vi "TLB Native Dynamic Events ver 0.17e.vi"() -> ()   [LabVIEW 2018]
uses:
  Labview Training Phase 2/Enum Controls/States for Action Engine.ctl
  TLB Type Definitions/State Type Definitions, for 0.26g versions and later 2.ctl
  TLB Type Definitions/Intruction Type Definitions.ctl
  TLB Type Definitions/Encoder cluster.ctl
  TLB Type Definitions/PING CLUSTER.ctl
  <vilib>/Studica/Studica Toolkit/NavX/NavX.lvlib
  <vilib>/Studica/Studica Toolkit/Background/DIO Channel.ctl
  Underlying VI's/NavX VI/navX type def.ctl
  <vilib>/Studica/Studica Toolkit/Background/I2C Channel.ctl
  TLB Type Definitions/Vision cluster.ctl
  <vilib>/NI_Real-Time Target Support.lvlib
  TLB Type Definitions/Stepper cluster.ctl
  Experimental VI's/Archived VI's/MOTOR CONTROL NO PID Type Def.ctl
  Underlying VI's/I2C Master VI/I2C MASTER Type Def.ctl
  Underlying VI's/I2C Master VI/I2C_MASTER_WRITE_NEW Type Def.ctl
  <vilib>/userdefined/High Color/IMAQdx.ctl
  Underlying VI's/I2C Master VI/Arduino_Interfacing.ctl
  TLB Type Definitions/Yaw Cluster.ctl
  TLB Type Definitions/Time cluster.ctl
  TLB Type Definitions/Y Stepper cluster.ctl
  Underlying VI's/Modified webcam FGV/Webcam AE.ctl
  Underlying VI's/Elasped Timer/Elapsed timer control.ctl
  Underlying VI's/Motor Control VI with PID/MOTOR CONTROL WITH PID AE DATA MODE TYPE DEF.ctl
  Underlying VI's/Motor Control VI with PID/MOTOR CONTROL WITH PID AE DIRECTION TYPE DEF.ctl
  TLB Type Definitions/IR Sensor Type Def.ctl
  <vilib>/myRIO/Common/Instrument Driver Framework/myRIO v1.0/AI/typedefs/AI Channels Enum.ctl
  <vilib>/myRIO/Common/Instrument Driver Framework/myRIO v1.0/AI/typedefs/AI Channels List.ctl
  <vilib>/Utility/RT CPU Load.ctl
panel:
  out "Left IR Sensor":dbl
  out "Obstacle detected":bool
  out "Speed & distance":T1
  out "Object Center Coordinates":cluster{"x":sgl, "y":sgl}
  out "Object detection cluster":T2
  out "Time up flag":bool
  out "Task selection":u8
  in  "Object recognition mode":enum16{"Ball", "Soap", "Gel", "Pipe", "None"}(ring)
  out "NavX Readings":T3
  out "Arduino Data":T4
  out "CPU loads":T5[](array[typedef]) {"ISR (%)" format="%#.2f"; "Idle (%)" format="%#.2f"; "Background (%)" format="%#.2f"; "Normal (%)" format="%#.2f"; "Above Normal (%)" format="%#.2f"; "High (%)" format="%#.2g"; "Timed Structures (%)" format="%#.2g"; "Time Critical (%)" format="%#.2g"; "Total (%)" format="%#.2g"}
  out "TASK ENABLE":bool
  out "Rising Edge":bool
  in  "Green LED":bool
  out "I2C Error":errorcluster
  out "State Logic":T6=enum."Startup"
  out "elements":T7[](array[typedef])
  in  "STOP TASK":bool
  in  "OK Button":bool
  in  "STOP":bool
  out "error out":errorcluster
  out "Action Queue Items":i32
  out "State Logic Queue Items":i32
  out "Action Queues items":string[](array[string])=["Hardware reset", "Software reset", ""]
  out "Action State":string
  # "System Health Status Update"
  # "VISION"
  # "TLB FRAMEWORK STATUS"
  # "Test Programme written by Calvin Loke    Dated: 28 Aug 2019\nTest Programme revised by Dr Alex See   Dated 30 Aug 2019\n\nRevision date: 20/03/2020\nProgramme version:   TLB Native Dynamic Events ver 0.14a"
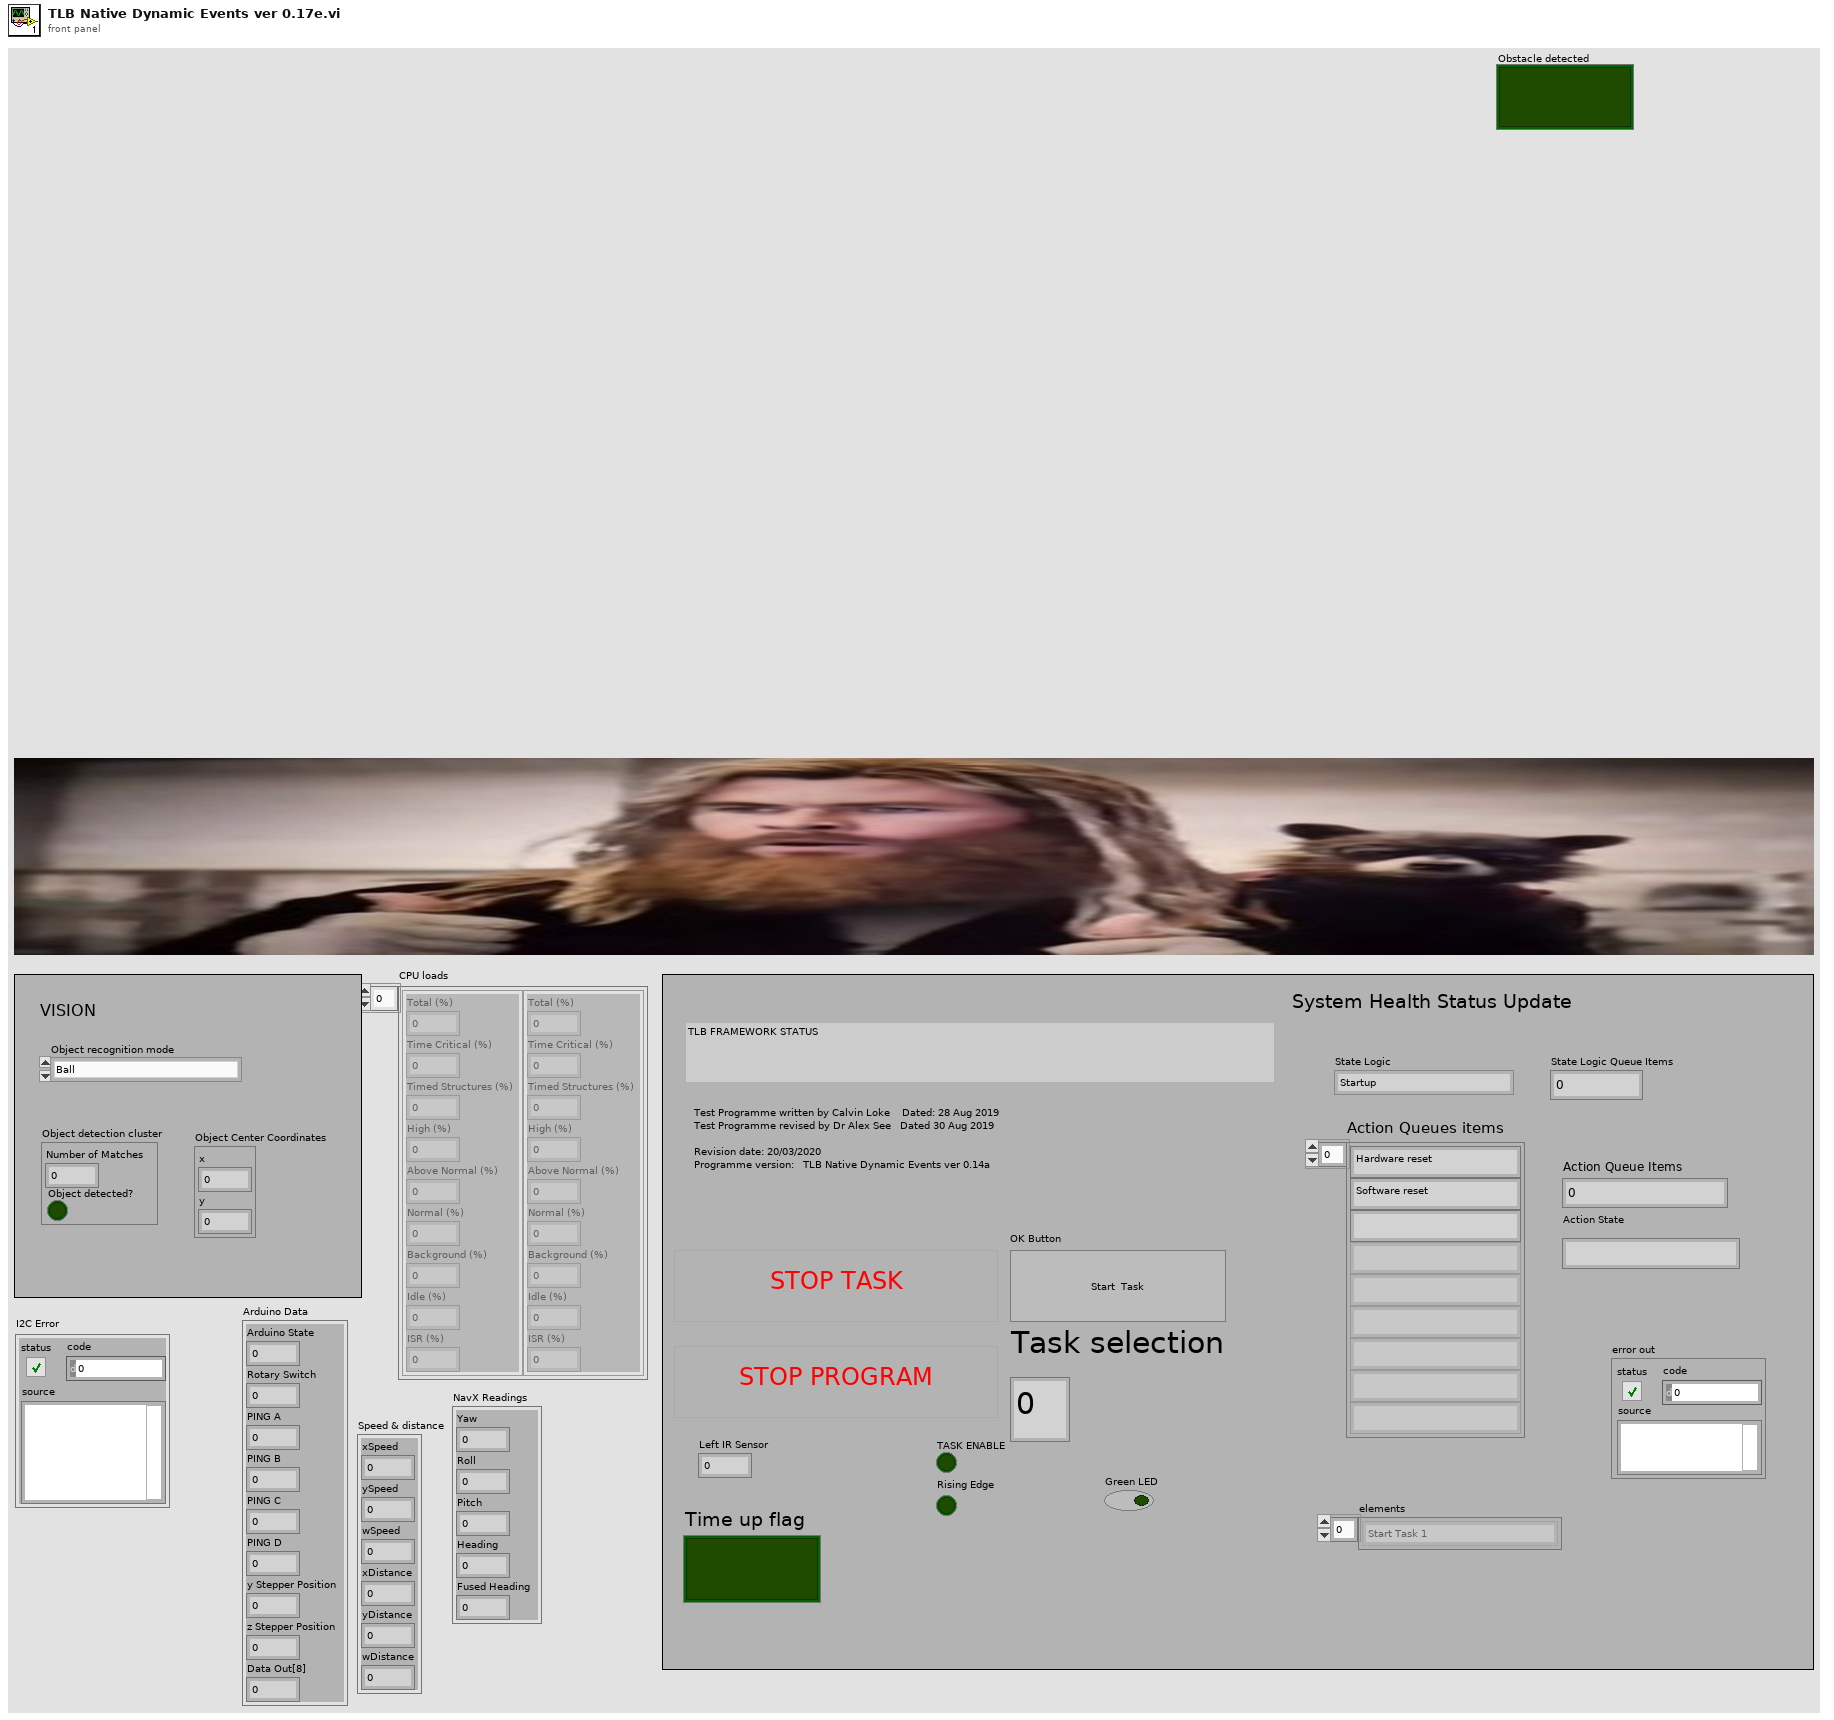
[diagram p1: front panel]
types:
  T1 = cluster{"xSpeed":dbl, "ySpeed":dbl, "wSpeed":dbl, "xDistance":dbl, "yDistance":dbl, "wDistance":dbl}
  T2 = cluster{"Number of Matches":i32, "Object detected?":bool}
  T3 = cluster{"Yaw":dbl, "Roll":dbl, "Pitch":dbl, "Heading":dbl, "Fused Heading":dbl}
  T4 = cluster{"Arduino State":u8, "Rotary Switch":u8, "PING A":u8, "PING B":u8, "PING C":u8, "PING D":u8, "y Stepper Position":u8, "z Stepper Position":u8, "Data Out[8]":u8}
  T5 = typedef "NI_Real-Time Target Support.lvlib/RT CPU Load.ctl" = cluster{"Total (%)":dbl, "Time Critical (%)":dbl, "Timed Structures (%)":dbl, "High (%)":dbl, "Above Normal (%)":dbl, "Normal (%)":dbl, "Background (%)":dbl, "Idle (%)":dbl, "ISR (%)":dbl}
  T6 = typedef "State Type Definitions, for 0.26g versions and later 2.ctl" = enum16{"None", "Startup", "Move to Angle", "True Stop", "Idle", "Shutdown", "Task 1A", "Task 1B", "Task 2:Raise Arm", "Task 2:Sensor Mode", "Task 2:Reverse Mode", "Task 3", "Task 4_A", "Task 4_B", "Task 4_C", "Task 4_D", "Task 5A", "Task 5B", "Task 5C", "Task 5D", "Task 5E: POSITION ARM", "Task 5F: ARM GRAB HEIGHT", "Task 5G: CLOSE CLAW", "Task 5H: RAISE ARM", "Task 6_A", "Task 6_B", "Task 7", "Task 8A: RAISE ARM", "Task 8B: MOVE TO BOX", "Task 8C: CAM BURST", "Task 8D: PROCESS IMAGE", "Task 8E: ROBOT ADJUST", "Task 8F: CAM BURST 2", "Task 8G: PROCESS IMAGE 2", "Task 8H: ARM ADJUST", "Task 8I: ARM GRAB HEIGHT", "Task 8J: CLOSE CLAW", "Task 8K: RAISE MY SWORD", "Task 9A: Raise Arm", "Task 9B: Rotate to Angle", "Task 9C: Detect Box", "Task 9D: MOVE FORWARD", "Task 9E: MOVE LEFT", "Task 9F: SCAN BOX", "Task 9G: MOVE RIGHT", "Task 9H: SCAN BOX 2", "Task 9I: ROTATE 90 CW", "Task 9J: FORWARD", "Task 9K: RAM WALL", "Task 9L: MOVE RIGHT", "Task 9M: SCAN BOX 3", "Task 9M: MOVE RIGHT", "Task 9N: SCAN BOX 4", "PENIS", "PENIS 2", "PENIS 3", "Task 9R: PROCESS COLOUR", "Task A1: Task 9 Open cam", "Task A2: Task 9 Move Arm", "Task A3: Task 9 Set Timer", "Task A4: Tasl 9 Capture images", "Task A5: Task 9 Close camera", "Task A6: Process Colour", "Task A7: Dispose Camera Buffer"}
  T7 = typedef "Intruction Type Definitions.ctl" = enum16{"None", "Start Task 1", "Start Task 2", "Start Task 3", "Start Task 4", "Start Task 5", "Start Task 6", "Start Task 7", "Start Task 8 - BALL", "Start Task 8 - Gel", "Start Task 8 - Pipe", "Start Task 8 - Soap", "Start Task 9", "Start Task A", "Start Task B", "Exit"}
  T8 = typedef "IR Sensor Type Def.ctl" = cluster{"Left IR Sensor":dbl, "Arm IR Sensor":dbl, "Bottom IR Sensor":dbl}
  T9 = typedef "Y Stepper cluster.ctl" = cluster{"yStepper desired":u8}
  T10 = typedef "Time cluster.ctl" = cluster{"Time up flag":bool, "SET TIME TO CHECK":dbl}
  T11 = typedef "Yaw Cluster.ctl" = cluster{"Yaw":dbl, "Compass":dbl}
  T12 = typedef "Stepper cluster.ctl" = cluster{"y Stepper Position":u8, "z Stepper Position":u8}
  T13 = typedef "DIO Channel.ctl" = enum16{"Not Connected", "A/DIO1", "A/DIO2", "A/DIO3", "A/DIO4", "A/DIO5", "A/DIO6", "A/DIO7", "A/DIO13", "B/DIO1", "B/DIO2", "B/DIO3", "B/DIO4", "B/DIO5", "B/DIO6", "B/DIO7", "B/DIO13", "C/DIO0", "C/DIO1", "C/DIO2", "C/DIO3", "C/DIO4", "C/DIO5", "C/DIO6", "C/DIO7"}
  T14 = typedef "Vision cluster.ctl" = cluster{"Recognized Object":bool, "Object X coordinate":dbl, "Object Y coordinate":dbl}
  T15 = typedef "PING CLUSTER.ctl" = cluster{"PING_A":u8, "PING_B":u8, "PING_C":u8, "PING_D":u8}
  T16 = typedef "Encoder cluster.ctl" = cluster{"xDistance":dbl, "yDistance":dbl, "wDistance":dbl}
  T17 = cluster{"DIO Channel":T13, "FPGA VI Reference Out":refnum<k20>}
  T18 = typedef "navX type def.ctl" = enum16{"Get i2C reference", "Read Values", "Zero Yaw"}
  T19 = typedef "Arduino_Interfacing.ctl" = enum16{"Initialize", "Write to Arduino", "Read From Arduino"}
  T20 = typedef "I2C Channel.ctl" = enum16{"Not Connected", "A", "B"}
  T21 = typedef "States for Action Engine.ctl" = enum16{"Initialize", "Write", "Read"}
  T22 = cluster{"I2C Ref Out":cluster{"I2C Channel":T20, "FPGA VI Reference Out":refnum<k20>}, "Connected":bool, "Slave Address (7-bit)":u8, "Registry":u8[]}
  T23 = typedef "Intruction Type Definitions.ctl" = enum16{"None", "Start Task 1", "Start Task 2", "Start Task 3", "Start Task 4", "Start Task 5", "Start Task 6", "Start Task 7", "Start Task 8", "Start Task 9", "Start Task A", "Start Task B", "Exit"}
  T24 = typedef "IMAQ Image.ctl" = refnum<image>
  T25 = typedef "State Type Definitions.ctl" = enum16{"None", "Startup", "Move to Angle", "True Stop", "Idle", "Shutdown", "Task 1", "Task 2:Raise Arm", "Task 2:Sensor Mode", "Task 2:Reverse Mode", "Task 3", "Task 4_A", "Task 4_B", "Task 4_C", "Task 4_D", "Task 5A: ARM CAM HEIGHT", "Task 5B: MOVE TO BOX", "Task 5C: CAM BURST", "Task 5D: PROCESS IMAGE", "Task 5E: POSITION ARM", "Task 5F: ARM GRAB HEIGHT", "Task 5G: CLOSE CLAW", "Task 5H: RAISE ARM", "Task 6_A", "Task 6_B", "Task 7", "Task 8A: RAISE ARM", "Task 8B: MOVE TO BOX", "Task 8C: CAM BURST", "Task 8D: PROCESS IMAGE", "Task 8E: ROBOT ADJUST", "Task 9A: Raise Arm", "Task 9B: Rotate to Angle", "Task 9C: Rotation alignmnet", "Task B"}
  T26 = typedef "MOTOR CONTROL WITH PID AE DIRECTION TYPE DEF.ctl" = enum16{"y-axis movement", "x-axis movement", "rotation", "stop", "reset encoders"}
  T27 = typedef "MOTOR CONTROL WITH PID AE DATA MODE TYPE DEF.ctl" = enum16{"Init AE", "Write to AE", "Read from AE"}
  T28 = typedef "Elapsed timer control.ctl" = enum16{"Start", "Pause", "Initialize"}
  T29 = typedef "I2C_MASTER_WRITE_NEW Type Def.ctl" = enum16{"Ultrasonic sensors", "Stepper origin", "zStepper 13.3k", "zStepper 13k", "zStepper 12k", "zStepper 11k", "zStepper 10k", "zStepper 9k", "zStepper 8k", "zStepper 7k", "zStepper 6k", "zStepper 5k", "zStepper 4k", "zStepper 3k", "zStepper 2k", "zStepper 1k", "zStepper 900", "zStepper 800", "zStepper 700", "zStepper 600", "zStepper 500", "zStepper 400", "zStepper 300", "zStepper 200", "zStepper 100", "zStepper 0", "yStepper control", "Open Claw", "Close Claw", "Soft Reset"}
  T30 = typedef "Webcam AE.ctl" = enum16{"Initialize Camera", "Open Camera", "Continuous Acquisition", "Close Camera", "Retrieve Image", "Dispose Camera Image Buffer"}
  T31 = typedef "IMAQdx.ctl" = refnum<k21>
  T32 = typedef "Webcam AE.ctl" = enum16{"Initialize Camera", "Open Camera", "Continuous Acquisition", "Close Camera", "Retrieve Image", "Dispose Image Buffers"}
  T33 = typedef "MOTOR CONTROL NO PID Type Def.ctl" = enum16{"Init", "Front Back", "Left Right", "Rotate", "Stop", "Latch"}
  T34 = typedef "AI Channels List.ctl" = T35[]
  T35 = typedef "AI Channels Enum.ctl" = enum16{"Not Connected", "AudioIn/Left", "AudioIn/Right", "C/AI0", "C/AI1", "A/AI0", "A/AI1", "A/AI2", "A/AI3", "A/AI4", "A/AI5", "A/AI6", "A/AI7", "B/AI0", "B/AI1", "B/AI2", "B/AI3", "B/AI4", "B/AI5", "B/AI6", "B/AI7", "AI/AI0", "AI/AI1", "AI/AI2", "AI/AI3", "A/AI0 (DIFF)", "A/AI1 (DIFF)", "A/AI2 (DIFF)", "A/AI3 (DIFF)", "B/AI0 (DIFF)", "B/AI1 (DIFF)", "B/AI2 (DIFF)", "B/AI3 (DIFF)"}
  T36 = typedef "I2C MASTER Type Def.ctl" = enum16{"Last State", "Mode 0", "Mode 1", "Mode 2", "Mode 3", "Mode 4", "Mode 5", "Mode 6", "Mode 7", "Mode 8", "Mode 9", "Mode 10"}
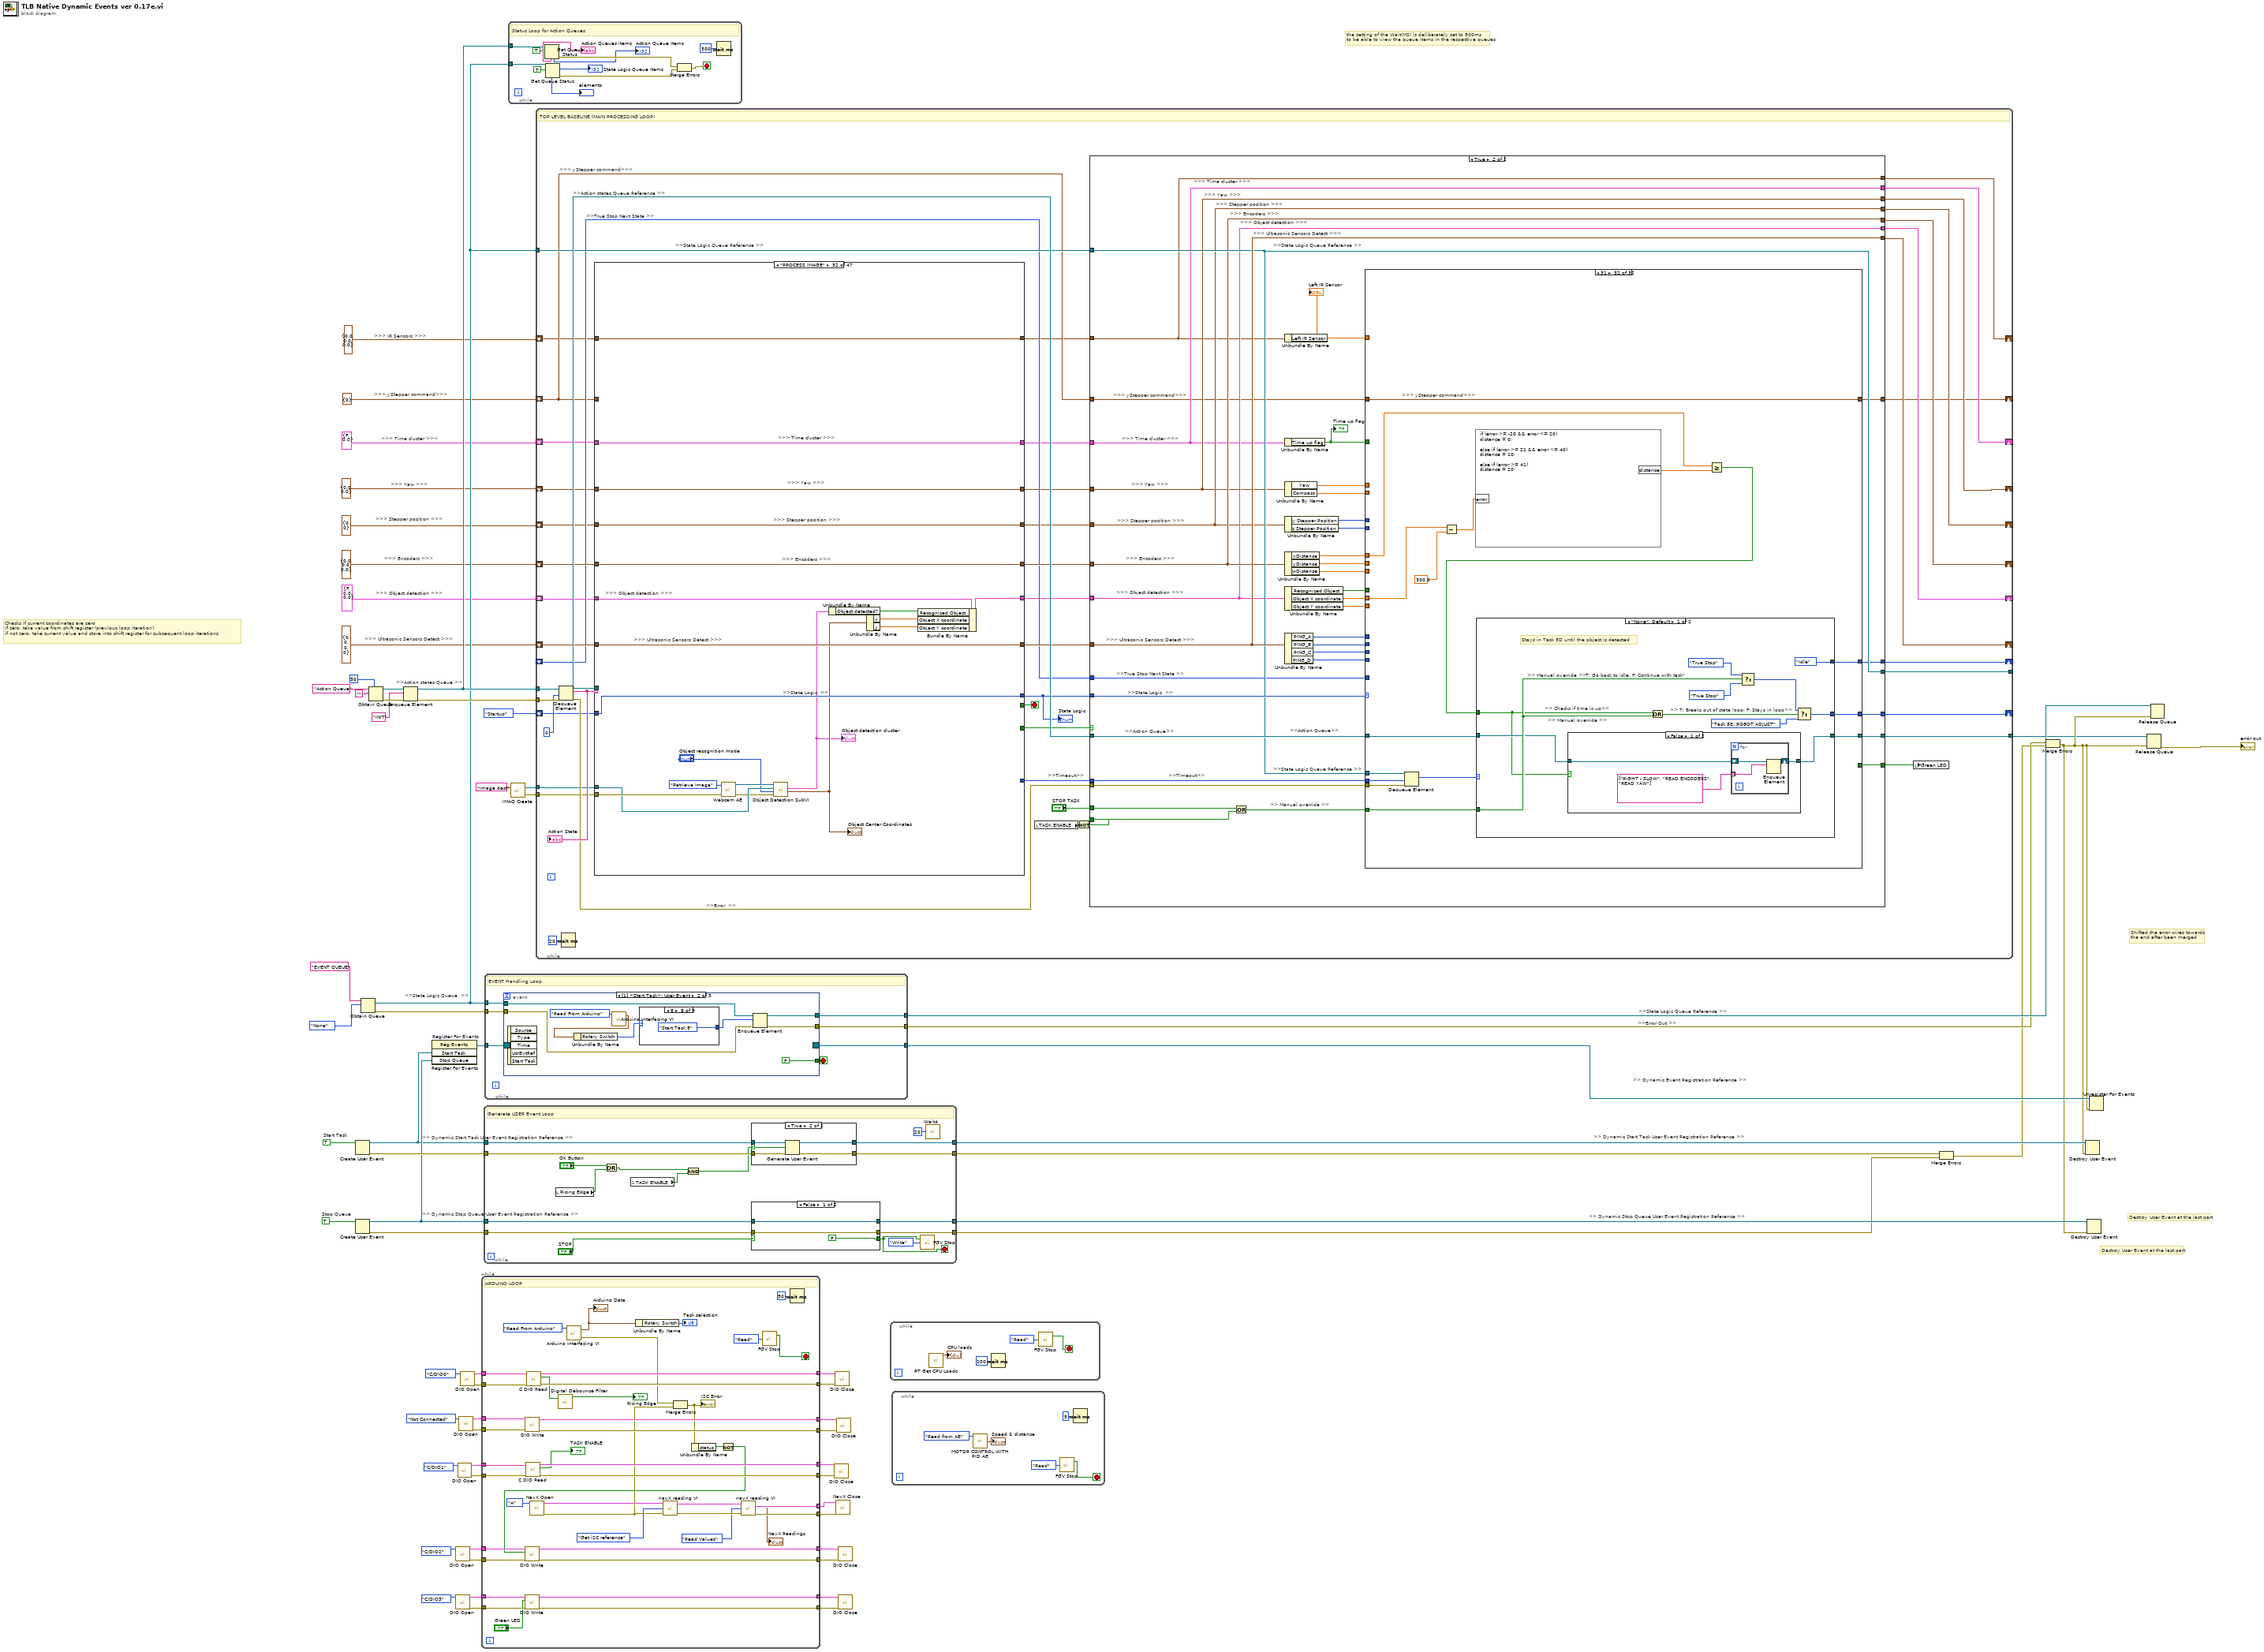
[diagram p0: block diagram]
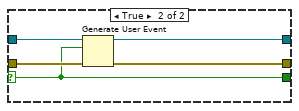
[diagram p2: hidden frame]
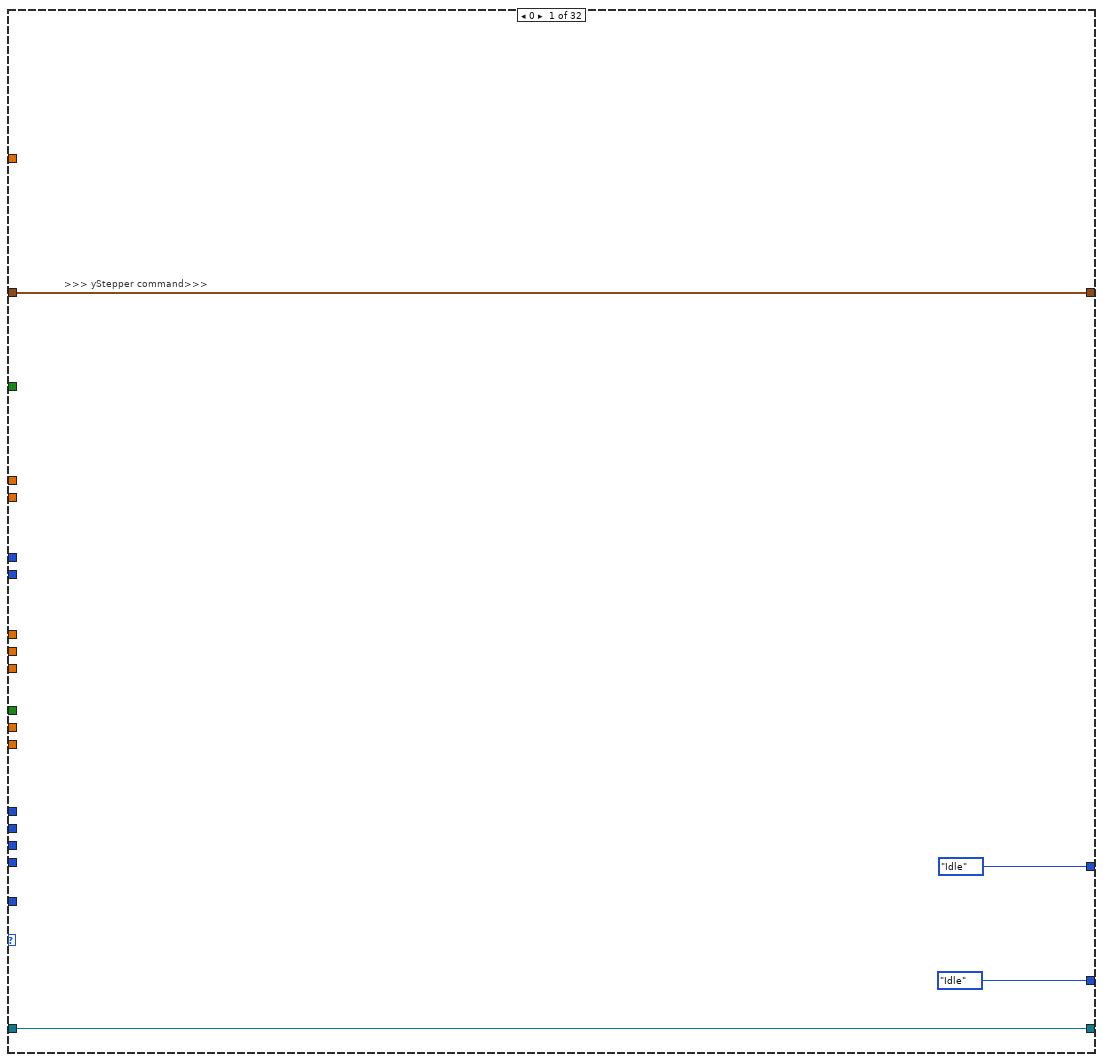
[diagram p5: hidden frame]
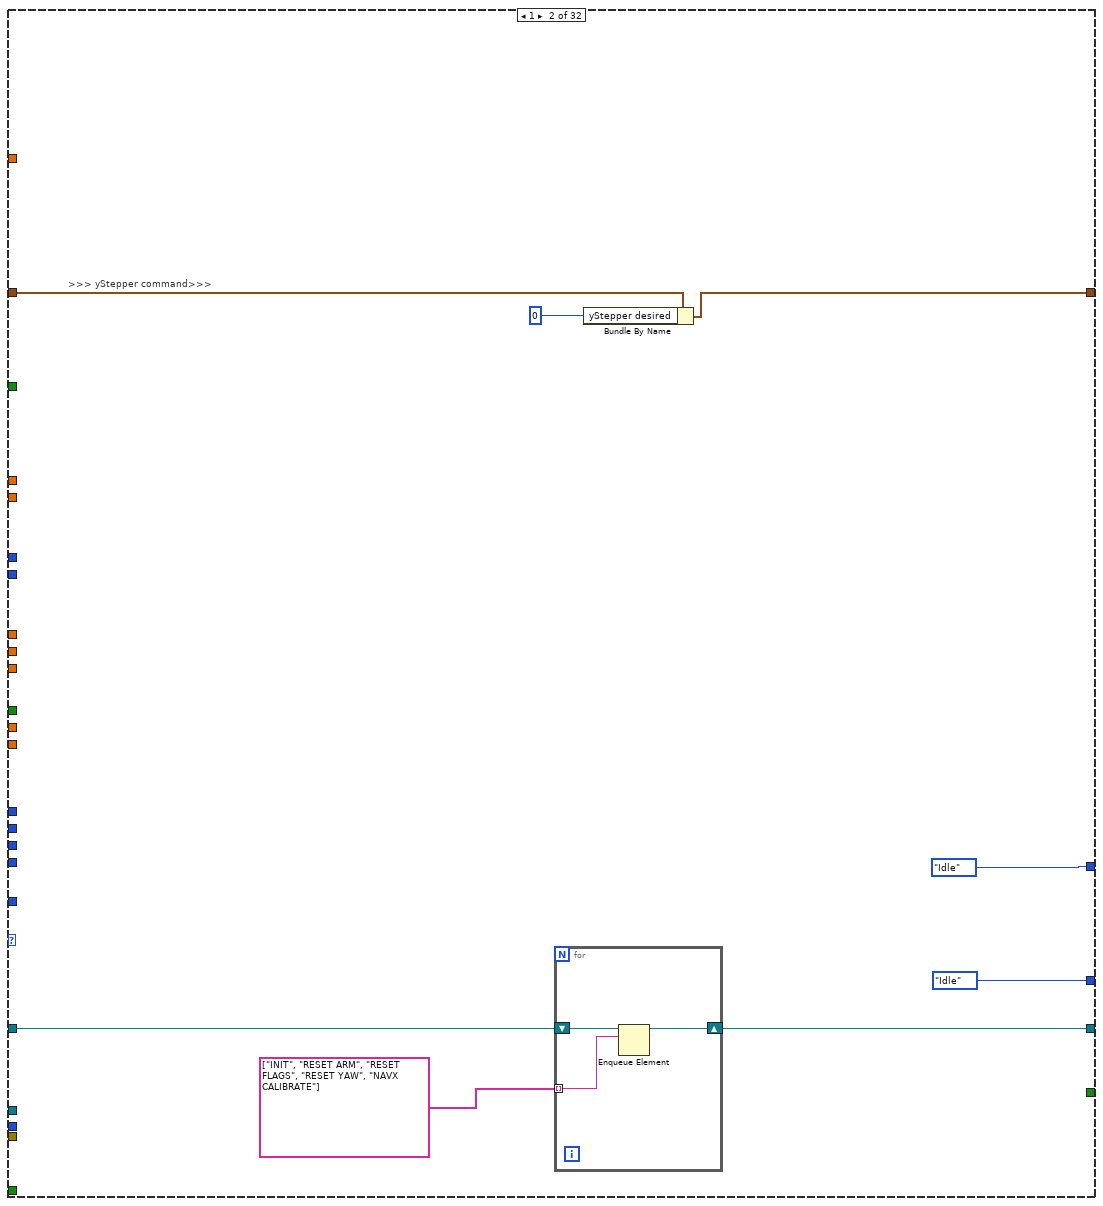
[diagram p6: hidden frame]
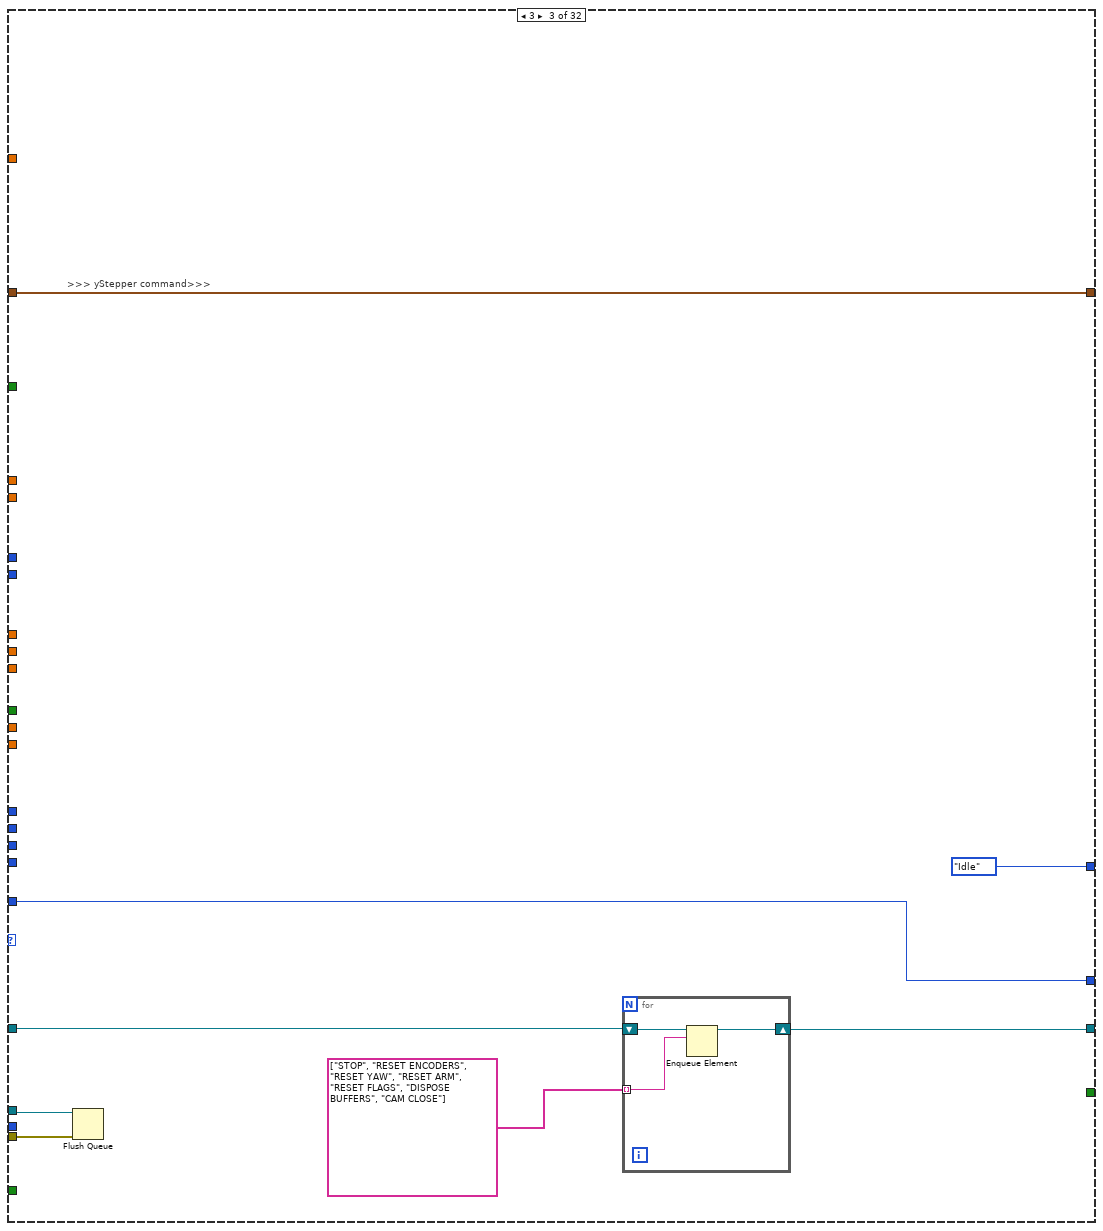
[diagram p7: hidden frame]
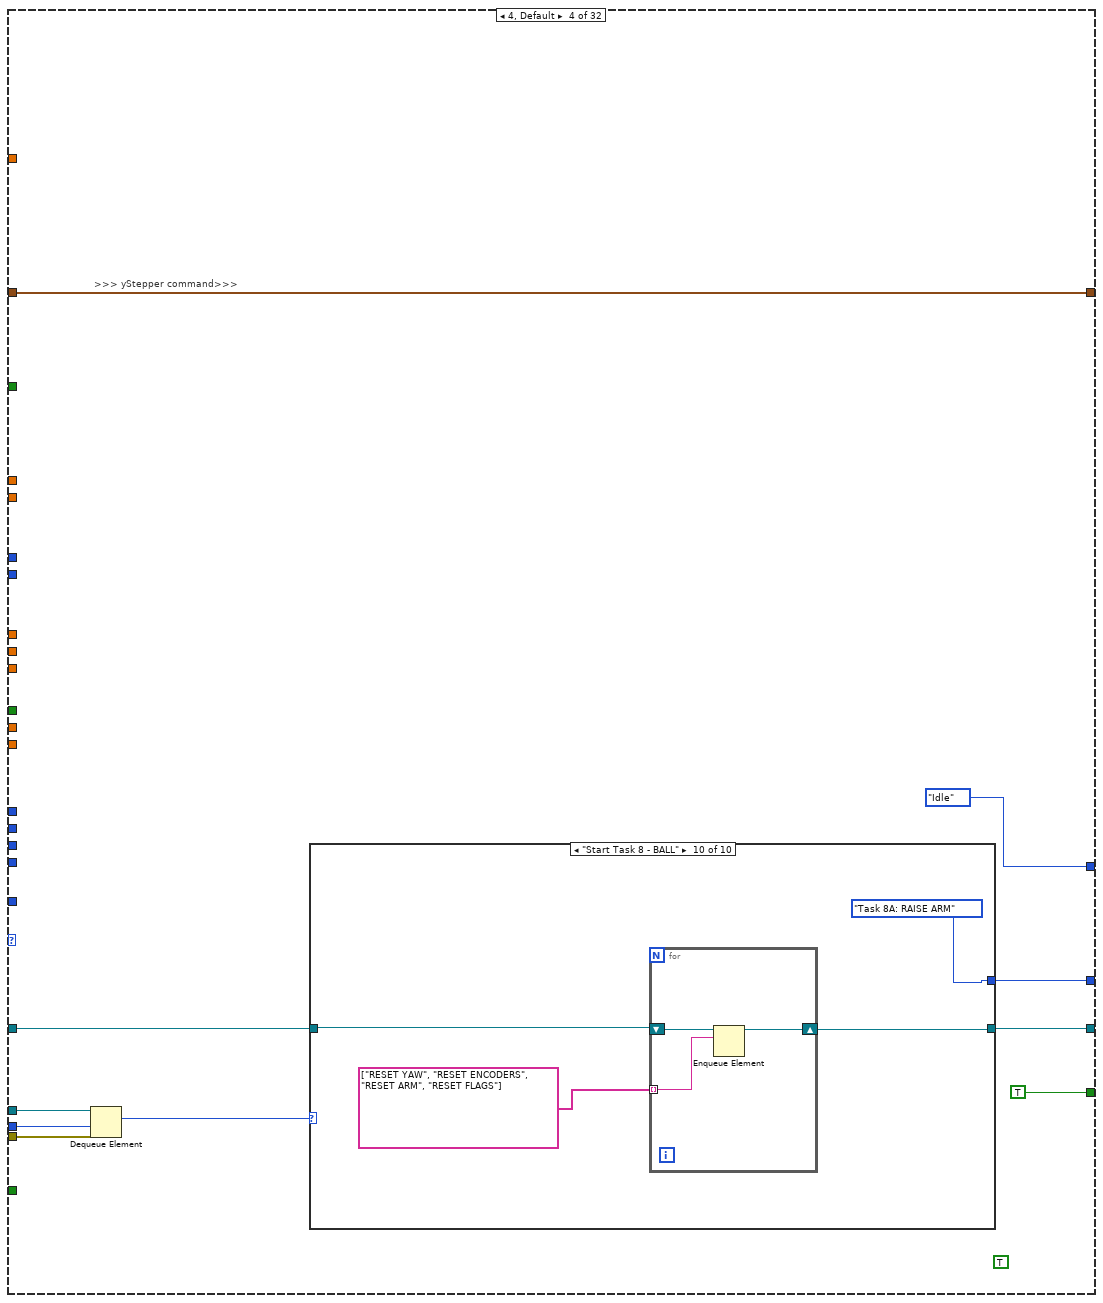
[diagram p8: hidden frame]
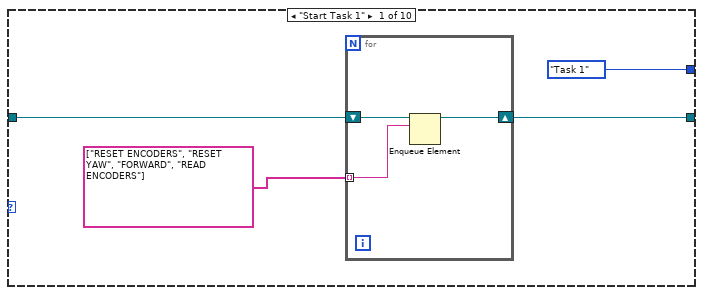
[diagram p9: hidden frame]
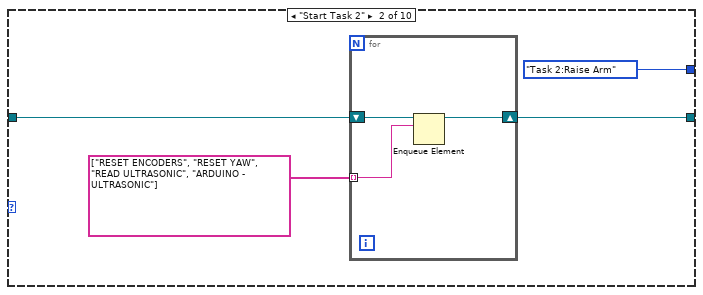
[diagram p10: hidden frame]
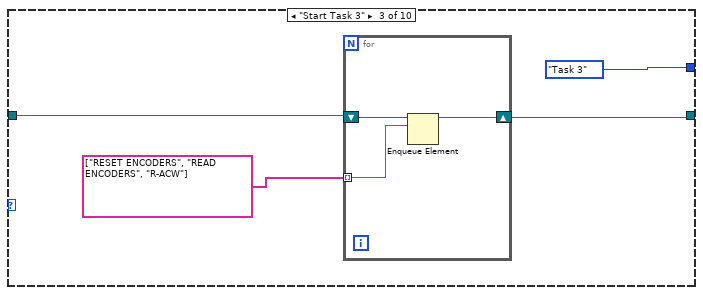
[diagram p11: hidden frame]
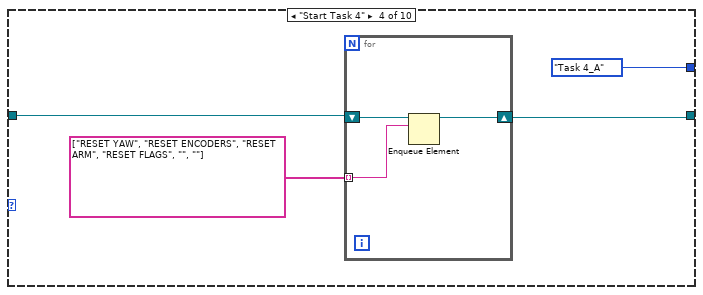
[diagram p12: hidden frame]
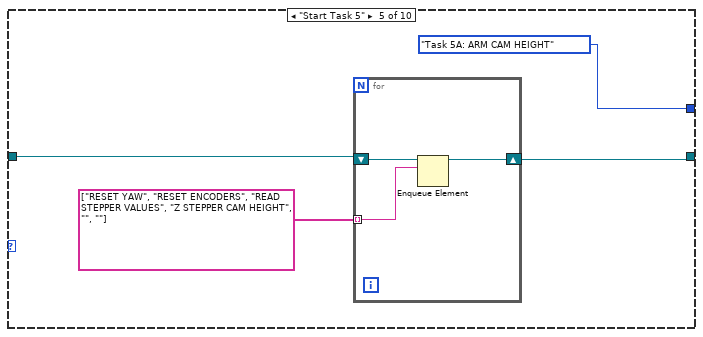
[diagram p13: hidden frame]
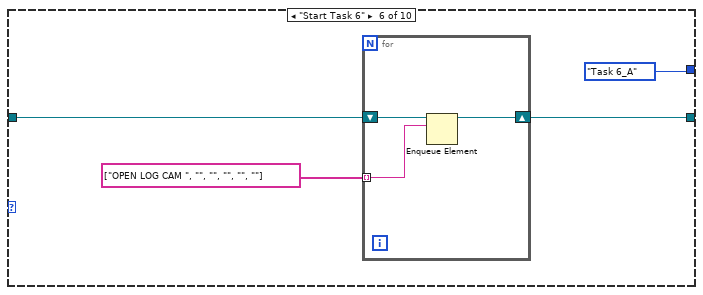
[diagram p14: hidden frame]
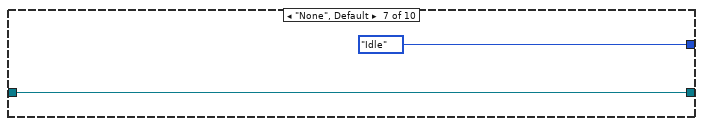
[diagram p15: hidden frame]
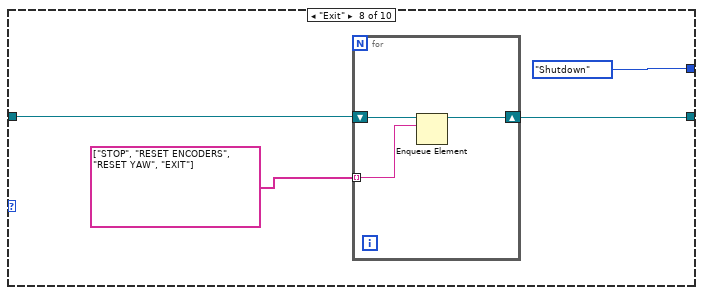
[diagram p16: hidden frame]
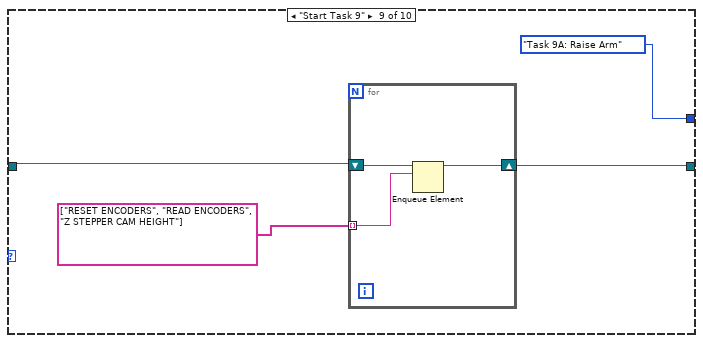
[diagram p17: hidden frame]
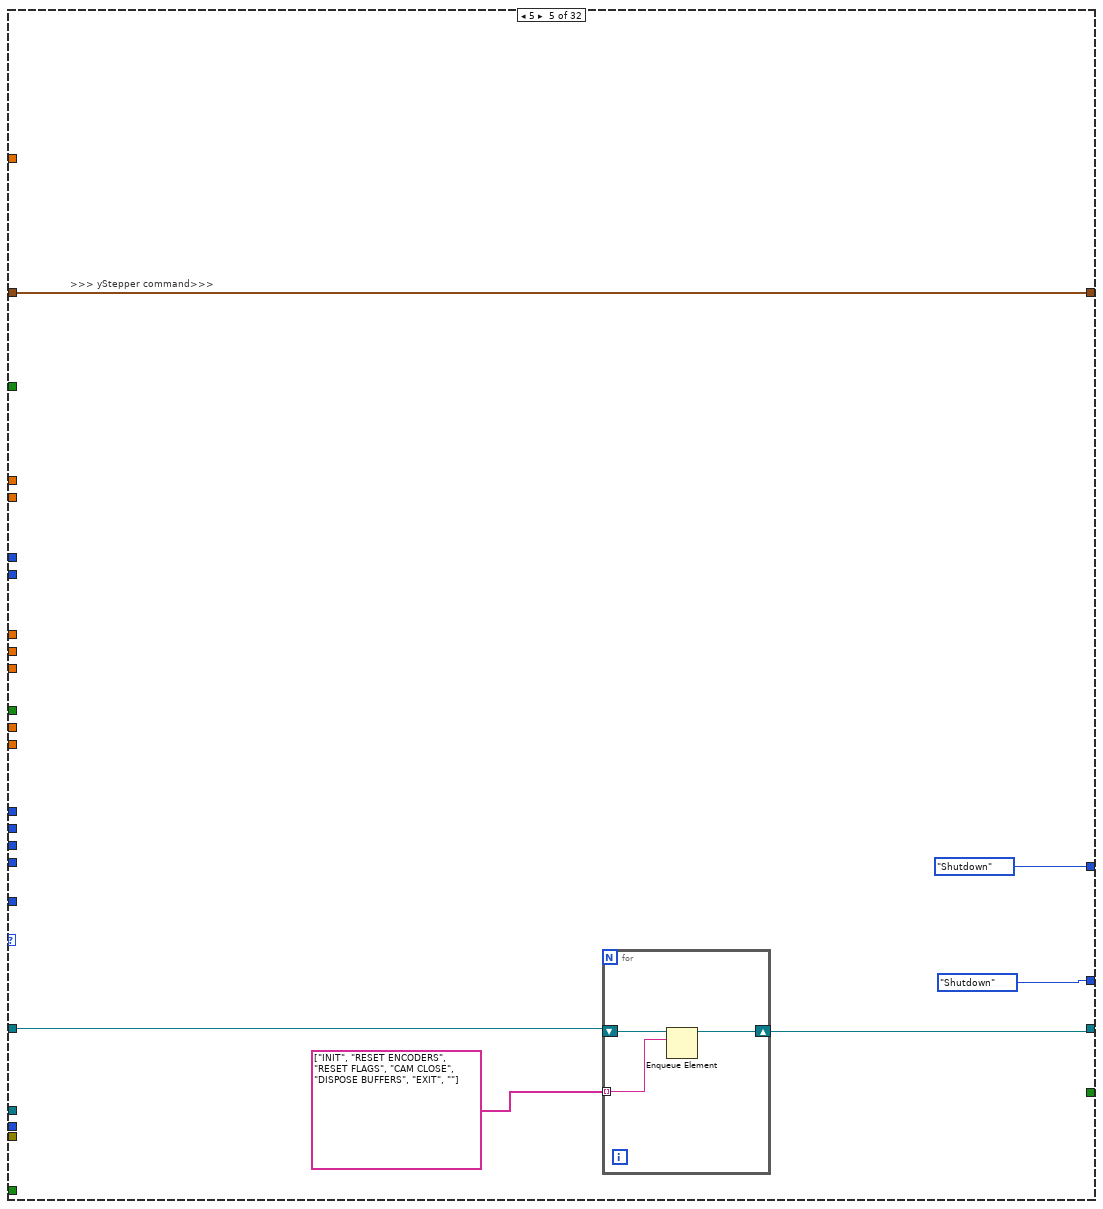
[diagram p18: hidden frame]
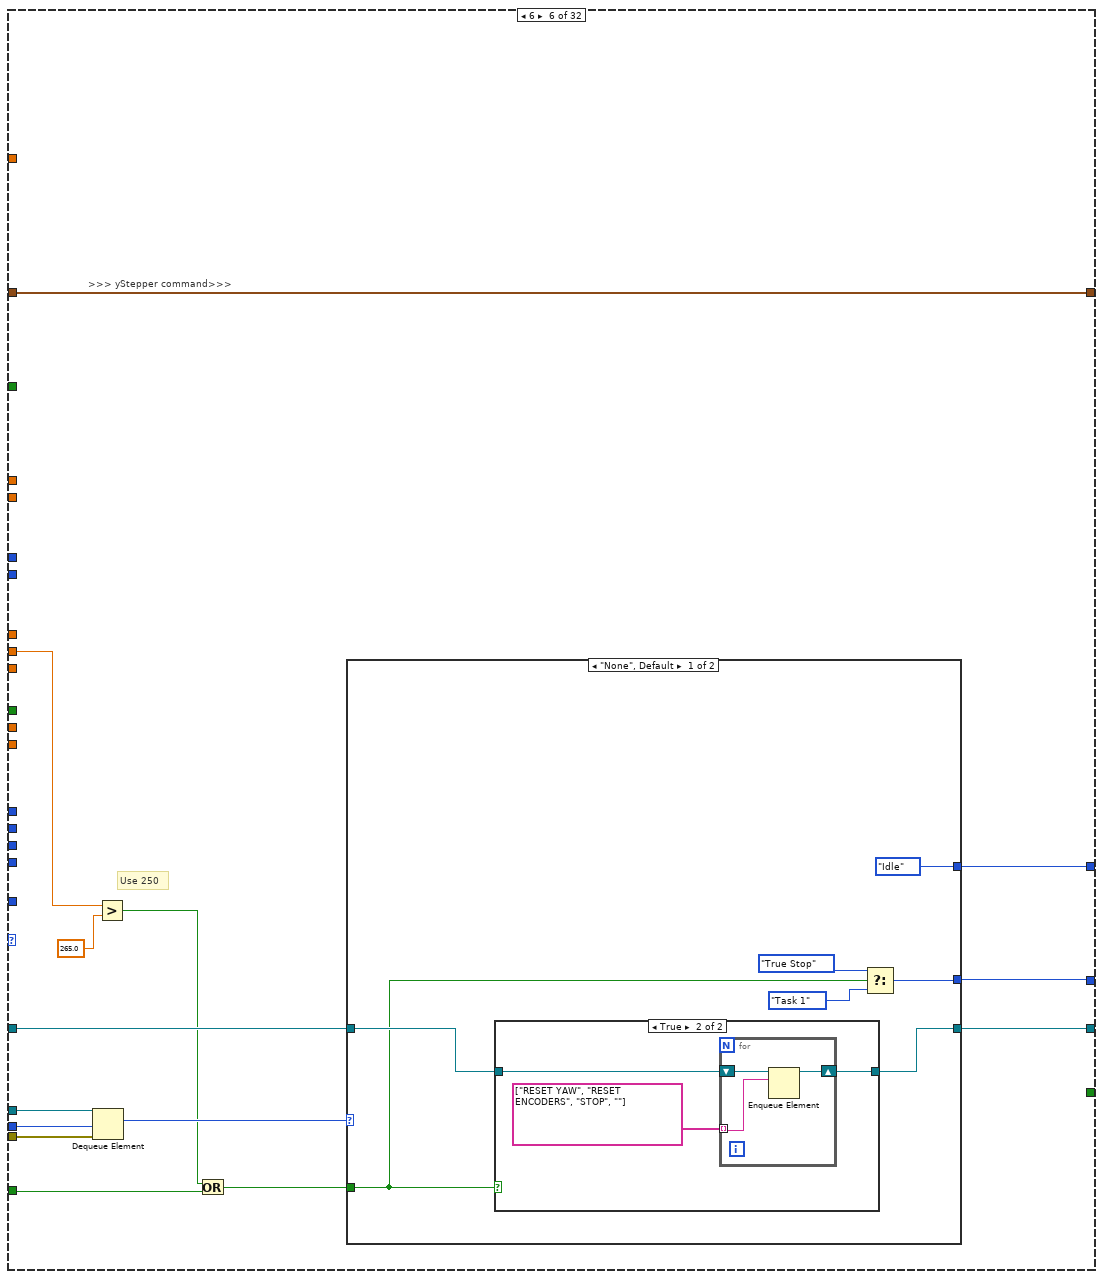
[diagram p19: hidden frame]
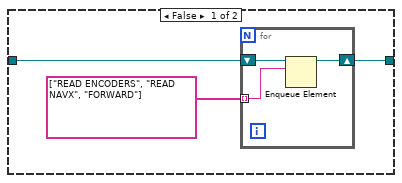
[diagram p20: hidden frame]
diagram:
  w69 = TRUE  # Stop Queue
  w68 = TRUE  # Start Task
  # ">>> IR Sensors >>>"
  # "Checks if current coordinates are zero\nif zero, take value from shift register (previous loop iteration)\nif not zero, take current value and store into shift register for subsequent loop iterations"
  # ">>> yStepper command>>>"
  # ">>> Time cluster >>>"
  # ">>> Yaw >>>"
  # ">>> Stepper position >>>"
  # ">>> Encoders >>>"
  # ">>> Object detection >>>"
  # ">>> Ultrasonic Sensors Detect >>>"
  # "the setting of the Wait(MS) is deliberately set to 500ms\nto be able to view the queue items in the respective queues"
  # ">>Error Out >>"
  # ">> Dynamic Stop Queue User Event Registration Reference >>"
  # ">> Dynamic Start Task User Event Registration Reference >>"
  # ">> Dynamic Stop Queue User Event Registration Reference >>"
  # ">> Dynamic Start Task User Event Registration Reference >>"
  # ">> Dynamic Event Registration Reference >>"
  # ">>Action states Queue >>"
  # ">>State Logic Queue  >>"
  # ">>State Logic Queue Reference >>"
  # "Destroy User Event at the last part"
  # "Destroy User Event at the last part"
  # "Shifted the error wires towards\nthe end after been merged"
  n1 = Create User Event(user event datatype=w68) -> (user event=w60:refnum<user-event>, error out=w65:errorcluster)  [unwired: 1 in]
  n2 = Create User Event(user event datatype=w69) -> (user event=w61:refnum<user-event>, error out=w64:errorcluster)  [unwired: 1 in]
  n3 = Obtain Queue(name (unnamed)="EVENT QUEUE", element data type=Intruction_Type_Definitions."None" ("Enum")) -> (queue out=w46:refnum<queue>, error out=w52:errorcluster)  [unwired: 3 in, 1 out]
  n4 = Obtain Queue(max queue size (-1, unlimited)=50, name (unnamed)="Action Queue", element data type="") -> (queue out=w55:refnum<queue>, error out=w51:errorcluster)  [unwired: 2 in, 1 out]
  n5 = Enqueue Element(queue=w55, element="INIT", error in (no error)=w51) -> (queue out=w47:refnum<queue>, error out=w50:errorcluster)  [unwired: 1 in, 1 out]
  n6 = register-events "Register For Events"(w60, w61) -> (reference out=w59:refnum<event-registration>)  [unwired: 2 in, 1 out]
  n7 = call <vilib>:"DIO Open.vi"("DIO Channel"=DIO_Channel."C/DIO2") -> ("error out"=w16:errorcluster, "DIO Info Out"=w17:T17)  [unwired: 9 in]
  n8 = call <vilib>:"DIO Open.vi"("DIO Channel"=DIO_Channel."C/DIO3") -> ("error out"=w11:errorcluster, "DIO Info Out"=w12:T17)  [unwired: 9 in]
  n9 = call <vilib>:"DIO Open.vi"("DIO Channel"=DIO_Channel."C/DIO1") -> ("error out"=w24:errorcluster, "DIO Info Out"=w25:T17)  [unwired: 9 in]
  n10 = call <vilib>:"DIO Open.vi"("DIO Channel"=DIO_Channel."Not Connected") -> ("error out"=w29:errorcluster, "DIO Info Out"=w31:T17)  [unwired: 9 in]
  n11 = call <vilib>:"DIO Open.vi"("DIO Channel"=DIO_Channel."C/DIO0") -> ("error out"=w34:errorcluster, "DIO Info Out"=w37:T17)  [unwired: 9 in]
  n12 = while {
    tunnel: w37 -> [w110]
    tunnel: [w109] -> w35
    tunnel: w34 -> [w108]
    tunnel: [w107] -> w33
    tunnel: w31 -> [w104]
    tunnel: [w103] -> w30
    tunnel: w29 -> [w102]
    tunnel: [w101] -> w28
    tunnel: [w100] -> w26
    tunnel: w25 -> [w99]
    tunnel: w24 -> [w98]
    tunnel: [w97] -> w23
    tunnel: w17 -> [w91]
    tunnel: w16 -> [w90]
    tunnel: [w89] -> w15
    tunnel: [w88] -> w14
    tunnel: w12 -> [w87]
    tunnel: w11 -> [w86]
    tunnel: [w85] -> w10
    tunnel: [w84] -> w9
    tunnel: [w78] -> w6
    tunnel: [w77] -> w7
    stop <- w112 stop-if-true
    # "ARDUINO LOOP"
    n13 = call <vilib>:"DIO Write.vi"("error in (no error)"=w86, "Input"="Green LED", "DIO Info In"=w87) -> ("error out"=w84:errorcluster, "DIO Info Out"=w85:T17)  [unwired: 7 in]
    n14 = call <vilib>:"DIO Write.vi"("error in (no error)"=w102, "DIO Info In"=w104) -> ("error out"=w101:errorcluster, "DIO Info Out"=w103:T17)  [unwired: 8 in]
    n15 = call <vilib>:"C DIO Read.vi"("error in (no error)"=w98, "DIO Info In in"=w99) -> ("error out"=w97:errorcluster, "IN"=→"TASK ENABLE":bool, "DIO Info In out"=w100:T17)  [unwired: 7 in]
    n16 = call <vilib>:"C DIO Read.vi"("error in (no error)"=w108, "DIO Info In in"=w110) -> ("error out"=w107:errorcluster, "IN"=w106:bool, "DIO Info In out"=w109:T17)  [unwired: 7 in]
    n17 = call <vilib>:"NavX Open.vi"("I2C Channel"=I2C_Channel."A") -> ("error out"=w93:errorcluster, "NavX Info"=w95:T22)  [unwired: 9 in]
    n18 = call "Digital Debounce Filter.vi"("Boolean input"=w106) -> ("Rising Edge"=→"Rising Edge":bool)  [unwired: 1 in, 2 out]
    n19 = call "Arduino Interfacing VI.vi"("AE Mode"=Arduino_Interfacing."Read From Arduino") -> ("error out"=w81:errorcluster, "Arduino Data"=w74:T4)  [unwired: 3 in]
    "Arduino Data" <- w74
    n20 = Unbundle By Name(w74) -> ("Rotary Switch"=→"Task selection":u8)
    n21 = call "navX reading VI.vi"("NavX Info In"=w95, "Mode"=navX_type_def."Get i2C reference", "error in (no error)"=w93) -> ("NavX Info Out"=w80:T22, "Error Out"=w79:errorcluster)  [unwired: 2 out]
    n22 = Merge Errors(w81, w93) -> (w72:errorcluster)
    "I2C Error" <- w72
    n23 = Unbundle By Name(w72) -> ("status"=w71:bool)
    n24 = Not(x=w71) -> (.not. x?=w70:bool)
    n25 = call <vilib>:"DIO Write.vi"("error in (no error)"=w90, "Input"=w70, "DIO Info In"=w91) -> ("error out"=w88:errorcluster, "DIO Info Out"=w89:T17)  [unwired: 7 in]
    n26 = call "navX reading VI.vi"("NavX Info In"=w80, "Mode"=navX_type_def."Read Values", "error in (no error)"=w79) -> ("NavX Info Out"=w78:T22, "NavX Readings"=→"NavX Readings":T3, "Error Out"=w77:errorcluster)  [unwired: 1 out]
    n27 = call "FGV Stop.vi"("Init/Read/Write State"=States_for_Action_Engine."Read") -> ("Output node"=w112:bool)  [unwired: 2 in, 1 out]
    n28 = Wait (ms)(milliseconds to wait=u32 50) -> ()  [unwired: 1 out]
  }
  n29 = while {
    tunnel: w60 -> [w130]
    tunnel: w61 -> [w129]
    tunnel: [w128] -> w67
    tunnel: [w127] -> w66
    tunnel: w65 -> [w126]
    tunnel: [w125] -> w63
    tunnel: w64 -> [w124]
    tunnel: [w123] -> w62
    stop <- w121 stop-if-true
    # "Generate USER Event Loop"
    n30 = local read "Rising Edge"() -> (w117:bool)
    n31 = Or(x="OK Button", y=w117) -> (x .or. y?=w116:bool)
    n32 = local read "TASK ENABLE"() -> (w115:bool)
    n33 = And(x=w116, y=w115) -> (x .and. y?=w114:bool)
    n34 = case shown="True" w114 {
      selector: w114 -> [_ w141]
      tunnel: w130 -> [w140 w145]
      tunnel: [w140 w144] -> w127
      tunnel: w126 -> [w139 w143]
      tunnel: [w139 w142] -> w125
      frame False {
      }
      frame True {
        n35 = Generate User Event(user event=w145, event data cluster=w141, error in=w143) -> (user event out=w144:refnum<user-event>, error out=w142:errorcluster)  [unwired: 1 in]
      }
    }
    n36 = case shown="False" "STOP" {
      selector: "STOP" -> [_ w134]
      tunnel: w129 -> [w133 w138]
      tunnel: [w133 w137] -> w128
      tunnel: w124 -> [w132 w136]
      tunnel: [w132 w135] -> w123
      tunnel: [FALSE w134] -> w121
      frame False {
      }
      frame True {
        n37 = Generate User Event(user event=w138, event data cluster=w134, error in=w136) -> (user event out=w137:refnum<user-event>, error out=w135:errorcluster)  [unwired: 1 in]
      }
    }
    n38 = call "FGV Stop.vi"("Init/Read/Write State"=States_for_Action_Engine."Write", "Input Node"=w121) -> ()  [unwired: 1 in, 2 out]
    n39 = call "Wait4"("Count(uSec)"=u32 20) -> ()  [unwired: 1 out]
  }
  n40 = while {
    tunnel: w59 -> [w152]
    tunnel: [w151] -> w58
    tunnel: w46 -> [w149]
    tunnel: [w148] -> w57
    tunnel: w52 -> [w147]
    tunnel: [w146] -> w49
    stop <- w150 stop-if-true
    # "EVENT Handling Loop"
    n41 = event shown="[1] <Start Task>: User Event" {
      selector: w152 -> [_ _ _]
      dyn-events: [_ _ _] -> w151
      timeout: _ -> [_ _ _]
      tunnel: [FALSE FALSE w182] -> w150
      tunnel: w149 -> [w157 w166 w180]
      tunnel: [w156 w165 w181] -> w148
      tunnel: w147 -> [w155 w164 w179]
      tunnel: [w154 w163 w178] -> w146
      event Timeout {
        n42 = event-data() -> ()  [unwired: 1 in, 3 out]
        n43 = Enqueue Element(queue=w157, element=Intruction_Type_Definitions."None" ("Enum"), error in (no error)=w155) -> (queue out=w156:refnum<queue>, error out=w154:errorcluster)  [unwired: 1 in, 1 out]
      }
      event User Event {
        n44 = event-data() -> ()  [unwired: 1 in, 5 out]
        n45 = call "Arduino Interfacing VI.vi"("AE Mode"=Arduino_Interfacing."Read From Arduino") -> ("Arduino Data"=w160:T4)  [unwired: 3 in, 1 out]
        n46 = Unbundle By Name(w160) -> ("Rotary Switch"=w159:u8)
        n47 = case shown="8" w159 {
          tunnel: [Intruction_Type_Definitions."None" ("Enum") Intruction_Type_Definitions."Start Task 1" ("Enum") Intruction_Type_Definitions."Start Task 2" ("Enum") Intruction_Type_Definitions."Start Task 3" ("Enum") Intruction_Type_Definitions."Start Task 4" ("Enum") Intruction_Type_Definitions."Start Task 5" ("Enum") Intruction_Type_Definitions."Start Task 6" ("Enum") Intruction_Type_Definitions."Start Task 8" ("Enum") Intruction_Type_Definitions."Start Task 9" ("Enum")] -> w162
          frame 0, Default {
          }
          frame 1 {
          }
          frame 2 {
          }
          frame 3 {
          }
          frame 4 {
          }
          frame 5 {
          }
          frame 6 {
          }
          frame 8 {
          }
          frame 9 {
          }
        }
        n48 = Enqueue Element(queue=w166, element=w162, error in (no error)=w164) -> (queue out=w165:refnum<queue>, error out=w163:errorcluster)  [unwired: 1 in, 1 out]
      }
      event User Event {
        n49 = event-data() -> ("Stop Queue"=w182:bool)  [unwired: 1 in, 4 out]
        n50 = Enqueue Element At Opposite End(queue=w180, element=Intruction_Type_Definitions."Exit" ("Enum"), error in (no error)=w179) -> (queue out=w181:refnum<queue>, error out=w178:errorcluster)  [unwired: 1 in, 1 out]
      }
    }
  }
  n51 = while {
    tunnel: w47 -> [w192]
    tunnel: w46 -> [w189]
    stop <- w186 stop-if-true
    # "Status Loop for Action Queues"
    n52 = Get Queue Status(queue=w192, return elements? (F)=TRUE) -> (error out=w188:errorcluster, # elements in queue=→"Action Queue Items":i32, elements=→"Action Queues items":string[])  [unwired: 1 in, 5 out]
    n53 = Get Queue Status(queue=w189, return elements? (F)=TRUE) -> (# pending remove=→"State Logic Queue Items":i32, error out=w187:errorcluster, elements=→"elements":T7[])  [unwired: 1 in, 5 out]
    n54 = Merge Errors(w188, w187) -> (w186:errorcluster)
    n55 = Wait (ms)(milliseconds to wait=u32 500) -> ()  [unwired: 1 out]
  }
  n56 = call "IMAQ Create"("Image Name"="Image dest") -> ("New Image"=w21:T24, "error out"=w20:errorcluster)  [unwired: 4 in]
  n57 = while {
    tunnel: w46 -> [w229]
    tunnel: w47 -> [w241]
    tunnel: w50 -> [w239]
    tunnel: [w238] -> _
    tunnel: [w237] -> w40
    shift-right: [w230] -> _
    shift-left: T15 {"PING_A"=0, "PING_B"=0, "PING_C"=0, "PING_D"=0} -> [w232]
    shift-right: [w223] -> _
    shift-left: State_Type_Definitions,_for_0.26g_versions_and_later_2."Startup" ("Enum") -> [w226]
    shift-right: [w219] -> _
    shift-left: T16 {"xDistance"=0.0, "yDistance"=0.0, "wDistance"=0.0} -> [w221]
    shift-right: [w216] -> _
    shift-left: _ -> [w215]
    tunnel: w21 -> [w214]
    tunnel: w20 -> [w213]
    shift-right: [w210] -> _
    shift-left: T14 {"Recognized Object"=FALSE, "Object X coordinate"=0.0, "Object Y coordinate"=0.0} -> [w212]
    shift-right: [w207] -> _
    shift-left: T12 {"y Stepper Position"=0, "z Stepper Position"=0} -> [w209]
    shift-right: [w204] -> _
    shift-left: T11 {"Yaw"=0.0, "Compass"=0.0} -> [w206]
    shift-right: [w201] -> _
    shift-left: T10 {"Time up flag"=FALSE, "SET TIME TO CHECK"=0.0} -> [w203]
    shift-right: [w199] -> _
    shift-left: T9 {"yStepper desired"=0} -> [w200]
    shift-right: [w195] -> _
    shift-left: T8 {"Left IR Sensor"=0.0, "Arm IR Sensor"=0.0, "Bottom IR Sensor"=0.0} -> [w197]
    stop <- w228 stop-if-true
    # ">>> yStepper command>>>"
    # ">>True Stop Next State >>"
    # ">>Error  >>"
    # ">>Timeout>>"
    # ">>Action states Queue Reference >>"
    # ">>State Logic Queue Reference >>"
    # "TOP LEVEL BASELINE (MAIN PROCESSING LOOP)"
    n58 = Dequeue Element(queue=w241, timeout in ms (-1)=0, error in (no error)=w239) -> (queue out=w233:refnum<queue>, element=w240:string, error out=w234:errorcluster)  [unwired: 1 out]
    "Action State" <- w240
    n59 = Wait (ms)(milliseconds to wait=u32 20) -> ()  [unwired: 1 out]
    n60 = case shown="\"PROCESS IMAGE\"" w240 {
      tunnel: [_ _ _ _ _ _ _ _ _ _ _ _ _ _ _ _ _ _ _ 0 w1842 _ _ _ _ _ _ _ _ _ _ _ _ _ _ _ _ _ _ _ _ _ _ _ _ _ _] -> w236
      tunnel: w233 -> [_ _ _ _ _ _ _ _ _ _ _ _ _ _ _ _ _ _ _ _ _ _ _ _ _ _ _ _ _ _ _ _ _ _ _ _ _ _ _ _ _ _ _ _ _ _ _]
      tunnel: w232 -> [w1601 w1610 w1622 w1633 w1650 w1661 w1672 w1684 w1696 w1708 w1719 w1726 w1741 w1755 w1767 w1775 w1787 w1812 w1822 w1833 w1843 w1852 w1862 w1892 w1903 w1911 w1920 w1933 w1946 w1956 w1965 w1982 w1991 w2002 w2012 w2022 w2032 w2039 w2051 w2067 w2073 w2085 w2097 w2109 w2121 w2133 w2144]
      tunnel: [w1601 w1610 w1622 w1633 w1650 w1661 w1672 w1684 w1696 w1708 w1719 w1726 w1741 w1756 w1767 w1775 w1787 w1813 w1822 w1833 w1843 w1852 w1862 w1891 w1903 w1911 w1920 w1933 w1946 w1956 w1965 w1982 w1991 w2002 w2012 w2022 w2032 w2039 w2051 w2067 w2073 w2085 w2097 w2109 w2121 w2133 w2144] -> w231
      tunnel: [TRUE TRUE _ _ _ _ _ _ _ _ _ _ _ _ _ _ _ _ _ _ _ _ _ _ _ _ _ _ _ _ _ _ _ _ _ _ _ _ _ _ _ _ _ _ _ _ _] -> w228
      tunnel: w226 -> [w1599 w1608 w1621 w1632 w1649 w1660 w1671 w1683 w1695 w1707 w1718 w1725 w1740 w1754 w1766 w1773 w1786 w1811 w1821 w1830 w1840 w1851 w1861 w1890 w1902 w1910 w1919 w1932 w1945 w1955 w1964 w1981 w1990 w2001 w2011 w2021 w2031 w2038 w2050 w2066 w2072 w2084 w2096 w2108 w2120 w2132 w2143]
      tunnel: [_ _ _ _ _ _ _ _ _ _ _ _ _ _ _ _ _ _ _ _ TRUE _ _ _ _ _ _ _ _ _ _ _ _ _ _ _ _ _ _ _ _ _ _ _ _ _ _] -> w225
      tunnel: [w1599 w1608 w1621 w1632 w1649 w1660 w1671 w1683 w1695 w1707 w1718 w1725 w1740 w1754 w1766 w1773 w1786 w1811 w1821 w1830 w1840 w1851 w1861 w1890 w1902 w1910 w1919 w1932 w1945 w1955 w1964 w1981 w1990 w2001 w2011 w2021 w2031 w2038 w2050 w2066 w2072 w2084 w2096 w2108 w2120 w2132 w2143] -> w224
      tunnel: w221 -> [w1598 w1607 w1620 w1635 w1648 w1659 w1670 w1682 w1694 w1706 w1717 w1727 w1739 w1753 w1768 w1777 w1788 w1810 w1823 w1829 w1839 w1853 w1863 w1880 w1901 w1913 w1921 w1934 w1947 w1957 w1966 w1983 w1993 w2004 w2014 w2024 w2034 w2041 w2053 w2069 w2075 w2087 w2099 w2111 w2123 w2135 w2146]
      tunnel: [w1598 w1607 w1620 w1635 w1648 w1659 w1670 w1682 w1694 w1706 w1717 w1727 w1738 w1753 w1768 w1777 w1788 w1809 w1823 w1829 w1839 w1853 w1863 w1879 w1901 w1913 w1921 w1934 w1947 w1957 w1966 w1983 w1993 w2004 w2014 w2024 w2034 w2041 w2053 w2069 w2075 w2087 w2099 w2111 w2123 w2135 w2146] -> w220
      tunnel: w214 -> [w1593 _ _ _ _ _ _ _ _ _ _ _ _ _ _ _ _ _ _ _ _ _ _ _ _ _ _ _ _ _ _ w1977 _ _ _ _ _ _ _ _ _ _ _ _ _ _ _]
      tunnel: w213 -> [_ _ _ _ _ _ _ _ _ _ _ _ _ _ _ _ _ _ _ _ _ _ _ _ _ _ _ _ _ w1949 _ w1979 w1989 _ _ _ _ _ _ _ _ _ _ _ _ _ _]
      tunnel: w212 -> [w1597 w1606 w1619 w1634 w1647 w1658 w1669 w1681 w1693 w1705 w1715 w1724 w1737 w1752 w1761 w1776 w1785 w1801 w1820 w1828 w1838 w1850 w1860 w1885 w1899 w1912 w1918 w1931 w1944 w1951 w1963 w1974 w1992 w2003 w2013 w2023 w2033 w2040 w2052 w2068 w2074 w2086 w2098 w2110 w2122 w2134 w2145]
      tunnel: [w1597 w1606 w1619 w1634 w1647 w1658 w1669 w1681 w1693 w1705 w1715 w1724 w1737 w1752 w1761 w1776 w1785 w1800 w1820 w1828 w1838 w1850 w1860 w1884 w1899 w1912 w1918 w1931 w1944 w1951 w1963 w1973 w1992 w2003 w2013 w2023 w2033 w2040 w2052 w2068 w2074 w2086 w2098 w2110 w2122 w2134 w2145] -> w211
      tunnel: w209 -> [w1596 w1605 w1618 w1636 w1646 w1657 w1668 w1680 w1692 w1704 w1714 w1723 w1736 w1751 w1769 w1778 w1784 w1806 w1819 w1827 w1837 w1849 w1859 w1875 w1898 w1909 w1917 w1930 w1943 w1954 w1962 w1984 w1994 w2000 w2010 w2020 w2030 w2042 w2054 w2065 w2076 w2088 w2100 w2112 w2124 w2136 w2147]
      tunnel: [w1596 w1605 w1618 w1636 w1646 w1657 w1668 w1680 w1692 w1704 w1714 w1723 w1736 w1751 w1769 w1778 w1784 w1805 w1819 w1827 w1837 w1849 w1859 w1874 w1898 w1909 w1917 w1930 w1943 w1954 w1962 w1984 w1994 w2000 w2010 w2020 w2030 w2042 w2054 w2064 w2076 w2088 w2100 w2112 w2124 w2136 w2147] -> w208
      tunnel: w206 -> [w1595 w1604 w1616 w1637 w1644 w1655 w1667 w1678 w1690 w1702 w1713 w1722 w1735 w1744 w1764 w1779 w1783 w1796 w1818 w1826 w1836 w1848 w1858 w1871 w1897 w1906 w1916 w1929 w1942 w1953 w1961 w1985 w1995 w1999 w2007 w2017 w2027 w2043 w2055 w2059 w2077 w2089 w2101 w2113 w2125 w2137 w2148]
      tunnel: [w1595 w1604 w1616 w1637 w1644 w1655 w1667 w1678 w1690 w1702 w1713 w1722 w1735 w1744 w1763 w1779 w1783 w1795 w1818 w1826 w1836 w1848 w1858 w1870 w1897 w1906 w1916 w1929 w1942 w1953 w1961 w1985 w1995 w1999 w2007 w2017 w2027 w2043 w2055 w2059 w2077 w2089 w2101 w2113 w2125 w2137 w2148] -> w205
      tunnel: w203 -> [w1592 w1603 w1617 w1638 w1645 w1656 w1666 w1679 w1691 w1703 w1712 w1721 w1734 w1743 w1760 w1780 w1782 w1792 w1815 w1825 w1835 w1847 w1857 w1868 w1895 w1905 w1915 w1928 w1941 w1952 w1960 w1986 w1996 w1998 w2006 w2016 w2026 w2044 w2056 w2058 w2071 w2083 w2095 w2107 w2119 w2131 w2142]
      tunnel: [w1592 w1603 w1617 w1638 w1645 w1656 w1666 w1679 w1691 w1703 w1712 w1721 w1734 w1743 w1760 w1780 w1782 w1792 w1815 w1825 w1835 w1847 w1857 w1867 w1895 w1905 w1915 w1928 w1941 w1952 w1960 w1986 w1996 w1998 w2006 w2016 w2026 w2044 w2056 w2058 w2071 w2081 w2093 w2105 w2117 w2129 w2141] -> w202
      tunnel: w200 -> [_ _ _ _ _ _ _ _ _ _ _ _ _ _ _ _ _ _ _ _ _ _ _ _ _ _ _ _ _ _ _ _ _ _ _ _ _ _ w2047 _ _ _ _ _ _ _ _]
      tunnel: [w1591 w1602 w1611 w1628 w1639 w1651 w1662 w1673 w1685 w1697 w1709 w1720 w1728 w1742 w1757 w1771 w1781 w1789 w1814 w1824 w1834 w1846 w1854 w1864 w1894 w1904 w1914 w1922 w1935 w1948 w1958 w1967 w1987 w1997 w2005 w2015 w2025 w2035 w2045 w2057 w2070 w2078 w2090 w2102 w2114 w2126 w2138] -> w196
      tunnel: w197 -> [w1591 w1602 w1611 w1628 w1639 w1651 w1662 w1673 w1685 w1697 w1709 w1720 w1728 w1742 w1757 w1772 w1781 w1789 w1814 w1824 w1834 w1846 w1854 w1864 w1894 w1904 w1914 w1922 w1935 w1948 w1958 w1967 w1987 w1997 w2005 w2015 w2025 w2035 w2045 w2057 w2070 w2078 w2090 w2102 w2114 w2126 w2138]
      frame "Exit" {
        # ">>State Logic  >>"
        # ">>> Time cluster >>>"
        # ">>> Yaw >>>"
        # ">>> Stepper position >>>"
        # ">>> Encoders >>>"
        # ">>> Object detection >>>"
        # ">>> Ultrasonic Sensors Detect >>>"
        n61 = call "Imaq Dispose"("All Images? (No)"=TRUE, "Image"=w1593) -> ()  [unwired: 4 in, 1 out]
      }
      frame "----Movement States----" {
        # ">>State Logic  >>"
        # ">>> Time cluster >>>"
        # ">>> Yaw >>>"
        # ">>> Stepper position >>>"
        # ">>> Encoders >>>"
        # ">>> Object detection >>>"
        # ">>> Ultrasonic Sensors Detect >>>"
      }
      frame "FORWARD" {
        # ">>State Logic  >>"
        # ">>> Time cluster >>>"
        # ">>> Yaw >>>"
        # ">>> Stepper position >>>"
        # ">>> Encoders >>>"
        # ">>> Object detection >>>"
        # ">>> Ultrasonic Sensors Detect >>>"
        n62 = Unbundle By Name(w1616) -> ("Yaw"=w1612:dbl)
        n63 = call "MOTOR CONTROL WITH PID AE.vi"("Yaw"=w1612, "Speed"=50.0, "Direction"=MOTOR_CONTROL_WITH_PID_AE_DIRECTION_TYPE_DEF."y-axis movement", "AE Mode"=MOTOR_CONTROL_WITH_PID_AE_DATA_MODE_TYPE_DEF."Write to AE") -> ()  [unwired: 1 out]
      }
      frame "FORWARD - IR ASSIST" {
        # ">>State Logic  >>"
        # ">>> Time cluster >>>"
        # ">>> Yaw >>>"
        # ">>> Stepper position >>>"
        # ">>> Encoders >>>"
        # ">>> Object detection >>>"
        # ">>> Ultrasonic Sensors Detect >>>"
        n64 = Unbundle By Name(w1628) -> ("Left IR Sensor"=w1627:dbl)
        n65 = Subtract(x=w1627, y=15.0) -> (x-y=w1625:dbl)
        n66 = Multiply(x=w1625, y=0.5) -> (x*y=w1623:dbl)
        n67 = call "MOTOR CONTROL WITH PID AE.vi"("Yaw"=w1623, "Speed"=30.0, "Direction"=MOTOR_CONTROL_WITH_PID_AE_DIRECTION_TYPE_DEF."y-axis movement", "AE Mode"=MOTOR_CONTROL_WITH_PID_AE_DATA_MODE_TYPE_DEF."Write to AE") -> ()  [unwired: 1 out]
      }
      frame "LEFT" {
        # ">>State Logic  >>"
        # ">>> Time cluster >>>"
        # ">>> Yaw >>>"
        # ">>> Stepper position >>>"
        # ">>> Encoders >>>"
        # ">>> Object detection >>>"
        # ">>> Ultrasonic Sensors Detect >>>"
        n68 = Unbundle By Name(w1644) -> ("Yaw"=w1641:dbl)
        n69 = call "MOTOR CONTROL WITH PID AE.vi"("Yaw"=w1641, "Speed"=-25.0, "Direction"=MOTOR_CONTROL_WITH_PID_AE_DIRECTION_TYPE_DEF."x-axis movement", "AE Mode"=MOTOR_CONTROL_WITH_PID_AE_DATA_MODE_TYPE_DEF."Write to AE") -> ()  [unwired: 1 out]
      }
      frame "R-ACW" {
        # ">>> IR Sensors >>>"
        # ">>> Time cluster >>>"
        # ">>> Yaw >>>"
        # ">>> Stepper position >>>"
        # ">>> Encoders >>>"
        # ">>> Object detection >>>"
        # ">>> Ultrasonic Sensors Detect >>>"
        n70 = call "MOTOR CONTROL WITH PID AE.vi"("Speed"=-10.0, "Direction"=MOTOR_CONTROL_WITH_PID_AE_DIRECTION_TYPE_DEF."rotation", "AE Mode"=MOTOR_CONTROL_WITH_PID_AE_DATA_MODE_TYPE_DEF."Write to AE") -> ()  [unwired: 1 in, 1 out]
      }
      frame "R-CW" {
        (unwired) -0.2 ("Speed")
        # ">>> Time cluster >>>"
        # ">>> Yaw >>>"
        # ">>> Stepper position >>>"
        # ">>> Encoders >>>"
        # ">>> Object detection >>>"
        # ">>> Ultrasonic Sensors Detect >>>"
        n71 = call "MOTOR CONTROL WITH PID AE.vi"("Speed"=10.0, "Direction"=MOTOR_CONTROL_WITH_PID_AE_DIRECTION_TYPE_DEF."rotation", "AE Mode"=MOTOR_CONTROL_WITH_PID_AE_DATA_MODE_TYPE_DEF."Write to AE") -> ()  [unwired: 1 in, 1 out]
      }
      frame "RIGHT" {
        # ">>> Time cluster >>>"
        # ">>> Yaw >>>"
        # ">>> Stepper position >>>"
        # ">>> Encoders >>>"
        # ">>> Object detection >>>"
        # ">>> Ultrasonic Sensors Detect >>>"
        n72 = Unbundle By Name(w1678) -> ("Yaw"=w1674:dbl)
        n73 = call "MOTOR CONTROL WITH PID AE.vi"("Yaw"=w1674, "Speed"=50.0, "Direction"=MOTOR_CONTROL_WITH_PID_AE_DIRECTION_TYPE_DEF."x-axis movement", "AE Mode"=MOTOR_CONTROL_WITH_PID_AE_DATA_MODE_TYPE_DEF."Write to AE") -> ()  [unwired: 1 out]
      }
      frame "RIGHT - SLOW" {
        # ">>> Time cluster >>>"
        # ">>> Yaw >>>"
        # ">>> Stepper position >>>"
        # ">>> Encoders >>>"
        # ">>> Object detection >>>"
        # ">>> Ultrasonic Sensors Detect >>>"
        n74 = Unbundle By Name(w1690) -> ("Yaw"=w1686:dbl)
        n75 = call "MOTOR CONTROL WITH PID AE.vi"("Yaw"=w1686, "Speed"=30.0, "Direction"=MOTOR_CONTROL_WITH_PID_AE_DIRECTION_TYPE_DEF."x-axis movement", "AE Mode"=MOTOR_CONTROL_WITH_PID_AE_DATA_MODE_TYPE_DEF."Write to AE") -> ()  [unwired: 1 out]
      }
      frame "REVERSE" {
        # ">>> Time cluster >>>"
        # ">>> Yaw >>>"
        # ">>> Stepper position >>>"
        # ">>> Encoders >>>"
        # ">>> Object detection >>>"
        # ">>> Ultrasonic Sensors Detect >>>"
        n76 = Unbundle By Name(w1702) -> ("Yaw"=w1698:dbl)
        n77 = call "MOTOR CONTROL WITH PID AE.vi"("Yaw"=w1698, "Speed"=-50.0, "Direction"=MOTOR_CONTROL_WITH_PID_AE_DIRECTION_TYPE_DEF."y-axis movement", "AE Mode"=MOTOR_CONTROL_WITH_PID_AE_DATA_MODE_TYPE_DEF."Write to AE") -> ()  [unwired: 1 out]
      }
      frame "STOP" {
        n78 = Wait (ms)(milliseconds to wait=u32 100) -> ()  [unwired: 1 out]
        n79 = call "MOTOR CONTROL WITH PID AE.vi"("Direction"=MOTOR_CONTROL_WITH_PID_AE_DIRECTION_TYPE_DEF."stop", "AE Mode"=MOTOR_CONTROL_WITH_PID_AE_DATA_MODE_TYPE_DEF."Write to AE") -> ()  [unwired: 2 in, 1 out]
      }
      frame "----SENSOR READING---- " {
      }
      frame "READ ENCODERS" {
        # ">>> Time cluster >>>"
        # ">>> Yaw >>>"
        # ">>> Stepper position >>>"
        # ">>> Object detection >>>"
        # ">>> Current encoder distance >>>"
        # ">>> Ultrasonic Sensors Detect >>>"
        n80 = call "MOTOR CONTROL WITH PID AE.vi"("AE Mode"=MOTOR_CONTROL_WITH_PID_AE_DATA_MODE_TYPE_DEF."Read from AE") -> ("Speed & distance"=w1732:T1)  [unwired: 3 in]
        n81 = Unbundle By Name(w1732) -> ("xDistance"=w1731:dbl, "yDistance"=w1730:dbl, "wDistance"=w1729:dbl)
        n82 = Bundle By Name(cluster=w1739, "xDistance"=w1731, "yDistance"=w1730, "wDistance"=w1729) -> (w1738:T16)
      }
      frame "READ ULTRASONIC" {
        (unwired) navX_type_def."Read Values" ("Mode")
        (unwired) MOTOR_CONTROL_NO_PID_Type_Def."Latch" ("Direction")
        # ">>State Logic  >>"
        # ">>> Time cluster >>>"
        # ">>> Ultrasonic Sensors Detect >>>"
        # ">>> Object detection >>>"
        # ">>> Encoders >>>"
        # ">>> Stepper position >>>"
        # ">>> Yaw >>>"
        n83 = call "Arduino Interfacing VI.vi"("AE Mode"=Arduino_Interfacing."Read From Arduino") -> ("Arduino Data"=w1749:T4)  [unwired: 3 in, 1 out]
        n84 = Unbundle By Name(w1749) -> ("PING A"=w1748:u8, "PING B"=w1747:u8, "PING C"=w1746:u8, "PING D"=w1745:u8)
        n85 = Bundle By Name(cluster=w1755, "PING_A"=w1748, "PING_B"=w1747, "PING_C"=w1746, "PING_D"=w1745) -> (w1756:T15)
      }
      frame "READ NAVX" {
        # ">>> Time cluster >>>"
        # ">>> Yaw >>>"
        # ">>> Ultrasonic Sensors Detect >>>"
        # ">>> Object detection >>>"
        # ">>> Encoders >>>"
        # ">>> Stepper position >>>"
        n86 = call "navX reading VI.vi"("Mode"=navX_type_def."Read Values") -> ("NavX Readings"=w1759:T3)  [unwired: 2 in, 3 out]
        n87 = Unbundle By Name(w1759) -> ("Heading"=w1758:dbl)
        n88 = Unbundle By Name(w1759) -> ("Yaw"=w1762:dbl)
        n89 = Bundle By Name(cluster=w1764, "Yaw"=w1762, "Compass"=w1758) -> (w1763:T11)
      }
      frame "READ IR" {
        w1774 = T34 [enum."A/AI0"] items=["Not Connected", "AudioIn/Left", "AudioIn/Right", "C/AI0", "C/AI1", "A/AI0", "A/AI1", "A/AI2", "A/AI3", "A/AI4", "A/AI5", "A/AI6", "A/AI7", "B/AI0", "B/AI1", "B/AI2", "B/AI3", "B/AI4", "B/AI5", "B/AI6", "B/AI7", "AI/AI0", "AI/AI1", "AI/AI2", "AI/AI3", "A/AI0 (DIFF)", "A/AI1 (DIFF)", "A/AI2 (DIFF)", "A/AI3 (DIFF)", "B/AI0 (DIFF)", "B/AI1 (DIFF)", "B/AI2 (DIFF)", "B/AI3 (DIFF)"] ("AI Channel")
        # ">>State Logic  >>"
        # ">>> Time cluster >>>"
        # ">>> Ultrasonic Sensors Detect >>>"
        # ">>> Object detection >>>"
        # ">>> Encoders >>>"
        # ">>> Stepper position >>>"
        # ">>> Yaw >>>"
        n90 = call <vilib>:"Sharp IR.vi"("AI Channel"=w1774) -> ("Sharp IR Distance"=w1770:dbl)  [unwired: 8 in, 2 out]
        n91 = Bundle By Name(cluster=w1772, "Left IR Sensor"=w1770) -> (w1771:T8)
      }
      frame "----SYSTEM MODES----" {
        (unwired) I2C_MASTER_Type_Def."Last State" ("Arduino Mode")
        # ">>> Object detection >>>"
        # ">>> Yaw >>>"
        # ">>> Ultrasonic Sensors Detect >>>"
        # ">>> Encoders >>>"
        # ">>> Stepper position >>>"
      }
      frame "INIT" {
        w1807 = u8 0
        w1808 = 0.0
        # ">>> Time cluster >>>"
        # ">>> Object detection >>>"
        # ">>> Yaw >>>"
        # ">>> Ultrasonic Sensors Detect >>>"
        # ">>> Encoders >>>"
        # ">>> Stepper position >>>"
        # ">>State Logic  >>"
        n92 = call "Arduino Interfacing VI.vi"("AE Mode"=Arduino_Interfacing."Initialize") -> ()  [unwired: 3 in, 2 out]
        n93 = call "FGV Stop.vi"("Init/Read/Write State"=States_for_Action_Engine."Initialize") -> ()  [unwired: 2 in, 2 out]
        n94 = call "Elasped Timer.vi"("Action"=Elapsed_timer_control."Initialize") -> ()  [unwired: 7 in, 4 out]
        n95 = call "MOTOR CONTROL WITH PID AE.vi"("AE Mode"=MOTOR_CONTROL_WITH_PID_AE_DATA_MODE_TYPE_DEF."Init AE") -> ()  [unwired: 3 in, 1 out]
        n96 = Bundle By Name(cluster=w1801, "Recognized Object"=FALSE, "Object X coordinate"=0.0, "Object Y coordinate"=0.0) -> (w1800:T14)
        n97 = Bundle By Name(cluster=w1806, "y Stepper Position"=u8 0, "z Stepper Position"=u8 0) -> (w1805:T12)
        n98 = Bundle By Name(cluster=w1810, "xDistance"=w1808, "yDistance"=w1808, "wDistance"=w1808) -> (w1809:T16)
        n99 = Bundle By Name(cluster=w1812, "PING_A"=w1807, "PING_B"=w1807, "PING_C"=w1807, "PING_D"=w1807) -> (w1813:T15)
        n100 = Bundle By Name(cluster=w1796, "Yaw"=0.0) -> (w1795:T11)
      }
      frame "ARDUINO - ULTRASONIC" {
        # ">>> Object detection >>>"
        # ">>> Yaw >>>"
        # ">>> Ultrasonic Sensors Detect >>>"
        # ">>> Encoders >>>"
        # ">>> Stepper position >>>"
        # ">>State Logic  >>"
        n101 = call "Arduino Interfacing VI.vi"("Data to Write"=I2C_MASTER_WRITE_NEW_Type_Def."Ultrasonic sensors", "AE Mode"=Arduino_Interfacing."Write to Arduino") -> ()  [unwired: 2 in, 2 out]
      }
      frame "NAVX CALIBRATE" {
        # ">>> Object detection >>>"
        # ">>> Yaw >>>"
        # ">>> Ultrasonic Sensors Detect >>>"
        # ">>> Encoders >>>"
        # ">>> Stepper position >>>"
        # ">>State Logic  >>"
        # "Adds a 15 second delay to the startup process \nfor the NavX to calibrate"
        n102 = Wait (ms)(milliseconds to wait=u32 1000) -> ()  [unwired: 1 out]
      }
      frame "NO ACTION", Default {
        (unwired) u8 0 ("y Stepper value")
        (unwired) TRUE ("Latch")
        (unwired) navX_type_def."Read Values" ("Mode")
        (unwired) MOTOR_CONTROL_NO_PID_Type_Def."Latch" ("Direction")
        # ">>> Object detection >>>"
        # ">>> Yaw >>>"
        # ">>> Ultrasonic Sensors Detect >>>"
        # ">>> Encoders >>>"
        # ">>> Stepper position >>>"
        # ">>State Logic  >>"
        n103 = case shown="4" w1840 {
          tunnel: [0 100] -> w1842
          frame 1, Default {
          }
          frame 4 {
          }
        }
      }
      frame "----RESET CASES----" {
        (unwired) I2C_MASTER_Type_Def."Last State" ("Arduino Mode")
        # ">>> Object detection >>>"
        # ">>> Yaw >>>"
        # ">>> Ultrasonic Sensors Detect >>>"
        # ">>> Encoders >>>"
        # ">>> Stepper position >>>"
        # ">>State Logic  >>"
      }
      frame "RESET ENCODERS" {
        # ">>> Object detection >>>"
        # ">>> Yaw >>>"
        # ">>> Ultrasonic Sensors Detect >>>"
        # ">>> Encoders >>>"
        # ">>> Stepper position >>>"
        # ">>State Logic  >>"
        n104 = call "MOTOR CONTROL WITH PID AE.vi"("Direction"=MOTOR_CONTROL_WITH_PID_AE_DIRECTION_TYPE_DEF."reset encoders", "AE Mode"=MOTOR_CONTROL_WITH_PID_AE_DATA_MODE_TYPE_DEF."Write to AE") -> ()  [unwired: 2 in, 1 out]
      }
      frame "RESET FLAGS" {
        (unwired) I2C_MASTER_Type_Def."Last State" ("Arduino Mode")
        # "Resets any software variables\nand/or non-critical states"
        n105 = Wait (ms)(milliseconds to wait=u32 20) -> ()  [unwired: 1 out]
        n106 = Bundle By Name(cluster=w1868, "Time up flag"=FALSE, "SET TIME TO CHECK"=0.0) -> (w1867:T10)
        n107 = Bundle By Name(cluster=w1885, "Recognized Object"=FALSE, "Object X coordinate"=0.0, "Object Y coordinate"=0.0) -> (w1884:T14)
        n108 = Bundle By Name(cluster=w1875, "y Stepper Position"=u8 0, "z Stepper Position"=u8 0) -> (w1874:T12)
        n109 = Bundle By Name(cluster=w1880, "xDistance"=0.0, "yDistance"=0.0, "wDistance"=0.0) -> (w1879:T16)
        n110 = Bundle By Name(cluster=w1892, "PING_A"=u8 0, "PING_B"=u8 0, "PING_C"=u8 0, "PING_D"=u8 0) -> (w1891:T15)
        n111 = Bundle By Name(cluster=w1871, "Yaw"=0.0) -> (w1870:T11)
      }
      frame "RESET YAW" {
        n112 = Wait (ms)(milliseconds to wait=u32 100) -> ()  [unwired: 1 out]
        n113 = call "navX reading VI.vi"("Mode"=navX_type_def."Zero Yaw") -> ()  [unwired: 2 in, 4 out]
      }
      frame "RESET ARM" {
        n114 = call "Arduino Interfacing VI.vi"("Data to Write"=I2C_MASTER_WRITE_NEW_Type_Def."Soft Reset", "AE Mode"=Arduino_Interfacing."Write to Arduino") -> ()  [unwired: 2 in, 2 out]
      }
      frame "--------CAM STATES-------" {
      }
      frame "OPEN LOG CAM" {
        n115 = call "Webcam AE.vi"("Session In"=T31 "cam0", "Camera states"=Webcam_AE."Initialize Camera") -> ("error out"=w1925:errorcluster, "Session Out"=w1924:T31)  [unwired: 1 in, 1 out]
        n116 = call "Webcam AE.vi"("error in (no error)"=w1925, "Session In"=w1924, "Camera states"=Webcam_AE."Open Camera") -> ()  [unwired: 3 out]
      }
      frame "OPEN LIFE CAM" {
        n117 = call "Webcam AE.vi"("Session In"=T31 "cam1", "Camera states"=Webcam_AE."Initialize Camera") -> ("error out"=w1938:errorcluster, "Session Out"=w1937:T31)  [unwired: 1 in, 1 out]
        n118 = call "Webcam AE.vi"("error in (no error)"=w1938, "Session In"=w1937, "Camera states"=Webcam_AE."Open Camera") -> ()  [unwired: 3 out]
      }
      frame "CAM ACQ" {
        # ">>State Logic  >>"
        # ">>> Time cluster >>>"
        # ">>> Yaw >>>"
        # ">>> Stepper position >>>"
        # ">>> Encoders >>>"
        # ">>> Object detection >>>"
        # ">>> Ultrasonic Sensors Detect >>>"
        n119 = call "Webcam AE.vi"("error in (no error)"=w1949, "Camera states"=Webcam_AE."Continuous Acquisition") -> ()  [unwired: 1 in, 3 out]
      }
      frame "CAM CLOSE" {
        # ">>State Logic  >>"
        # ">>> Time cluster >>>"
        # ">>> Yaw >>>"
        # ">>> Stepper position >>>"
        # ">>> Encoders >>>"
        # ">>> Object detection >>>"
        # ">>> Ultrasonic Sensors Detect >>>"
        n120 = call "Webcam AE.vi"("Camera states"=Webcam_AE."Close Camera") -> ()  [unwired: 2 in, 3 out]
      }
      frame "PROCESS IMAGE" {
        # ">>State Logic  >>"
        # ">>> Time cluster >>>"
        # ">>> Yaw >>>"
        # ">>> Stepper position >>>"
        # ">>> Encoders >>>"
        # ">>> Object detection >>>"
        # ">>> Ultrasonic Sensors Detect >>>"
        n121 = call "Webcam AE.vi"("error in (no error)"=w1979, "Camera states"=Webcam_AE."Retrieve Image") -> ("error out"=w1975:errorcluster, "Image Out"=w1978:T24)  [unwired: 1 in, 1 out]
        n122 = call "Object Detection SubVI.vi"("Error In"=w1975, "Mode"="Object recognition mode", "Image Dest"=w1977, "Image in"=w1978) -> ("Object Center Coordinates"=w1972:cluster{"x":sgl, "y":sgl}, "Object detection cluster"=w1968:T2)  [unwired: 2 out]
        "Object detection cluster" <- w1968
        "Object Center Coordinates" <- w1972
        n123 = Unbundle By Name(w1968) -> ("Object detected?"=w1969:bool)
        n124 = Unbundle By Name(w1972) -> ("x"=w1971:sgl, "y"=w1970:sgl)
        n125 = Bundle By Name(cluster=w1974, "Recognized Object"=w1969, "Object X coordinate"=w1971, "Object Y coordinate"=w1970) -> (w1973:T14)
      }
      frame "DISPOSE BUFFERS" {
        # ">>State Logic  >>"
        # ">>> Time cluster >>>"
        # ">>> Yaw >>>"
        # ">>> Stepper position >>>"
        # ">>> Encoders >>>"
        # ">>> Object detection >>>"
        # ">>> Ultrasonic Sensors Detect >>>"
        n126 = call "Webcam AE.vi"("error in (no error)"=w1989, "Camera states"=Webcam_AE."Dispose Image Buffers") -> ()  [unwired: 1 in, 3 out]
      }
      frame "-----ARM ACTIONS-----" {
      }
      frame "CLOSE CLAW" {
        n127 = call "Arduino Interfacing VI.vi"("Data to Write"=I2C_MASTER_WRITE_NEW_Type_Def."Close Claw", "AE Mode"=Arduino_Interfacing."Write to Arduino") -> ()  [unwired: 2 in, 2 out]
      }
      frame "OPEN CLAW" {
        n128 = call "Arduino Interfacing VI.vi"("Data to Write"=I2C_MASTER_WRITE_NEW_Type_Def."Open Claw", "AE Mode"=Arduino_Interfacing."Write to Arduino") -> ()  [unwired: 2 in, 2 out]
      }
      frame "Z STEPPER CAM HEIGHT" {
        n129 = call "Arduino Interfacing VI.vi"("Data to Write"=I2C_MASTER_WRITE_NEW_Type_Def."zStepper 6k", "AE Mode"=Arduino_Interfacing."Write to Arduino") -> ()  [unwired: 2 in, 2 out]
      }
      frame "Z STEPPER GRAB HEIGHT" {
        # ">>State Logic  >>"
        # ">>> Time cluster >>>"
        # ">>> Yaw >>>"
        # ">>> Stepper position >>>"
        # ">>> Encoders >>>"
        # ">>> Object detection >>>"
        # ">>> Ultrasonic Sensors Detect >>>"
        n130 = call "Arduino Interfacing VI.vi"("Data to Write"=I2C_MASTER_WRITE_NEW_Type_Def."zStepper 100", "AE Mode"=Arduino_Interfacing."Write to Arduino") -> ()  [unwired: 2 in, 2 out]
      }
      frame "Y STEPPER CONTROL" {
        # ">>State Logic  >>"
        # ">>> yStepper command>>>"
        # ">>> Time cluster >>>"
        # ">>> Yaw >>>"
        # ">>> Stepper position >>>"
        # ">>> Encoders >>>"
        # ">>> Object detection >>>"
        # ">>> Ultrasonic Sensors Detect >>>"
        n131 = Unbundle By Name(w2047) -> ("yStepper desired"=w2046:u8)
        n132 = call "Arduino Interfacing VI.vi"("y Stepper value"=w2046, "Data to Write"=I2C_MASTER_WRITE_NEW_Type_Def."yStepper control", "AE Mode"=Arduino_Interfacing."Write to Arduino") -> ()  [unwired: 1 in, 2 out]
      }
      frame "READ STEPPER VALUES" {
        # ">>State Logic  >>"
        # ">>> Time cluster >>>"
        # ">>> Yaw >>>"
        # ">>> Stepper position >>>"
        # ">>> Encoders >>>"
        # ">>> Object detection >>>"
        # ">>> Ultrasonic Sensors Detect >>>"
        n133 = call "Arduino Interfacing VI.vi"("AE Mode"=Arduino_Interfacing."Read From Arduino") -> ("Arduino Data"=w2062:T4)  [unwired: 3 in, 1 out]
        n134 = Unbundle By Name(w2062) -> ("y Stepper Position"=w2061:u8, "z Stepper Position"=w2060:u8)
        n135 = Bundle By Name(cluster=w2065, "y Stepper Position"=w2061, "z Stepper Position"=w2060) -> (w2064:T12)
      }
      frame " -----TIMING-----" {
        # ">>State Logic  >>"
        # ">>> Time cluster >>>"
        # ">>> Yaw >>>"
        # ">>> Stepper position >>>"
        # ">>> Encoders >>>"
        # ">>> Object detection >>>"
        # ">>> Ultrasonic Sensors Detect >>>"
      }
      frame "SET TIMER 1" {
        # ">>State Logic  >>"
        # ">>> Time cluster >>>"
        # ">>> Yaw >>>"
        # ">>> Stepper position >>>"
        # ">>> Encoders >>>"
        # ">>> Object detection >>>"
        # ">>> Ultrasonic Sensors Detect >>>"
        n136 = call "Elasped Timer.vi"("Time Setting"=1.0, "Action"=Elapsed_timer_control."Initialize") -> ()  [unwired: 6 in, 4 out]
        n137 = Bundle By Name(cluster=w2083, "Time up flag"=FALSE) -> (w2081:T10)
      }
      frame "SET TIMER 2" {
        # ">>State Logic  >>"
        # ">>> Time cluster >>>"
        # ">>> Yaw >>>"
        # ">>> Stepper position >>>"
        # ">>> Encoders >>>"
        # ">>> Object detection >>>"
        # ">>> Ultrasonic Sensors Detect >>>"
        n138 = call "Elasped Timer.vi"("Time Setting"=2.0, "Action"=Elapsed_timer_control."Initialize") -> ()  [unwired: 6 in, 4 out]
        n139 = Bundle By Name(cluster=w2095, "Time up flag"=FALSE) -> (w2093:T10)
      }
      frame "SET TIMER 3" {
        # ">>State Logic  >>"
        # ">>> Time cluster >>>"
        # ">>> Yaw >>>"
        # ">>> Stepper position >>>"
        # ">>> Encoders >>>"
        # ">>> Object detection >>>"
        # ">>> Ultrasonic Sensors Detect >>>"
        n140 = call "Elasped Timer.vi"("Time Setting"=3.0, "Action"=Elapsed_timer_control."Initialize") -> ()  [unwired: 6 in, 4 out]
        n141 = Bundle By Name(cluster=w2107, "Time up flag"=FALSE) -> (w2105:T10)
      }
      frame "SET TIMER 4" {
        # ">>State Logic  >>"
        # ">>> Time cluster >>>"
        # ">>> Yaw >>>"
        # ">>> Stepper position >>>"
        # ">>> Encoders >>>"
        # ">>> Object detection >>>"
        # ">>> Ultrasonic Sensors Detect >>>"
        n142 = call "Elasped Timer.vi"("Time Setting"=4.0, "Action"=Elapsed_timer_control."Initialize") -> ()  [unwired: 6 in, 4 out]
        n143 = Bundle By Name(cluster=w2119, "Time up flag"=FALSE) -> (w2117:T10)
      }
      frame "SET TIMER 5" {
        # ">>State Logic  >>"
        # ">>> Time cluster >>>"
        # ">>> Yaw >>>"
        # ">>> Stepper position >>>"
        # ">>> Encoders >>>"
        # ">>> Object detection >>>"
        # ">>> Ultrasonic Sensors Detect >>>"
        n144 = call "Elasped Timer.vi"("Time Setting"=5.0, "Action"=Elapsed_timer_control."Initialize") -> ()  [unwired: 6 in, 4 out]
        n145 = Bundle By Name(cluster=w2131, "Time up flag"=FALSE) -> (w2129:T10)
      }
      frame "START TIMER" {
        # ">>State Logic  >>"
        # ">>> Time cluster >>>"
        # ">>> Yaw >>>"
        # ">>> Stepper position >>>"
        # ">>> Encoders >>>"
        # ">>> Object detection >>>"
        # ">>> Ultrasonic Sensors Detect >>>"
        n146 = call "Elasped Timer.vi"("Action"=Elapsed_timer_control."Start") -> ("Time Out?!"=w2139:bool)  [unwired: 7 in, 3 out]
        n147 = Bundle By Name(cluster=w2142, "Time up flag"=w2139) -> (w2141:T10)
      }
    }
    "State Logic" <- w224
    n148 = local read "TASK ENABLE"() -> (w218:bool)
    n149 = Not(x=w218) -> (.not. x?=w217:bool)
    n150 = case shown="True" w225 {
      tunnel: w229 -> [w253 w286]
      tunnel: w233 -> [w249 w288]
      tunnel: [w253 w286] -> w238
      tunnel: [w249 w289] -> w237
      tunnel: w234 -> [_ w284]
      tunnel: w236 -> [_ w285]
      tunnel: w231 -> [w252 w291]
      tunnel: [w252 w291] -> w230
      tunnel: "STOP TASK" -> [_ w274]
      tunnel: w224 -> [w251 w290]
      tunnel: [w251 w287] -> w223
      tunnel: w220 -> [w250 w280]
      tunnel: [w250 w280] -> w219
      tunnel: w217 -> [_ w275]
      tunnel: [w248 w272] -> w216
      tunnel: w215 -> [w248 w271]
      tunnel: w211 -> [w247 w268]
      tunnel: [w247 w268] -> w210
      tunnel: w208 -> [w246 w264]
      tunnel: [w246 w264] -> w207
      tunnel: w205 -> [w245 w262]
      tunnel: [w245 w262] -> w204
      tunnel: w202 -> [w244 w260]
      tunnel: [w244 w260] -> w201
      tunnel: w200 -> [w243 w259]
      tunnel: [w243 w258] -> w199
      tunnel: [_ w256] -> w198
      tunnel: w196 -> [w242 w254]
      tunnel: [w242 w254] -> w195
      frame False {
        # ">>> IR Sensors >>>"
        # ">>> IR Sensors >>>"
        # ">>> yStepper command>>>"
        # ">>> Time cluster >>>"
        # ">>> Yaw >>>"
        # ">>> Stepper position >>>"
        # ">>> Encoders >>>"
        # ">>> Object detection >>>"
        # ">>> Ultrasonic Sensors Detect >>>"
        # ">>> Time cluster >>>"
        # ">>> Yaw >>>"
        # ">>> Stepper position >>>"
        # ">>> Encoders >>>"
        # ">>> Object detection >>>"
        # ">>> Ultrasonic Sensors Detect >>>"
      }
      frame True {
        # ">>State Logic Queue Reference >>"
        # ">>Timeout>>"
        # ">>> yStepper command>>>"
        # ">>> Time cluster >>>"
        # ">>> Object detection >>>"
        # ">>> Yaw >>>"
        # ">>> Ultrasonic Sensors Detect >>>"
        # ">>> Encoders >>>"
        # ">>> Stepper position >>>"
        # ">>State Logic  >>"
        # ">>True Stop Next State >>"
        # ">>Action Queue>>"
        # ">> Manual override >>"
        # ">>> Time cluster >>>"
        # ">>> Yaw >>>"
        # ">>> Stepper position >>>"
        # ">>> Encoders >>>"
        # ">>> Object detection >>>"
        # ">>> Ultrasonic Sensors Detect >>>"
        # ">>Action Queue>>"
        # ">>State Logic Queue Reference >>"
        n151 = Or(x=w274, y=w275) -> (x .or. y?=w273:bool)
        n152 = Unbundle By Name(w254) -> ("Left IR Sensor"=w255:dbl)
        "Left IR Sensor" <- w255
        n153 = Unbundle By Name(w260) -> ("Time up flag"=w261:bool)
        "Time up flag" <- w261
        n154 = Unbundle By Name(w262) -> ("Yaw"=w263:dbl, "Compass"=w257:dbl)
        n155 = Unbundle By Name(w264) -> ("y Stepper Position"=w266:u8, "z Stepper Position"=w265:u8)
        n156 = Unbundle By Name(w280) -> ("xDistance"=w277:dbl, "yDistance"=w278:dbl, "wDistance"=w279:dbl)
        n157 = Unbundle By Name(w268) -> ("Recognized Object"=w267:bool, "Object X coordinate"=w270:dbl, "Object Y coordinate"=w269:dbl)
        n158 = Unbundle By Name(w291) -> ("PING_A"=w283:u8, "PING_B"=w282:u8, "PING_C"=w281:u8, "PING_D"=w276:u8)
        n159 = case shown="31" w290 {
          tunnel: [w294 w300 w312 w321 w395 w408 w443 w495 w536 w582 w624 w677 w723 w762 w821 w865 w904 w951 w992 w1043 w1079 w1129 w1171 w1213 w1243 w1290 w1330 w1380 w1424 w1463 w1510 w1557] -> w289
          tunnel: w288 -> [w294 w303 w313 w324 w397 w409 w452 w493 w540 w583 w630 w670 w726 w769 w811 w868 w910 w950 w995 w1033 w1085 w1119 w1166 w1204 w1247 w1297 w1335 w1370 w1427 w1469 w1509 w1556]
          tunnel: [State_Type_Definitions,_for_0.26g_versions_and_later_2."Idle" ("Enum") State_Type_Definitions,_for_0.26g_versions_and_later_2."Idle" ("Enum") w308 w323 State_Type_Definitions,_for_0.26g_versions_and_later_2."Shutdown" ("Enum") w410 w450 w496 w537 w581 w625 w676 w724 w764 w820 w866 w911 w952 w994 w1042 w1086 w1128 w1172 w1205 w1244 w1291 w1331 w1379 w1425 w1470 w1511 w1558] -> w287
          tunnel: w286 -> [_ _ w311 w327 _ w415 w446 w492 w541 w590 w629 w674 w727 w768 w818 w863 w909 w948 w996 w1040 w1084 w1126 w1169 w1212 w1251 w1296 w1338 w1377 w1422 w1468 w1507 w1554]
          tunnel: w285 -> [_ _ _ w326 _ w414 w445 w491 w542 w589 w628 w673 w720 w767 w817 w862 w908 w947 w997 w1039 w1083 w1125 w1168 w1210 w1246 w1295 w1337 w1376 w1421 w1467 w1506 w1553]
          tunnel: w284 -> [_ _ w310 w322 _ w413 w444 w490 w543 w588 w627 w672 w719 w766 w819 w864 w907 w946 w998 w1041 w1082 w1127 w1167 w1211 w1250 w1294 w1336 w1378 w1423 w1466 w1505 w1552]
          tunnel: w273 -> [_ _ _ _ _ w407 w451 w489 w544 w585 w623 w675 w725 w770 w812 w869 w905 w949 w999 w1034 w1080 w1120 w1170 w1208 w1249 w1289 w1334 w1371 w1428 w1464 w1508 w1555]
          tunnel: w283 -> [_ _ _ _ _ _ _ _ _ _ _ _ _ _ _ _ _ _ _ _ _ _ _ _ _ _ _ _ _ _ _ _]
          tunnel: w282 -> [_ _ _ _ _ _ _ w488 _ _ _ w666 w708 w760 _ w855 _ _ _ _ _ _ _ _ _ _ _ _ w1414 _ _ _]
          tunnel: w281 -> [_ _ _ _ _ _ _ w487 _ _ _ w667 w709 w761 _ w856 _ _ _ _ _ _ _ _ _ _ _ _ w1415 _ _ _]
          tunnel: w279 -> [_ _ _ _ _ _ _ _ _ w587 _ _ _ _ _ _ _ _ _ _ _ _ _ _ _ _ _ _ _ _ _ _]
          tunnel: w278 -> [_ _ _ _ _ w406 _ _ w535 _ _ _ _ w765 _ _ _ _ _ _ _ _ _ _ _ _ _ _ _ _ _ _]
          tunnel: w277 -> [_ _ _ _ _ _ _ _ _ _ _ _ w714 _ _ _ _ _ _ _ _ _ _ _ _ _ _ _ _ _ _ w1546]
          tunnel: w276 -> [_ _ _ _ _ _ _ _ _ _ _ _ _ _ _ _ _ _ _ _ _ _ _ _ _ _ _ _ _ _ _ _]
          tunnel: [State_Type_Definitions,_for_0.26g_versions_and_later_2."Idle" ("Enum") State_Type_Definitions,_for_0.26g_versions_and_later_2."Idle" ("Enum") State_Type_Definitions,_for_0.26g_versions_and_later_2."Idle" ("Enum") State_Type_Definitions,_for_0.26g_versions_and_later_2."Idle" ("Enum") State_Type_Definitions,_for_0.26g_versions_and_later_2."Shutdown" ("Enum") w403 w449 w494 w538 w578 w622 w669 w722 w763 w822 w867 w903 w953 w993 w1044 w1078 w1130 w1173 w1206 w1245 w1292 w1333 w1381 w1426 w1462 w1512 w1559] -> w272
          tunnel: w271 -> [_ _ w308 _ _ _ _ _ _ _ _ _ _ _ _ _ _ _ _ _ _ _ _ _ _ _ _ _ _ _ _ _]
          tunnel: w267 -> [_ _ _ _ _ _ _ _ _ _ _ _ _ _ _ _ _ _ _ _ _ _ _ w1207 _ _ _ _ _ _ _ _]
          tunnel: w270 -> [_ _ _ _ _ _ _ _ _ _ _ _ _ _ _ _ _ _ _ _ _ _ _ _ _ _ _ _ _ _ _ w1549]
          tunnel: w269 -> [_ _ _ _ _ _ _ _ _ _ _ _ _ _ _ _ _ _ w988 _ _ _ _ _ _ _ _ _ _ _ _ _]
          tunnel: w266 -> [_ _ _ _ _ _ _ _ _ _ _ _ _ _ _ _ _ _ w987 _ _ _ _ _ _ _ _ _ _ _ _ _]
          tunnel: w265 -> [_ _ _ _ _ _ w448 _ _ _ w620 _ _ _ w815 _ _ _ _ w1037 _ w1123 w1165 _ w1248 _ _ w1374 _ _ _ _]
          tunnel: w263 -> [_ _ _ _ _ _ _ _ _ _ _ _ _ _ _ _ _ _ _ _ _ _ _ _ _ _ _ _ _ _ _ _]
          tunnel: w261 -> [_ _ _ _ _ _ _ _ _ _ _ _ _ _ _ _ w901 w943 _ _ w1076 _ _ _ _ _ _ _ _ w1460 w1502 _]
          tunnel: w259 -> [w292 w298 w307 w319 w393 w402 w447 w486 w539 w577 w621 w668 w718 w759 w810 w860 w902 w944 w990 w1032 w1077 w1118 w1162 w1203 w1242 w1293 w1332 w1369 w1419 w1461 w1503 w1550]
          tunnel: [w292 w297 w307 w319 w393 w402 w447 w486 w539 w577 w621 w668 w718 w759 w810 w860 w902 w944 w989 w1032 w1077 w1118 w1162 w1203 w1242 w1293 w1332 w1369 w1419 w1461 w1503 w1550] -> w258
          tunnel: w257 -> [_ _ _ _ _ _ _ _ _ _ _ _ _ _ _ _ _ _ _ _ _ _ _ _ _ w1288 _ _ _ _ _ _]
          tunnel: [_ _ _ TRUE _ _ _ _ _ _ _ _ _ _ _ _ _ _ _ _ _ _ _ _ _ _ _ _ _ _ _ _] -> w256
          tunnel: w255 -> [_ _ _ _ _ _ _ _ _ _ _ _ _ _ _ _ _ _ _ _ _ _ _ _ _ _ _ _ _ _ _ _]
          frame 0 {
            # ">>> yStepper command>>>"
          }
          frame 1 {
            # ">>> yStepper command>>>"
            n160 = for {
              shift-right: [w306] -> w300
              shift-left: w303 -> [w305]
              tunnel: string[] ["INIT", "RESET ARM", "RESET FLAGS", "RESET YAW", "NAVX CALIBRATE"] -> [w304] mode=indexing
              n161 = Enqueue Element(queue=w305, element=w304) -> (queue out=w306:refnum<queue>)  [unwired: 2 in, 2 out]
            }
            n162 = Bundle By Name(cluster=w298, "yStepper desired"=u8 0) -> (w297:T9)
          }
          frame 3 {
            # ">>> yStepper command>>>"
            n163 = Flush Queue(queue=w311, error in (no error)=w310) -> ()  [unwired: 3 out]
            n164 = for {
              shift-right: [w317] -> w312
              shift-left: w313 -> [w316]
              tunnel: string[] ["STOP", "RESET ENCODERS", "RESET YAW", "RESET ARM", "RESET FLAGS", "DISPOSE BUFFERS", "CAM CLOSE"] -> [w315] mode=indexing
              n165 = Enqueue Element(queue=w316, element=w315) -> (queue out=w317:refnum<queue>)  [unwired: 2 in, 2 out]
            }
          }
          frame 4, Default {
            (unwired) TRUE ("Green LED")
            # ">>> yStepper command>>>"
            n166 = Dequeue Element(queue=w327, timeout in ms (-1)=w326, error in (no error)=w322) -> (element=w325:T7)  [unwired: 3 out]
            n167 = case shown="\"Start Task 8 - BALL\"" w325 {
              tunnel: [w329 w336 w343 w350 w357 w364 w371 w373 w381 w387] -> w321
              tunnel: w324 -> [w330 w337 w344 w351 w358 w365 w371 w374 w380 w388]
              tunnel: [State_Type_Definitions."Task 1" ("Enum") State_Type_Definitions,_for_0.26g_versions_and_later_2."Task 2:Raise Arm" ("Enum") State_Type_Definitions,_for_0.26g_versions_and_later_2."Task 3" ("Enum") State_Type_Definitions,_for_0.26g_versions_and_later_2."Task 4_A" ("Enum") State_Type_Definitions."Task 5A: ARM CAM HEIGHT" ("Enum") State_Type_Definitions,_for_0.26g_versions_and_later_2."Task 6_A" ("Enum") State_Type_Definitions,_for_0.26g_versions_and_later_2."Idle" ("Enum") State_Type_Definitions,_for_0.26g_versions_and_later_2."Shutdown" ("Enum") State_Type_Definitions,_for_0.26g_versions_and_later_2."Task 9A: Raise Arm" ("Enum") State_Type_Definitions,_for_0.26g_versions_and_later_2."Task 8A: RAISE ARM" ("Enum")] -> w323
              frame "Start Task 1" {
                n168 = for {
                  shift-right: [w334] -> w329
                  shift-left: w330 -> [w333]
                  tunnel: string[] ["RESET ENCODERS", "RESET YAW", "FORWARD", "READ ENCODERS"] -> [w332] mode=indexing
                  n169 = Enqueue Element(queue=w333, element=w332) -> (queue out=w334:refnum<queue>)  [unwired: 2 in, 2 out]
                }
              }
              frame "Start Task 2" {
                n170 = for {
                  shift-right: [w341] -> w336
                  shift-left: w337 -> [w340]
                  tunnel: string[] ["RESET ENCODERS", "RESET YAW", "READ ULTRASONIC", "ARDUINO - ULTRASONIC"] -> [w339] mode=indexing
                  n171 = Enqueue Element(queue=w340, element=w339) -> (queue out=w341:refnum<queue>)  [unwired: 2 in, 2 out]
                }
              }
              frame "Start Task 3" {
                n172 = for {
                  shift-right: [w348] -> w343
                  shift-left: w344 -> [w347]
                  tunnel: string[] ["RESET ENCODERS", "READ ENCODERS", "R-ACW"] -> [w346] mode=indexing
                  n173 = Enqueue Element(queue=w347, element=w346) -> (queue out=w348:refnum<queue>)  [unwired: 2 in, 2 out]
                }
              }
              frame "Start Task 4" {
                n174 = for {
                  shift-right: [w355] -> w350
                  shift-left: w351 -> [w354]
                  tunnel: string[] ["RESET YAW", "RESET ENCODERS", "RESET ARM", "RESET FLAGS", "", ""] -> [w353] mode=indexing
                  n175 = Enqueue Element(queue=w354, element=w353) -> (queue out=w355:refnum<queue>)  [unwired: 2 in, 2 out]
                }
              }
              frame "Start Task 5" {
                n176 = for {
                  shift-right: [w362] -> w357
                  shift-left: w358 -> [w361]
                  tunnel: string[] ["RESET YAW", "RESET ENCODERS", "READ STEPPER VALUES", "Z STEPPER CAM HEIGHT", "", ""] -> [w360] mode=indexing
                  n177 = Enqueue Element(queue=w361, element=w360) -> (queue out=w362:refnum<queue>)  [unwired: 2 in, 2 out]
                }
              }
              frame "Start Task 6" {
                n178 = for {
                  shift-right: [w369] -> w364
                  shift-left: w365 -> [w368]
                  tunnel: string[] ["OPEN LOG CAM ", "", "", "", "", ""] -> [w367] mode=indexing
                  n179 = Enqueue Element(queue=w368, element=w367) -> (queue out=w369:refnum<queue>)  [unwired: 2 in, 2 out]
                }
              }
              frame "None", Default {
              }
              frame "Exit" {
                n180 = for {
                  shift-right: [w378] -> w373
                  shift-left: w374 -> [w377]
                  tunnel: string[] ["STOP", "RESET ENCODERS", "RESET YAW", "EXIT"] -> [w376] mode=indexing
                  n181 = Enqueue Element(queue=w377, element=w376) -> (queue out=w378:refnum<queue>)  [unwired: 2 in, 2 out]
                }
              }
              frame "Start Task 9" {
                n182 = for {
                  shift-right: [w385] -> w381
                  shift-left: w380 -> [w384]
                  tunnel: string[] ["RESET ENCODERS", "READ ENCODERS", "Z STEPPER CAM HEIGHT"] -> [w383] mode=indexing
                  n183 = Enqueue Element(queue=w384, element=w383) -> (queue out=w385:refnum<queue>)  [unwired: 2 in, 2 out]
                }
              }
              frame "Start Task 8 - BALL" {
                n184 = for {
                  shift-right: [w392] -> w387
                  shift-left: w388 -> [w391]
                  tunnel: string[] ["RESET YAW", "RESET ENCODERS", "RESET ARM", "RESET FLAGS"] -> [w390] mode=indexing
                  n185 = Enqueue Element(queue=w391, element=w390) -> (queue out=w392:refnum<queue>)  [unwired: 2 in, 2 out]
                }
              }
            }
          }
          frame 5 {
            # ">>> yStepper command>>>"
            n186 = for {
              shift-right: [w401] -> w395
              shift-left: w397 -> [w400]
              tunnel: string[] ["INIT", "RESET ENCODERS", "RESET FLAGS", "CAM CLOSE", "DISPOSE BUFFERS", "EXIT", ""] -> [w399] mode=indexing
              n187 = Enqueue Element(queue=w400, element=w399) -> (queue out=w401:refnum<queue>)  [unwired: 2 in, 2 out]
            }
          }
          frame 6 {
            # ">>> yStepper command>>>"
            # "Use 250"
            n188 = Dequeue Element(queue=w415, timeout in ms (-1)=w414, error in (no error)=w413) -> (element=w412:T7)  [unwired: 3 out]
            n189 = Greater?(x=w406, y=265.0) -> (0:w404:bool)
            n190 = Or(x=w404, y=w407) -> (x .or. y?=w411:bool)
            n191 = case shown="\"None\", Default" w412 {
              tunnel: w411 -> [w418 _]
              tunnel: [w422 State_Type_Definitions,_for_0.26g_versions_and_later_2."True Stop" ("Enum")] -> w410
              tunnel: w409 -> [w419 w437]
              tunnel: [w417 w436] -> w408
              tunnel: [State_Type_Definitions,_for_0.26g_versions_and_later_2."Idle" ("Enum") State_Type_Definitions,_for_0.26g_versions_and_later_2."Shutdown" ("Enum")] -> w403
              frame "None", Default {
                n192 = case shown="True" w418 {
                  tunnel: w419 -> [w425 w431]
                  tunnel: [w424 w429] -> w417
                  frame False {
                    n193 = for {
                      shift-right: [w427] -> w424
                      shift-left: w425 -> [w428]
                      tunnel: string[] ["READ ENCODERS", "READ NAVX", "FORWARD"] ("element") -> [w426] mode=indexing
                      n194 = Enqueue Element(queue=w428, element=w426) -> (queue out=w427:refnum<queue>)  [unwired: 2 in, 2 out]
                    }
                  }
                  frame True {
                    n195 = for {
                      shift-right: [w433] -> w429
                      shift-left: w431 -> [w434]
                      tunnel: string[] ["RESET YAW", "RESET ENCODERS", "STOP", ""] -> [w432] mode=indexing
                      n196 = Enqueue Element(queue=w434, element=w432) -> (queue out=w433:refnum<queue>)  [unwired: 2 in, 2 out]
                    }
                  }
                }
                n197 = Select(t=State_Type_Definitions,_for_0.26g_versions_and_later_2."True Stop" ("Enum"), s=w418, f=State_Type_Definitions."Task 1" ("Enum")) -> (s? t:f=w422:u16)
              }
              frame "Exit" {
                n198 = for {
                  shift-right: [w441] -> w436
                  shift-left: w437 -> [w442]
                  tunnel: string[] ["STOP", "RESET ENCODERS", "RESET YAW", ""] -> [w440] mode=indexing
                  n199 = Enqueue Element(queue=w442, element=w440) -> (queue out=w441:refnum<queue>)  [unwired: 2 in, 2 out]
                }
              }
            }
          }
          frame 8 {
            # ">> Stepper height reeached >>"
            # ">>> yStepper command>>>"
            # ">> Manual override >>"
            n200 = Dequeue Element(queue=w446, timeout in ms (-1)=w445, error in (no error)=w444) -> (element=w455:T7)  [unwired: 3 out]
            n201 = Equal?(x=w448, y=u8 60) -> (x = y?=w453:bool)
            n202 = case shown="\"None\", Default" w455 {
              tunnel: [w466 State_Type_Definitions,_for_0.26g_versions_and_later_2."True Stop" ("Enum")] -> w450
              tunnel: [w464 w481] -> w443
              tunnel: w452 -> [w463 _]
              tunnel: w451 -> [w457 _]
              tunnel: [State_Type_Definitions,_for_0.26g_versions_and_later_2."Idle" ("Enum") State_Type_Definitions,_for_0.26g_versions_and_later_2."Shutdown" ("Enum")] -> w449
              tunnel: w453 -> [w456 _]
              frame "None", Default {
                # ">> WIill proceed to part ii if not manual override >>"
                # ">>If ENABLE or Trigger is set to true>>"
                n203 = Or(x=w456, y=w457) -> (x .or. y?=w458:bool)
                n204 = case shown="True" w456 {
                  tunnel: [w469 w475] -> w464
                  tunnel: w463 -> [w468 w474]
                  frame False {
                    n205 = for {
                      shift-right: [w471] -> w469
                      shift-left: w468 -> [w472]
                      tunnel: string[] ["Z STEPPER CAM HEIGHT", "READ STEPPER VALUES"] ("element") -> [w470] mode=indexing
                      n206 = Enqueue Element(queue=w472, element=w470) -> (queue out=w471:refnum<queue>)  [unwired: 2 in, 2 out]
                    }
                  }
                  frame True {
                    n207 = for {
                      shift-right: [w477] -> w475
                      shift-left: w474 -> [w478]
                      tunnel: string[] ["ARDUINO - ULTRASONIC", "READ ULTRASONIC", "", "", "", ""] -> [w476] mode=indexing
                      n208 = Enqueue Element(queue=w478, element=w476) -> (queue out=w477:refnum<queue>)  [unwired: 2 in, 2 out]
                    }
                  }
                }
                n209 = Select(t=State_Type_Definitions,_for_0.26g_versions_and_later_2."True Stop" ("Enum"), s=w457, f=State_Type_Definitions,_for_0.26g_versions_and_later_2."Task 2:Sensor Mode" ("Enum")) -> (s? t:f=w460:T6)
                n210 = Select(t=w460, s=w458, f=State_Type_Definitions,_for_0.26g_versions_and_later_2."Task 2:Raise Arm" ("Enum")) -> (s? t:f=w466:T6)
              }
              frame "Exit" {
                n211 = for {
                  shift-right: [w484] -> w481
                  shift-left: _ -> [w485]
                  tunnel: string[] ["STOP", "RESET ENCODERS", "RESET YAW", ""] -> [w483] mode=indexing
                  n212 = Enqueue Element(queue=w485, element=w483) -> (queue out=w484:refnum<queue>)  [unwired: 2 in, 2 out]
                }
              }
            }
          }
          frame 9 {
            w500 = u8 20 ("y")
            # ">>> yStepper command>>>"
            # ">>Object detected>>"
            n213 = Dequeue Element(queue=w492, timeout in ms (-1)=w491, error in (no error)=w490) -> (element=w501:T7)  [unwired: 3 out]
            n214 = Less?(x=w488, y=w500) -> (x < y?=w499:bool)
            n215 = Less?(x=w487, y=w500) -> (x < y?=w498:bool)
            n216 = Or(x=w499, y=w498) -> (x .or. y?=w497:bool)
            "Obstacle detected" <- w497
            n217 = case shown="\"None\", Default" w501 {
              tunnel: w497 -> [w504 _]
              tunnel: [w511 State_Type_Definitions,_for_0.26g_versions_and_later_2."True Stop" ("Enum")] -> w496
              tunnel: w489 -> [w503 _]
              tunnel: w493 -> [w510 w527]
              tunnel: [w509 w528] -> w495
              tunnel: [State_Type_Definitions,_for_0.26g_versions_and_later_2."Idle" ("Enum") State_Type_Definitions,_for_0.26g_versions_and_later_2."Shutdown" ("Enum")] -> w494
              frame "None", Default {
                n218 = case shown="True" w504 {
                  tunnel: w510 -> [w514 w521]
                  tunnel: [w515 w520] -> w509
                  frame False {
                    n219 = for {
                      tunnel: string[] ["READ ULTRASONIC", "STOP"] ("element") -> [w516] mode=indexing
                      shift-right: [w518] -> w515
                      shift-left: w514 -> [w517]
                      n220 = Enqueue Element(queue=w517, element=w516) -> (queue out=w518:refnum<queue>)  [unwired: 2 in, 2 out]
                    }
                  }
                  frame True {
                    n221 = for {
                      shift-right: [w523] -> w520
                      shift-left: w521 -> [w524]
                      tunnel: string[] ["RESET ENCODERS", "READ NAVX", "READ ENCODERS"] -> [w522] mode=indexing
                      n222 = Enqueue Element(queue=w524, element=w522) -> (queue out=w523:refnum<queue>)  [unwired: 2 in, 2 out]
                    }
                  }
                }
                n223 = Or(x=w504, y=w503) -> (x .or. y?=w502:bool)
                n224 = Select(t=State_Type_Definitions,_for_0.26g_versions_and_later_2."True Stop" ("Enum"), s=w503, f=State_Type_Definitions,_for_0.26g_versions_and_later_2."Task 2:Reverse Mode" ("Enum")) -> (s? t:f=w505:T6)
                n225 = Select(t=w505, s=w502, f=State_Type_Definitions,_for_0.26g_versions_and_later_2."Task 2:Sensor Mode" ("Enum")) -> (s? t:f=w511:T6)
              }
              frame "Exit" {
                n226 = for {
                  shift-right: [w531] -> w528
                  shift-left: w527 -> [w532]
                  tunnel: string[] ["STOP", "RESET ENCODERS", "RESET YAW", "ARDUINO MODE 0"] -> [w530] mode=indexing
                  n227 = Enqueue Element(queue=w532, element=w530) -> (queue out=w531:refnum<queue>)  [unwired: 2 in, 2 out]
                }
              }
            }
          }
          frame 10 {
            # ">>> yStepper command>>>"
            n228 = Dequeue Element(queue=w541, timeout in ms (-1)=w542, error in (no error)=w543) -> (element=w545:T7)  [unwired: 3 out]
            n229 = Less?(x=w535, y=-50.0) -> (x < y?=w533:bool)
            n230 = case shown="\"None\", Default" w545 {
              tunnel: [w555 State_Type_Definitions,_for_0.26g_versions_and_later_2."True Stop" ("Enum")] -> w537
              tunnel: w544 -> [w548 _]
              tunnel: w540 -> [w554 w571]
              tunnel: [w553 w572] -> w536
              tunnel: [State_Type_Definitions,_for_0.26g_versions_and_later_2."Idle" ("Enum") State_Type_Definitions,_for_0.26g_versions_and_later_2."Shutdown" ("Enum")] -> w538
              tunnel: w533 -> [w546 _]
              frame "None", Default {
                n231 = case shown="False" w546 {
                  tunnel: w554 -> [w558 w565]
                  tunnel: [w559 w564] -> w553
                  frame False {
                    n232 = for {
                      tunnel: string[] ["READ ENCODERS", "REVERSE", "READ NAVX"] ("element") -> [w560] mode=indexing
                      shift-right: [w562] -> w559
                      shift-left: w558 -> [w561]
                      n233 = Enqueue Element(queue=w561, element=w560) -> (queue out=w562:refnum<queue>)  [unwired: 2 in, 2 out]
                    }
                  }
                  frame True {
                    n234 = for {
                      shift-right: [w567] -> w564
                      shift-left: w565 -> [w568]
                      tunnel: string[] ["STOP", "ARDUINO - ULTRASONIC", "READ ULTRASONIC", "RESET ENCODERS"] -> [w566] mode=indexing
                      n235 = Enqueue Element(queue=w568, element=w566) -> (queue out=w567:refnum<queue>)  [unwired: 2 in, 2 out]
                    }
                  }
                }
                n236 = Or(x=w546, y=w548) -> (x .or. y?=w547:bool)
                n237 = Select(t=State_Type_Definitions,_for_0.26g_versions_and_later_2."True Stop" ("Enum"), s=w548, f=State_Type_Definitions,_for_0.26g_versions_and_later_2."Task 2:Sensor Mode" ("Enum")) -> (s? t:f=w549:T6)
                n238 = Select(t=w549, s=w547, f=State_Type_Definitions,_for_0.26g_versions_and_later_2."Task 2:Reverse Mode" ("Enum")) -> (s? t:f=w555:T6)
              }
              frame "Exit" {
                n239 = for {
                  shift-right: [w575] -> w572
                  shift-left: w571 -> [w576]
                  tunnel: string[] ["STOP", "RESET ENCODERS", "RESET YAW", "ARDUINO MODE 0"] -> [w574] mode=indexing
                  n240 = Enqueue Element(queue=w576, element=w574) -> (queue out=w575:refnum<queue>)  [unwired: 2 in, 2 out]
                }
              }
            }
          }
          frame 11 {
            # ">>> yStepper command>>>"
            n241 = Dequeue Element(queue=w590, timeout in ms (-1)=w589, error in (no error)=w588) -> (element=w579:T7)  [unwired: 3 out]
            n242 = Greater?(x=w587, y=160.0) -> (0:w584:bool)
            n243 = Or(x=w584, y=w585) -> (x .or. y?=w580:bool)
            n244 = case shown="\"None\", Default" w579 {
              tunnel: w580 -> [w593 _]
              tunnel: [w597 State_Type_Definitions,_for_0.26g_versions_and_later_2."True Stop" ("Enum")] -> w581
              tunnel: w583 -> [w594 w613]
              tunnel: [w592 w612] -> w582
              tunnel: [State_Type_Definitions,_for_0.26g_versions_and_later_2."Idle" ("Enum") State_Type_Definitions,_for_0.26g_versions_and_later_2."Shutdown" ("Enum")] -> w578
              frame "None", Default {
                n245 = case shown="False" w593 {
                  tunnel: w594 -> [w600 w606]
                  tunnel: [w599 w604] -> w592
                  frame False {
                    n246 = for {
                      shift-right: [w602] -> w599
                      shift-left: w600 -> [w603]
                      tunnel: string[] ["READ ENCODERS", "R-CW"] ("element") -> [w601] mode=indexing
                      n247 = Enqueue Element(queue=w603, element=w601) -> (queue out=w602:refnum<queue>)  [unwired: 2 in, 2 out]
                    }
                  }
                  frame True {
                    n248 = for {
                      shift-right: [w608] -> w604
                      shift-left: w606 -> [w609]
                      tunnel: string[] ["RESET YAW", "RESET ENCODERS", "STOP", "ARDUINO MODE 0"] -> [w607] mode=indexing
                      n249 = Enqueue Element(queue=w609, element=w607) -> (queue out=w608:refnum<queue>)  [unwired: 2 in, 2 out]
                    }
                  }
                }
                n250 = Select(t=State_Type_Definitions,_for_0.26g_versions_and_later_2."True Stop" ("Enum"), s=w593, f=State_Type_Definitions,_for_0.26g_versions_and_later_2."Task 3" ("Enum")) -> (s? t:f=w597:T6)
              }
              frame "Exit" {
                n251 = for {
                  shift-right: [w616] -> w612
                  shift-left: w613 -> [w617]
                  tunnel: string[] ["STOP", "RESET ENCODERS", "RESET YAW", ""] -> [w615] mode=indexing
                  n252 = Enqueue Element(queue=w617, element=w615) -> (queue out=w616:refnum<queue>)  [unwired: 2 in, 2 out]
                }
              }
            }
          }
          frame 12 {
            # ">> Stepper height reeached >>"
            # ">>> yStepper command>>>"
            # ">> Manual override >>"
            n253 = Dequeue Element(queue=w629, timeout in ms (-1)=w628, error in (no error)=w627) -> (element=w626:T7)  [unwired: 3 out]
            n254 = Equal?(x=w620, y=u8 60) -> (x = y?=w618:bool)
            n255 = case shown="\"Exit\"" w626 {
              tunnel: [w641 State_Type_Definitions,_for_0.26g_versions_and_later_2."True Stop" ("Enum")] -> w625
              tunnel: [w639 w657] -> w624
              tunnel: w630 -> [w638 w654]
              tunnel: w623 -> [w632 _]
              tunnel: [State_Type_Definitions,_for_0.26g_versions_and_later_2."Idle" ("Enum") State_Type_Definitions,_for_0.26g_versions_and_later_2."Shutdown" ("Enum")] -> w622
              tunnel: w618 -> [w631 _]
              frame "None", Default {
                # ">> WIill proceed to part ii if not manual override >>"
                # ">>If ENABLE or Trigger is set to true>>"
                n256 = Or(x=w631, y=w632) -> (x .or. y?=w633:bool)
                n257 = case shown="False" w631 {
                  tunnel: [w644 w650] -> w639
                  tunnel: w638 -> [w643 w649]
                  frame False {
                    n258 = for {
                      shift-right: [w646] -> w644
                      shift-left: w643 -> [w647]
                      tunnel: string[] ["Z STEPPER CAM HEIGHT", "READ STEPPER VALUES"] ("element") -> [w645] mode=indexing
                      n259 = Enqueue Element(queue=w647, element=w645) -> (queue out=w646:refnum<queue>)  [unwired: 2 in, 2 out]
                    }
                  }
                  frame True {
                    n260 = for {
                      shift-right: [w652] -> w650
                      shift-left: w649 -> [w653]
                      tunnel: string[] ["ARDUINO - ULTRASONIC", "READ ULTRASONIC", "FORWARD", "", "", ""] -> [w651] mode=indexing
                      n261 = Enqueue Element(queue=w653, element=w651) -> (queue out=w652:refnum<queue>)  [unwired: 2 in, 2 out]
                    }
                  }
                }
                n262 = Select(t=State_Type_Definitions,_for_0.26g_versions_and_later_2."True Stop" ("Enum"), s=w632, f=State_Type_Definitions,_for_0.26g_versions_and_later_2."Task 4_B" ("Enum")) -> (s? t:f=w635:T6)
                n263 = Select(t=w635, s=w633, f=State_Type_Definitions,_for_0.26g_versions_and_later_2."Task 4_A" ("Enum")) -> (s? t:f=w641:T6)
              }
              frame "Exit" {
                n264 = for {
                  shift-right: [w660] -> w657
                  shift-left: w654 -> [w661]
                  tunnel: string[] ["STOP", "RESET ENCODERS", "RESET YAW", ""] -> [w659] mode=indexing
                  n265 = Enqueue Element(queue=w661, element=w659) -> (queue out=w660:refnum<queue>)  [unwired: 2 in, 2 out]
                }
              }
            }
          }
          frame 13 {
            w665 = u8 20
            # ">> Path blocked >>"
            # ">>> yStepper command>>>"
            # ">> Manual override >>"
            n266 = Dequeue Element(queue=w674, timeout in ms (-1)=w673, error in (no error)=w672) -> (element=w671:T7)  [unwired: 3 out]
            n267 = Less?(x=w667, y=w665) -> (x < y?=w662:bool)
            n268 = Less?(x=w666, y=w665) -> (x < y?=w663:bool)
            n269 = And(x=w663, y=w662) -> (x .and. y?=w664:bool)
            n270 = case shown="\"None\", Default" w671 {
              tunnel: [w688 State_Type_Definitions,_for_0.26g_versions_and_later_2."True Stop" ("Enum")] -> w676
              tunnel: [w686 w703] -> w677
              tunnel: w670 -> [w685 _]
              tunnel: w675 -> [w679 _]
              tunnel: [State_Type_Definitions,_for_0.26g_versions_and_later_2."Idle" ("Enum") State_Type_Definitions,_for_0.26g_versions_and_later_2."Shutdown" ("Enum")] -> w669
              tunnel: w664 -> [w678 _]
              frame "None", Default {
                # ">> Manual override forces program to true stop >>"
                # ">>If ENABLE or Trigger is set to true>>"
                n271 = Or(x=w678, y=w679) -> (x .or. y?=w684:bool)
                n272 = case shown="True" w678 {
                  tunnel: [w691 w696] -> w686
                  tunnel: w685 -> [w690 w695]
                  frame False {
                    n273 = for {
                      shift-right: [w693] -> w691
                      shift-left: w690 -> [w694]
                      tunnel: string[] ["FORWARD", "READ ULTRASONIC", "READ NAVX"] ("element") -> [w692] mode=indexing
                      n274 = Enqueue Element(queue=w694, element=w692) -> (queue out=w693:refnum<queue>)  [unwired: 2 in, 2 out]
                    }
                  }
                  frame True {
                    n275 = for {
                      shift-right: [w699] -> w696
                      shift-left: w695 -> [w700]
                      tunnel: string[] ["STOP", "RESET YAW", "RESET ENCODERS", "RESET FLAGS"] -> [w698] mode=indexing
                      n276 = Enqueue Element(queue=w700, element=w698) -> (queue out=w699:refnum<queue>)  [unwired: 2 in, 2 out]
                    }
                  }
                }
                n277 = Select(t=State_Type_Definitions,_for_0.26g_versions_and_later_2."True Stop" ("Enum"), s=w679, f=State_Type_Definitions,_for_0.26g_versions_and_later_2."Task 4_C" ("Enum")) -> (s? t:f=w681:T6)
                n278 = Select(t=w681, s=w684, f=State_Type_Definitions,_for_0.26g_versions_and_later_2."Task 4_B" ("Enum")) -> (s? t:f=w688:T6)
              }
              frame "Exit" {
                n279 = for {
                  shift-right: [w706] -> w703
                  shift-left: _ -> [w707]
                  tunnel: string[] ["STOP", "RESET ENCODERS", "RESET YAW", ""] -> [w705] mode=indexing
                  n280 = Enqueue Element(queue=w707, element=w705) -> (queue out=w706:refnum<queue>)  [unwired: 2 in, 2 out]
                }
              }
            }
          }
          frame 14 {
            w717 = u8 20
            # ">> xDistance travelled>>"
            # ">> Path NOT blocked >>"
            # ">>> yStepper command>>>"
            # ">> Manual override >>"
            n281 = Dequeue Element(queue=w727, timeout in ms (-1)=w720, error in (no error)=w719) -> (element=w721:T7)  [unwired: 3 out]
            n282 = Greater?(x=w709, y=w717) -> (0:w715:bool)
            n283 = Greater?(x=w714, y=80.0) -> (0:w712:bool)
            n284 = Greater?(x=w708, y=w717) -> (0:w716:bool)
            n285 = And(x=w716, y=w715) -> (x .and. y?=w711:bool)
            n286 = And(x=w712, y=w711) -> (x .and. y?=w710:bool)
            n287 = case shown="\"None\", Default" w721 {
              tunnel: [w738 State_Type_Definitions,_for_0.26g_versions_and_later_2."True Stop" ("Enum")] -> w724
              tunnel: [w736 w754] -> w723
              tunnel: w726 -> [w735 w751]
              tunnel: w725 -> [w729 _]
              tunnel: [State_Type_Definitions,_for_0.26g_versions_and_later_2."Idle" ("t") State_Type_Definitions,_for_0.26g_versions_and_later_2."Shutdown" ("Enum")] -> w722
              tunnel: w710 -> [w728 _]
              frame "None", Default {
                # ">> Manual override forces program to true stop >>"
                # ">>If ENABLE or Trigger is set to true>>"
                n288 = Or(x=w728, y=w729) -> (x .or. y?=w734:bool)
                n289 = case shown="False" w728 {
                  tunnel: [w741 w746] -> w736
                  tunnel: w735 -> [w739 w745]
                  frame False {
                    n290 = for {
                      shift-right: [w743] -> w741
                      shift-left: w739 -> [w744]
                      tunnel: string[] ["RIGHT", "READ NAVX", "READ ENCODERS", "READ ULTRASONIC"] ("element") -> [w742] mode=indexing
                      n291 = Enqueue Element(queue=w744, element=w742) -> (queue out=w743:refnum<queue>)  [unwired: 2 in, 2 out]
                    }
                  }
                  frame True {
                    n292 = for {
                      shift-right: [w749] -> w746
                      shift-left: w745 -> [w750]
                      tunnel: string[] ["STOP", "RESET YAW", "RESET ENCODERS", "ARDUINO - ULTRASONIC"] -> [w748] mode=indexing
                      n293 = Enqueue Element(queue=w750, element=w748) -> (queue out=w749:refnum<queue>)  [unwired: 2 in, 2 out]
                    }
                  }
                }
                n294 = Select(t=State_Type_Definitions,_for_0.26g_versions_and_later_2."True Stop" ("Enum"), s=w729, f=State_Type_Definitions,_for_0.26g_versions_and_later_2."Task 4_D" ("Enum")) -> (s? t:f=w730:T6)
                n295 = Select(t=w730, s=w734, f=State_Type_Definitions,_for_0.26g_versions_and_later_2."Task 4_C" ("Enum")) -> (s? t:f=w738:T6)
              }
              frame "Exit" {
                n296 = for {
                  shift-right: [w757] -> w754
                  shift-left: w751 -> [w758]
                  tunnel: string[] ["STOP", "RESET ENCODERS", "RESET YAW", ""] -> [w756] mode=indexing
                  n297 = Enqueue Element(queue=w758, element=w756) -> (queue out=w757:refnum<queue>)  [unwired: 2 in, 2 out]
                }
              }
            }
          }
          frame 15 {
            w777 = u8 20
            # ">> yDistance travelled>>"
            # ">> Path blocked >>"
            # ">>> yStepper command>>>"
            # ">> Manual override >>"
            n298 = Dequeue Element(queue=w768, timeout in ms (-1)=w767, error in (no error)=w766) -> (element=w778:T7)  [unwired: 3 out]
            n299 = Less?(x=w761, y=w777) -> (x < y?=w775:bool)
            n300 = Greater?(x=w765, y=200.0) -> (0:w773:bool)
            n301 = Less?(x=w760, y=w777) -> (x < y?=w776:bool)
            n302 = And(x=w776, y=w775) -> (x .and. y?=w772:bool)
            n303 = Or(x=w773, y=w772) -> (x .or. y?=w771:bool)
            n304 = case shown="\"None\", Default" w778 {
              tunnel: [w789 State_Type_Definitions,_for_0.26g_versions_and_later_2."True Stop" ("Enum")] -> w764
              tunnel: [w787 w805] -> w762
              tunnel: w769 -> [w786 w802]
              tunnel: w770 -> [w780 _]
              tunnel: [State_Type_Definitions,_for_0.26g_versions_and_later_2."Idle" ("t") State_Type_Definitions,_for_0.26g_versions_and_later_2."Shutdown" ("Enum")] -> w763
              tunnel: w771 -> [w779 _]
              frame "None", Default {
                # ">> Manual override forces program to true stop >>"
                # ">>If ENABLE or Trigger is set to true>>"
                n305 = Or(x=w779, y=w780) -> (x .or. y?=w785:bool)
                n306 = case shown="True" w779 {
                  tunnel: [w792 w797] -> w787
                  tunnel: w786 -> [w790 w796]
                  frame False {
                    n307 = for {
                      shift-right: [w794] -> w792
                      shift-left: w790 -> [w795]
                      tunnel: string[] ["FORWARD", "READ NAVX", "READ ENCODERS", "READ ULTRASONIC"] ("element") -> [w793] mode=indexing
                      n308 = Enqueue Element(queue=w795, element=w793) -> (queue out=w794:refnum<queue>)  [unwired: 2 in, 2 out]
                    }
                  }
                  frame True {
                    n309 = for {
                      shift-right: [w800] -> w797
                      shift-left: w796 -> [w801]
                      tunnel: string[] ["STOP", "RESET YAW", "RESET ENCODERS", "RESET FLAGS"] -> [w799] mode=indexing
                      n310 = Enqueue Element(queue=w801, element=w799) -> (queue out=w800:refnum<queue>)  [unwired: 2 in, 2 out]
                    }
                  }
                }
                n311 = Select(t=State_Type_Definitions,_for_0.26g_versions_and_later_2."True Stop" ("Enum"), s=w780, f=State_Type_Definitions,_for_0.26g_versions_and_later_2."True Stop" ("Enum")) -> (s? t:f=w781:T6)
                n312 = Select(t=w781, s=w785, f=State_Type_Definitions,_for_0.26g_versions_and_later_2."Task 4_D" ("Enum")) -> (s? t:f=w789:T6)
              }
              frame "Exit" {
                n313 = for {
                  shift-right: [w808] -> w805
                  shift-left: w802 -> [w809]
                  tunnel: string[] ["STOP", "RESET ENCODERS", "RESET YAW", ""] -> [w807] mode=indexing
                  n314 = Enqueue Element(queue=w809, element=w807) -> (queue out=w808:refnum<queue>)  [unwired: 2 in, 2 out]
                }
              }
            }
          }
          frame 15 {
            # ">>> yStepper command>>>"
            # ">> Manual override >>"
            n315 = Dequeue Element(queue=w818, timeout in ms (-1)=w817, error in (no error)=w819) -> (element=w816:T7)  [unwired: 3 out]
            n316 = Equal?(x=w815, y=u8 60) -> (x = y?=w813:bool)
            n317 = case shown="\"None\", Default" w816 {
              tunnel: [w829 State_Type_Definitions,_for_0.26g_versions_and_later_2."True Stop" ("Enum")] -> w820
              tunnel: [w832 w849] -> w821
              tunnel: [State_Type_Definitions,_for_0.26g_versions_and_later_2."Idle" ("Enum") State_Type_Definitions,_for_0.26g_versions_and_later_2."Shutdown" ("Enum")] -> w822
              tunnel: w813 -> [w828 _]
              tunnel: w812 -> [w827 _]
              tunnel: w811 -> [w823 w846]
              frame "None", Default {
                # "Stays in Task 5_A until stepper reaches desired \nheight"
                # "T: Go back to idle, F: Continue with task\""
                # ">> Manual override >>"
                n318 = case shown="True" w828 {
                  tunnel: [w836 w842] -> w832
                  tunnel: w823 -> [w834 w840]
                  frame False {
                    n319 = for {
                      tunnel: string[] ["Z STEPPER CAM HEIGHT", "READ STEPPER VALUES"] ("element") -> [w837] mode=indexing
                      shift-right: [w839] -> w836
                      shift-left: w834 -> [w838]
                      n320 = Enqueue Element(queue=w838, element=w837) -> (queue out=w839:refnum<queue>)  [unwired: 2 in, 2 out]
                    }
                  }
                  frame True {
                    n321 = for {
                      shift-right: [w844] -> w842
                      shift-left: w840 -> [w845]
                      tunnel: string[] ["ARDUINO - ULTRASONIC", "READ ULTRASONIC", ""] -> [w843] mode=indexing
                      n322 = Enqueue Element(queue=w845, element=w843) -> (queue out=w844:refnum<queue>)  [unwired: 2 in, 2 out]
                    }
                  }
                }
                n323 = Or(x=w828, y=w827) -> (x .or. y?=w830:bool)
                n324 = Select(t=State_Type_Definitions,_for_0.26g_versions_and_later_2."True Stop" ("Enum"), s=w827, f=State_Type_Definitions."Task 5B: MOVE TO BOX" ("Enum")) -> (s? t:f=w824:u16)
                n325 = Select(t=w824, s=w830, f=State_Type_Definitions."Task 5A: ARM CAM HEIGHT" ("Enum")) -> (s? t:f=w829:u16)
              }
              frame "Exit" {
                n326 = for {
                  shift-right: [w852] -> w849
                  shift-left: w846 -> [w853]
                  tunnel: string[] ["STOP", "RESET ENCODERS", "RESET YAW", "ARDUINO MODE 0"] -> [w851] mode=indexing
                  n327 = Enqueue Element(queue=w853, element=w851) -> (queue out=w852:refnum<queue>)  [unwired: 2 in, 2 out]
                }
              }
            }
          }
          frame 16 {
            w859 = u8 20 ("y")
            # ">>> yStepper command>>>"
            n328 = Less?(x=w856, y=w859) -> (x < y?=w857:bool)
            n329 = Dequeue Element(queue=w863, timeout in ms (-1)=w862, error in (no error)=w864) -> (element=w861:T7)  [unwired: 3 out]
            n330 = Less?(x=w855, y=w859) -> (x < y?=w858:bool)
            n331 = And(x=w858, y=w857) -> (x .and. y?=w854:bool)
            n332 = case shown="\"None\", Default" w861 {
              tunnel: [w876 State_Type_Definitions,_for_0.26g_versions_and_later_2."True Stop" ("Enum")] -> w866
              tunnel: [w879 w896] -> w865
              tunnel: [State_Type_Definitions,_for_0.26g_versions_and_later_2."Idle" ("Enum") State_Type_Definitions,_for_0.26g_versions_and_later_2."Shutdown" ("Enum")] -> w867
              tunnel: w869 -> [w875 _]
              tunnel: w868 -> [w871 w893]
              tunnel: w854 -> [w870 _]
              frame "None", Default {
                # "Stays in Task 5_B to capture image over 5 seconds"
                # "T: Go back to idle, F: Continue with task\""
                # ">> Manual override >>"
                n333 = case shown="True" w870 {
                  tunnel: [w883 w889] -> w879
                  tunnel: w871 -> [w881 w887]
                  frame False {
                    n334 = for {
                      tunnel: string[] ["FORWARD", "READ ULTRASONIC", "READ NAVX"] ("element") -> [w884] mode=indexing
                      shift-right: [w886] -> w883
                      shift-left: w881 -> [w885]
                      n335 = Enqueue Element(queue=w885, element=w884) -> (queue out=w886:refnum<queue>)  [unwired: 2 in, 2 out]
                    }
                  }
                  frame True {
                    n336 = for {
                      shift-right: [w891] -> w889
                      shift-left: w887 -> [w892]
                      tunnel: string[] ["STOP", "RESET ENCODERS", "OPEN LOG CAM", "SET TIMER 5"] -> [w890] mode=indexing
                      n337 = Enqueue Element(queue=w892, element=w890) -> (queue out=w891:refnum<queue>)  [unwired: 2 in, 2 out]
                    }
                  }
                }
                n338 = Or(x=w870, y=w875) -> (x .or. y?=w877:bool)
                n339 = Select(t=State_Type_Definitions,_for_0.26g_versions_and_later_2."True Stop" ("Enum"), s=w875, f=State_Type_Definitions."Task 5C: CAM BURST" ("Enum")) -> (s? t:f=w872:u16)
                n340 = Select(t=w872, s=w877, f=State_Type_Definitions."Task 5B: MOVE TO BOX" ("Enum")) -> (s? t:f=w876:u16)
              }
              frame "Exit" {
                n341 = for {
                  shift-right: [w899] -> w896
                  shift-left: w893 -> [w900]
                  tunnel: string[] ["STOP", "RESET ENCODERS", "RESET YAW", "ARDUINO MODE 0"] -> [w898] mode=indexing
                  n342 = Enqueue Element(queue=w900, element=w898) -> (queue out=w899:refnum<queue>)  [unwired: 2 in, 2 out]
                }
              }
            }
          }
          frame 17 {
            # ">>> yStepper command>>>"
            # ">> Manual override >>"
            n343 = Dequeue Element(queue=w909, timeout in ms (-1)=w908, error in (no error)=w907) -> (element=w906:T7)  [unwired: 3 out]
            n344 = case shown="\"None\", Default" w906 {
              tunnel: [w918 State_Type_Definitions,_for_0.26g_versions_and_later_2."True Stop" ("Enum")] -> w911
              tunnel: [w921 w938] -> w904
              tunnel: [State_Type_Definitions,_for_0.26g_versions_and_later_2."Idle" ("Enum") State_Type_Definitions,_for_0.26g_versions_and_later_2."Shutdown" ("Enum")] -> w903
              tunnel: w905 -> [w912 _]
              tunnel: w910 -> [w917 w935]
              tunnel: w901 -> [w916 _]
              frame "None", Default {
                # ">> Is time up? >>"
                # "Determines if object is in range to pick up"
                # ">> Manual override >>"
                n345 = case shown="True" w916 {
                  tunnel: [w925 w931] -> w921
                  tunnel: w917 -> [w923 w929]
                  frame False {
                    n346 = for {
                      tunnel: string[] ["CAM ACQ", "START TIMER"] ("element") -> [w926] mode=indexing
                      shift-right: [w928] -> w925
                      shift-left: w923 -> [w927]
                      n347 = Enqueue Element(queue=w927, element=w926) -> (queue out=w928:refnum<queue>)  [unwired: 2 in, 2 out]
                    }
                  }
                  frame True {
                    n348 = for {
                      shift-right: [w933] -> w931
                      shift-left: w929 -> [w934]
                      tunnel: string[] ["CAM CLOSE", "PROCESS IMAGE", "SET TIMER 5"] -> [w932] mode=indexing
                      n349 = Enqueue Element(queue=w934, element=w932) -> (queue out=w933:refnum<queue>)  [unwired: 2 in, 2 out]
                    }
                  }
                }
                n350 = Or(x=w916, y=w912) -> (x .or. y?=w919:bool)
                n351 = Select(t=State_Type_Definitions,_for_0.26g_versions_and_later_2."True Stop" ("Enum"), s=w912, f=State_Type_Definitions."Task 5D: PROCESS IMAGE" ("Enum")) -> (s? t:f=w914:u16)
                n352 = Select(t=w914, s=w919, f=State_Type_Definitions."Task 5C: CAM BURST" ("Enum")) -> (s? t:f=w918:u16)
              }
              frame "Exit" {
                n353 = for {
                  shift-right: [w941] -> w938
                  shift-left: w935 -> [w942]
                  tunnel: string[] ["STOP", "RESET ENCODERS", "RESET YAW", "ARDUINO MODE 0"] -> [w940] mode=indexing
                  n354 = Enqueue Element(queue=w942, element=w940) -> (queue out=w941:refnum<queue>)  [unwired: 2 in, 2 out]
                }
              }
            }
          }
          frame 18 {
            # ">>> yStepper command>>>"
            n355 = Dequeue Element(queue=w948, timeout in ms (-1)=w947, error in (no error)=w946) -> (element=w945:T7)  [unwired: 3 out]
            n356 = case shown="\"None\", Default" w945 {
              tunnel: [w960 State_Type_Definitions,_for_0.26g_versions_and_later_2."True Stop" ("Enum")] -> w952
              tunnel: [w963 w980] -> w951
              tunnel: [State_Type_Definitions,_for_0.26g_versions_and_later_2."Idle" ("Enum") State_Type_Definitions,_for_0.26g_versions_and_later_2."Shutdown" ("Enum")] -> w953
              tunnel: w949 -> [w959 _]
              tunnel: w950 -> [w955 w977]
              tunnel: w943 -> [w954 _]
              frame "None", Default {
                # ">> T: Breaks out of state loop; F: Stays in loop>>"
                # ">> Manual override >>"
                # ">> Checks if time is up>>"
                # "Stays in Task 5D until the object is detected"
                # "T: Go back to idle, F: Continue with task\""
                # ">> Manual override >>"
                n357 = case shown="True" w954 {
                  tunnel: [w967 w973] -> w963
                  tunnel: w955 -> [w965 w971]
                  frame False {
                    n358 = for {
                      tunnel: string[] ["START TIMER", "PROCESS IMAGE", ""] ("element") -> [w968] mode=indexing
                      shift-right: [w970] -> w967
                      shift-left: w965 -> [w969]
                      n359 = Enqueue Element(queue=w969, element=w968) -> (queue out=w970:refnum<queue>)  [unwired: 2 in, 2 out]
                    }
                  }
                  frame True {
                    n360 = for {
                      shift-right: [w975] -> w973
                      shift-left: w971 -> [w976]
                      tunnel: string[] ["CAM CLOSE", "", ""] -> [w974] mode=indexing
                      n361 = Enqueue Element(queue=w976, element=w974) -> (queue out=w975:refnum<queue>)  [unwired: 2 in, 2 out]
                    }
                  }
                }
                n362 = Or(x=w954, y=w959) -> (x .or. y?=w961:bool)
                n363 = Select(t=State_Type_Definitions,_for_0.26g_versions_and_later_2."True Stop" ("Enum"), s=w959, f=State_Type_Definitions,_for_0.26g_versions_and_later_2."Task 5E: POSITION ARM" ("Enum")) -> (s? t:f=w956:T6)
                n364 = Select(t=w956, s=w961, f=State_Type_Definitions."Task 5D: PROCESS IMAGE" ("Enum")) -> (s? t:f=w960:u16)
              }
              frame "Exit" {
                n365 = for {
                  shift-right: [w983] -> w980
                  shift-left: w977 -> [w984]
                  tunnel: string[] ["STOP", "RESET ENCODERS", "RESET YAW", "ARDUINO MODE 0"] -> [w982] mode=indexing
                  n366 = Enqueue Element(queue=w984, element=w982) -> (queue out=w983:refnum<queue>)  [unwired: 2 in, 2 out]
                }
              }
            }
          }
          frame 20 {
            # ">>> yStepper command>>>"
            n367 = Dequeue Element(queue=w996, timeout in ms (-1)=w997, error in (no error)=w998) -> (element=w1000:T7)  [unwired: 3 out]
            n368 = formula code="if (pos < 100)\ny = 41;\n\nelse if (pos >= 100 && pos <= 140)\ny = 30;\n\nelse if (pos >= 141 && pos <= 170)\ny = 25;\n\nelse if (pos >= 171 &&pos <= 180) \ny = 20;\n\nelse if (pos >= 181&& pos <= 200)\ny = 15;\n\nelse if (pos >= 201 && pos <= 230)\ny = 10;\n\nelse if (pos >= 231 && pos <= 320)\ny = 8;\n\nelse if (pos > 320)\ny = 0;"("pos"=w988) -> ("y"=w991:dbl)
            n369 = To Unsigned Byte Integer(number=w991) -> (unsigned 8bit integer=w986:u8)
            n370 = Equal?(x=w987, y=w986) -> (x = y?=w985:bool)
            n371 = case shown="\"None\", Default" w1000 {
              tunnel: [w1007 State_Type_Definitions,_for_0.26g_versions_and_later_2."True Stop" ("Enum")] -> w994
              tunnel: [w1010 w1027] -> w992
              tunnel: [State_Type_Definitions,_for_0.26g_versions_and_later_2."Idle" ("Enum") State_Type_Definitions,_for_0.26g_versions_and_later_2."Shutdown" ("Enum")] -> w993
              tunnel: w999 -> [w1006 _]
              tunnel: w995 -> [w1002 w1024]
              tunnel: w985 -> [w1001 _]
              frame "None", Default {
                # ">> T: Breaks out of state loop; F: Stays in loop>>"
                # ">> Manual override >>"
                # ">> Checks if time is up>>"
                # "Stays in Task 5D until the object is detected"
                # "T: Go back to idle, F: Continue with task\""
                # ">> Manual override >>"
                n372 = case shown="False" w1001 {
                  tunnel: [w1014 w1020] -> w1010
                  tunnel: w1002 -> [w1012 w1018]
                  frame False {
                    n373 = for {
                      tunnel: string[] ["READ STEPPER VALUES", "Y STEPPER CONTROL", ""] ("element") -> [w1015] mode=indexing
                      shift-right: [w1017] -> w1014
                      shift-left: w1012 -> [w1016]
                      n374 = Enqueue Element(queue=w1016, element=w1015) -> (queue out=w1017:refnum<queue>)  [unwired: 2 in, 2 out]
                    }
                  }
                  frame True {
                    n375 = for {
                      shift-right: [w1022] -> w1020
                      shift-left: w1018 -> [w1023]
                      tunnel: string[] ["CAM CLOSE", "DISPOSE BUFFERS", ""] -> [w1021] mode=indexing
                      n376 = Enqueue Element(queue=w1023, element=w1021) -> (queue out=w1022:refnum<queue>)  [unwired: 2 in, 2 out]
                    }
                  }
                }
                n377 = Or(x=w1001, y=w1006) -> (x .or. y?=w1008:bool)
                n378 = Select(t=State_Type_Definitions,_for_0.26g_versions_and_later_2."True Stop" ("Enum"), s=w1006, f=State_Type_Definitions,_for_0.26g_versions_and_later_2."Task 5F: ARM GRAB HEIGHT" ("Enum")) -> (s? t:f=w1003:T6)
                n379 = Select(t=w1003, s=w1008, f=State_Type_Definitions,_for_0.26g_versions_and_later_2."Task 5E: POSITION ARM" ("Enum")) -> (s? t:f=w1007:T6)
              }
              frame "Exit" {
                n380 = for {
                  shift-right: [w1030] -> w1027
                  shift-left: w1024 -> [w1031]
                  tunnel: string[] ["STOP", "RESET ENCODERS", "RESET YAW", "ARDUINO MODE 0"] -> [w1029] mode=indexing
                  n381 = Enqueue Element(queue=w1031, element=w1029) -> (queue out=w1030:refnum<queue>)  [unwired: 2 in, 2 out]
                }
              }
            }
            n382 = Bundle By Name(cluster=w990, "yStepper desired"=w986) -> (w989:T9)
          }
          frame 21 {
            # ">>> yStepper command>>>"
            # ">> Manual override >>"
            n383 = Dequeue Element(queue=w1040, timeout in ms (-1)=w1039, error in (no error)=w1041) -> (element=w1038:T7)  [unwired: 3 out]
            n384 = Equal?(x=w1037, y=u8 1) -> (x = y?=w1035:bool)
            n385 = case shown="\"None\", Default" w1038 {
              tunnel: [w1051 State_Type_Definitions,_for_0.26g_versions_and_later_2."True Stop" ("Enum")] -> w1042
              tunnel: [w1054 w1071] -> w1043
              tunnel: [State_Type_Definitions,_for_0.26g_versions_and_later_2."Idle" ("Enum") State_Type_Definitions,_for_0.26g_versions_and_later_2."Shutdown" ("Enum")] -> w1044
              tunnel: w1035 -> [w1050 _]
              tunnel: w1034 -> [w1049 _]
              tunnel: w1033 -> [w1045 w1068]
              frame "None", Default {
                # "Stays in Task 5F until stepper reaches desired \nheight"
                # "T: Go back to idle, F: Continue with task\""
                # ">> Manual override >>"
                n386 = case shown="True" w1050 {
                  tunnel: [w1058 w1064] -> w1054
                  tunnel: w1045 -> [w1056 w1062]
                  frame False {
                    n387 = for {
                      tunnel: string[] ["Z STEPPER GRAB HEIGHT", "READ STEPPER VALUES"] ("element") -> [w1059] mode=indexing
                      shift-right: [w1061] -> w1058
                      shift-left: w1056 -> [w1060]
                      n388 = Enqueue Element(queue=w1060, element=w1059) -> (queue out=w1061:refnum<queue>)  [unwired: 2 in, 2 out]
                    }
                  }
                  frame True {
                    n389 = for {
                      shift-right: [w1066] -> w1064
                      shift-left: w1062 -> [w1067]
                      tunnel: string[] ["SET TIMER 5", "CLOSE CLAW", ""] -> [w1065] mode=indexing
                      n390 = Enqueue Element(queue=w1067, element=w1065) -> (queue out=w1066:refnum<queue>)  [unwired: 2 in, 2 out]
                    }
                  }
                }
                n391 = Or(x=w1050, y=w1049) -> (x .or. y?=w1052:bool)
                n392 = Select(t=State_Type_Definitions,_for_0.26g_versions_and_later_2."True Stop" ("Enum"), s=w1049, f=State_Type_Definitions,_for_0.26g_versions_and_later_2."Task 5G: CLOSE CLAW" ("Enum")) -> (s? t:f=w1046:T6)
                n393 = Select(t=w1046, s=w1052, f=State_Type_Definitions,_for_0.26g_versions_and_later_2."Task 5F: ARM GRAB HEIGHT" ("Enum")) -> (s? t:f=w1051:T6)
              }
              frame "Exit" {
                n394 = for {
                  shift-right: [w1074] -> w1071
                  shift-left: w1068 -> [w1075]
                  tunnel: string[] ["STOP", "RESET ENCODERS", "RESET YAW", "ARDUINO MODE 0"] -> [w1073] mode=indexing
                  n395 = Enqueue Element(queue=w1075, element=w1073) -> (queue out=w1074:refnum<queue>)  [unwired: 2 in, 2 out]
                }
              }
            }
          }
          frame 22 {
            # ">>> yStepper command>>>"
            # ">> Manual override >>"
            n396 = Dequeue Element(queue=w1084, timeout in ms (-1)=w1083, error in (no error)=w1082) -> (element=w1081:T7)  [unwired: 3 out]
            n397 = case shown="\"None\", Default" w1081 {
              tunnel: [w1093 State_Type_Definitions,_for_0.26g_versions_and_later_2."True Stop" ("Enum")] -> w1086
              tunnel: [w1096 w1113] -> w1079
              tunnel: [State_Type_Definitions,_for_0.26g_versions_and_later_2."Idle" ("Enum") State_Type_Definitions,_for_0.26g_versions_and_later_2."Shutdown" ("Enum")] -> w1078
              tunnel: w1080 -> [w1087 _]
              tunnel: w1085 -> [w1092 w1110]
              tunnel: w1076 -> [w1091 _]
              frame "None", Default {
                # ">> Is time up? >>"
                # "Determines if object is in range to pick up"
                # ">> Manual override >>"
                n398 = case shown="True" w1091 {
                  tunnel: [w1100 w1106] -> w1096
                  tunnel: w1092 -> [w1098 w1104]
                  frame False {
                    n399 = for {
                      tunnel: string[] ["CLOSE CLAW", "START TIMER"] ("element") -> [w1101] mode=indexing
                      shift-right: [w1103] -> w1100
                      shift-left: w1098 -> [w1102]
                      n400 = Enqueue Element(queue=w1102, element=w1101) -> (queue out=w1103:refnum<queue>)  [unwired: 2 in, 2 out]
                    }
                  }
                  frame True {
                    n401 = for {
                      shift-right: [w1108] -> w1106
                      shift-left: w1104 -> [w1109]
                      tunnel: string[] ["READ STEPPER VALUES", "", ""] -> [w1107] mode=indexing
                      n402 = Enqueue Element(queue=w1109, element=w1107) -> (queue out=w1108:refnum<queue>)  [unwired: 2 in, 2 out]
                    }
                  }
                }
                n403 = Or(x=w1091, y=w1087) -> (x .or. y?=w1094:bool)
                n404 = Select(t=State_Type_Definitions,_for_0.26g_versions_and_later_2."True Stop" ("Enum"), s=w1087, f=State_Type_Definitions,_for_0.26g_versions_and_later_2."Task 5H: RAISE ARM" ("Enum")) -> (s? t:f=w1089:T6)
                n405 = Select(t=w1089, s=w1094, f=State_Type_Definitions,_for_0.26g_versions_and_later_2."Task 5G: CLOSE CLAW" ("Enum")) -> (s? t:f=w1093:T6)
              }
              frame "Exit" {
                n406 = for {
                  shift-right: [w1116] -> w1113
                  shift-left: w1110 -> [w1117]
                  tunnel: string[] ["STOP", "RESET ENCODERS", "RESET YAW", "ARDUINO MODE 0"] -> [w1115] mode=indexing
                  n407 = Enqueue Element(queue=w1117, element=w1115) -> (queue out=w1116:refnum<queue>)  [unwired: 2 in, 2 out]
                }
              }
            }
          }
          frame 23 {
            # ">>> yStepper command>>>"
            # ">> Manual override >>"
            n408 = Dequeue Element(queue=w1126, timeout in ms (-1)=w1125, error in (no error)=w1127) -> (element=w1124:T7)  [unwired: 3 out]
            n409 = Equal?(x=w1123, y=u8 60) -> (x = y?=w1121:bool)
            n410 = case shown="\"None\", Default" w1124 {
              tunnel: [w1137 State_Type_Definitions,_for_0.26g_versions_and_later_2."True Stop" ("Enum")] -> w1128
              tunnel: [w1140 w1157] -> w1129
              tunnel: [State_Type_Definitions,_for_0.26g_versions_and_later_2."Idle" ("Enum") State_Type_Definitions,_for_0.26g_versions_and_later_2."Shutdown" ("Enum")] -> w1130
              tunnel: w1121 -> [w1136 _]
              tunnel: w1120 -> [w1135 _]
              tunnel: w1119 -> [w1131 w1154]
              frame "None", Default {
                # "Stays in Task 5_A until stepper reaches desired \nheight"
                # "T: Go back to idle, F: Continue with task\""
                # ">> Manual override >>"
                n411 = case shown="False" w1136 {
                  tunnel: [w1144 w1150] -> w1140
                  tunnel: w1131 -> [w1142 w1148]
                  frame False {
                    n412 = for {
                      tunnel: string[] ["Z STEPPER CAM HEIGHT", "READ STEPPER VALUES"] ("element") -> [w1145] mode=indexing
                      shift-right: [w1147] -> w1144
                      shift-left: w1142 -> [w1146]
                      n413 = Enqueue Element(queue=w1146, element=w1145) -> (queue out=w1147:refnum<queue>)  [unwired: 2 in, 2 out]
                    }
                  }
                  frame True {
                    n414 = for {
                      shift-right: [w1152] -> w1150
                      shift-left: w1148 -> [w1153]
                      tunnel: string[] ["ARDUINO - ULTRASONIC", "READ ULTRASONIC", ""] -> [w1151] mode=indexing
                      n415 = Enqueue Element(queue=w1153, element=w1151) -> (queue out=w1152:refnum<queue>)  [unwired: 2 in, 2 out]
                    }
                  }
                }
                n416 = Or(x=w1136, y=w1135) -> (x .or. y?=w1138:bool)
                n417 = Select(t=State_Type_Definitions,_for_0.26g_versions_and_later_2."True Stop" ("Enum"), s=w1135, f=State_Type_Definitions,_for_0.26g_versions_and_later_2."True Stop" ("Enum")) -> (s? t:f=w1132:T6)
                n418 = Select(t=w1132, s=w1138, f=State_Type_Definitions,_for_0.26g_versions_and_later_2."Task 5H: RAISE ARM" ("Enum")) -> (s? t:f=w1137:T6)
              }
              frame "Exit" {
                n419 = for {
                  shift-right: [w1160] -> w1157
                  shift-left: w1154 -> [w1161]
                  tunnel: string[] ["STOP", "RESET ENCODERS", "RESET YAW", "ARDUINO MODE 0"] -> [w1159] mode=indexing
                  n420 = Enqueue Element(queue=w1161, element=w1159) -> (queue out=w1160:refnum<queue>)  [unwired: 2 in, 2 out]
                }
              }
            }
          }
          frame 24 {
            # ">>> yStepper command>>>"
            n421 = Dequeue Element(queue=w1169, timeout in ms (-1)=w1168, error in (no error)=w1167) -> (element=w1174:T7)  [unwired: 3 out]
            n422 = Equal?(x=w1165, y=u8 60) -> (x = y?=w1164:bool)
            n423 = case shown="\"None\", Default" w1174 {
              tunnel: [w1181 State_Type_Definitions,_for_0.26g_versions_and_later_2."True Stop" ("Enum")] -> w1172
              tunnel: [w1180 w1198] -> w1171
              tunnel: [State_Type_Definitions,_for_0.26g_versions_and_later_2."Idle" ("Enum") State_Type_Definitions,_for_0.26g_versions_and_later_2."Shutdown" ("Enum")] -> w1173
              tunnel: w1170 -> [w1176 _]
              tunnel: w1166 -> [w1178 _]
              tunnel: w1164 -> [w1175 _]
              frame "None", Default {
                n424 = case shown="False" w1175 {
                  tunnel: [w1186 w1192] -> w1180
                  tunnel: w1178 -> [w1184 w1190]
                  frame False {
                    n425 = for {
                      tunnel: string[] ["Z STEPPER CAM HEIGHT", "READ STEPPER VALUES"] ("element") -> [w1187] mode=indexing
                      shift-right: [w1189] -> w1186
                      shift-left: w1184 -> [w1188]
                      n426 = Enqueue Element(queue=w1188, element=w1187) -> (queue out=w1189:refnum<queue>)  [unwired: 2 in, 2 out]
                    }
                  }
                  frame True {
                    n427 = for {
                      shift-right: [w1194] -> w1192
                      shift-left: w1190 -> [w1195]
                      tunnel: string[] ["CAM ACQ", "OPEN LOG CAM"] -> [w1193] mode=indexing
                      n428 = Enqueue Element(queue=w1195, element=w1193) -> (queue out=w1194:refnum<queue>)  [unwired: 2 in, 2 out]
                    }
                  }
                }
                n429 = Or(x=w1175, y=w1176) -> (x .or. y?=w1177:bool)
                n430 = Select(t=State_Type_Definitions,_for_0.26g_versions_and_later_2."Task 6_B" ("Enum"), s=w1177, f=State_Type_Definitions,_for_0.26g_versions_and_later_2."Task 6_A" ("Enum")) -> (s? t:f=w1181:T6)
              }
              frame "Exit" {
                n431 = for {
                  shift-right: [w1201] -> w1198
                  shift-left: _ -> [w1202]
                  tunnel: string[] ["STOP", "RESET ENCODERS", "RESET YAW", "ARDUINO MODE 0"] -> [w1200] mode=indexing
                  n432 = Enqueue Element(queue=w1202, element=w1200) -> (queue out=w1201:refnum<queue>)  [unwired: 2 in, 2 out]
                }
              }
            }
          }
          frame 25 {
            # ">>> yStepper command>>>"
            n433 = Dequeue Element(queue=w1212, timeout in ms (-1)=w1210, error in (no error)=w1211) -> (element=w1209:T7)  [unwired: 3 out]
            n434 = case shown="\"None\", Default" w1209 {
              tunnel: [w1219 State_Type_Definitions,_for_0.26g_versions_and_later_2."True Stop" ("Enum")] -> w1205
              tunnel: [w1218 w1237] -> w1213
              tunnel: [State_Type_Definitions,_for_0.26g_versions_and_later_2."Idle" ("Enum") State_Type_Definitions,_for_0.26g_versions_and_later_2."Shutdown" ("Enum")] -> w1206
              tunnel: w1208 -> [w1214 _]
              tunnel: w1207 -> [w1216 _]
              tunnel: w1204 -> [w1215 w1234]
              frame "None", Default {
                # ">> Manual override >>"
                n435 = case shown="True" w1216 {
                  tunnel: [w1224 w1230] -> w1218
                  tunnel: w1215 -> [w1223 w1228]
                  frame False {
                    n436 = for {
                      shift-right: [w1227] -> w1224
                      shift-left: w1223 -> [w1226]
                      tunnel: string[] ["CAM ACQ", "PROCESS IMAGE", "OPEN CLAW"] -> [w1225] mode=indexing
                      n437 = Enqueue Element(queue=w1226, element=w1225) -> (queue out=w1227:refnum<queue>)  [unwired: 2 in, 2 out]
                    }
                  }
                  frame True {
                    n438 = for {
                      shift-right: [w1232] -> w1230
                      shift-left: w1228 -> [w1233]
                      tunnel: string[] ["CAM ACQ", "PROCESS IMAGE", "CLOSE CLAW"] -> [w1231] mode=indexing
                      n439 = Enqueue Element(queue=w1233, element=w1231) -> (queue out=w1232:refnum<queue>)  [unwired: 2 in, 2 out]
                    }
                  }
                }
                n440 = Select(t=State_Type_Definitions,_for_0.26g_versions_and_later_2."True Stop" ("Enum"), s=w1214, f=State_Type_Definitions,_for_0.26g_versions_and_later_2."Task 6_B" ("Enum")) -> (s? t:f=w1219:T6)
              }
              frame "Exit" {
                # ">> State after true stop >>"
                # ">> Goes to true stop >>"
                n441 = for {
                  shift-right: [w1240] -> w1237
                  shift-left: w1234 -> [w1241]
                  tunnel: string[] ["STOP", "RESET ENCODERS", "RESET YAW", ""] -> [w1239] mode=indexing
                  n442 = Enqueue Element(queue=w1241, element=w1239) -> (queue out=w1240:refnum<queue>)  [unwired: 2 in, 2 out]
                }
              }
            }
          }
          frame 38 {
            # ">> Stepper height reeached >>"
            # ">>> yStepper command>>>"
            # ">> Manual override >>"
            n443 = Dequeue Element(queue=w1251, timeout in ms (-1)=w1246, error in (no error)=w1250) -> (element=w1254:T7)  [unwired: 3 out]
            n444 = Equal?(x=w1248, y=u8 60) -> (x = y?=w1252:bool)
            n445 = case shown="\"None\", Default" w1254 {
              tunnel: [w1265 State_Type_Definitions,_for_0.26g_versions_and_later_2."True Stop" ("Enum")] -> w1244
              tunnel: [w1263 w1280] -> w1243
              tunnel: w1247 -> [w1262 _]
              tunnel: w1249 -> [w1256 _]
              tunnel: [State_Type_Definitions,_for_0.26g_versions_and_later_2."Idle" ("Enum") State_Type_Definitions,_for_0.26g_versions_and_later_2."Shutdown" ("Enum")] -> w1245
              tunnel: w1252 -> [w1255 _]
              frame "None", Default {
                # ">> WIill proceed to part ii if not manual override >>"
                # ">>If ENABLE or Trigger is set to true>>"
                n446 = Or(x=w1255, y=w1256) -> (x .or. y?=w1257:bool)
                n447 = case shown="True" w1255 {
                  tunnel: [w1268 w1274] -> w1263
                  tunnel: w1262 -> [w1267 w1273]
                  frame False {
                    n448 = for {
                      shift-right: [w1270] -> w1268
                      shift-left: w1267 -> [w1271]
                      tunnel: string[] ["Z STEPPER CAM HEIGHT", "READ STEPPER VALUES"] ("element") -> [w1269] mode=indexing
                      n449 = Enqueue Element(queue=w1271, element=w1269) -> (queue out=w1270:refnum<queue>)  [unwired: 2 in, 2 out]
                    }
                  }
                  frame True {
                    n450 = for {
                      shift-right: [w1276] -> w1274
                      shift-left: w1273 -> [w1277]
                      tunnel: string[] ["ARDUINO - ULTRASONIC", "READ ULTRASONIC", "", "", "", ""] -> [w1275] mode=indexing
                      n451 = Enqueue Element(queue=w1277, element=w1275) -> (queue out=w1276:refnum<queue>)  [unwired: 2 in, 2 out]
                    }
                  }
                }
                n452 = Select(t=State_Type_Definitions,_for_0.26g_versions_and_later_2."True Stop" ("Enum"), s=w1256, f=State_Type_Definitions,_for_0.26g_versions_and_later_2."Task 9B: Rotate to Angle" ("Enum")) -> (s? t:f=w1259:T6)
                n453 = Select(t=w1259, s=w1257, f=State_Type_Definitions,_for_0.26g_versions_and_later_2."Task 9A: Raise Arm" ("Enum")) -> (s? t:f=w1265:T6)
              }
              frame "Exit" {
                n454 = for {
                  shift-right: [w1283] -> w1280
                  shift-left: _ -> [w1284]
                  tunnel: string[] ["STOP", "RESET ENCODERS", "RESET YAW", ""] -> [w1282] mode=indexing
                  n455 = Enqueue Element(queue=w1284, element=w1282) -> (queue out=w1283:refnum<queue>)  [unwired: 2 in, 2 out]
                }
              }
            }
          }
          frame 39 {
            # ">>> yStepper command>>>"
            n456 = Dequeue Element(queue=w1296, timeout in ms (-1)=w1295, error in (no error)=w1294) -> (element=w1298:T7)  [unwired: 3 out]
            n457 = In Range and Coerce(upper limit=305.0, x=w1288, lower limit=295.0) -> (In Range?=w1285:bool)  [unwired: 1 out]
            n458 = case shown="\"None\", Default" w1298 {
              tunnel: w1289 -> [w1301 _]
              tunnel: [w1309 State_Type_Definitions,_for_0.26g_versions_and_later_2."True Stop" ("Enum")] -> w1291
              tunnel: w1297 -> [w1307 w1325]
              tunnel: [w1306 w1324] -> w1290
              tunnel: [State_Type_Definitions,_for_0.26g_versions_and_later_2."Idle" ("Enum") State_Type_Definitions,_for_0.26g_versions_and_later_2."Shutdown" ("Enum")] -> w1292
              tunnel: w1285 -> [w1299 _]
              frame "None", Default {
                n459 = Or(x=w1299, y=w1301) -> (x .or. y?=w1300:bool)
                n460 = case shown="True" w1299 {
                  tunnel: w1307 -> [w1312 w1318]
                  tunnel: [w1311 w1316] -> w1306
                  frame False {
                    n461 = for {
                      shift-right: [w1314] -> w1311
                      shift-left: w1312 -> [w1315]
                      tunnel: string[] ["READ NAVX", "R-ACW"] ("element") -> [w1313] mode=indexing
                      n462 = Enqueue Element(queue=w1315, element=w1313) -> (queue out=w1314:refnum<queue>)  [unwired: 2 in, 2 out]
                    }
                  }
                  frame True {
                    n463 = for {
                      shift-right: [w1320] -> w1316
                      shift-left: w1318 -> [w1321]
                      tunnel: string[] ["STOP", "RESET ENCODERS", "RESET YAW", ""] -> [w1319] mode=indexing
                      n464 = Enqueue Element(queue=w1321, element=w1319) -> (queue out=w1320:refnum<queue>)  [unwired: 2 in, 2 out]
                    }
                  }
                }
                n465 = Select(t=State_Type_Definitions,_for_0.26g_versions_and_later_2."True Stop" ("Enum"), s=w1301, f=State_Type_Definitions."Task 9C: Rotation alignmnet") -> (s? t:f=w1303:u16)
                n466 = Select(t=w1303, s=w1300, f=State_Type_Definitions,_for_0.26g_versions_and_later_2."Task 9B: Rotate to Angle" ("Enum")) -> (s? t:f=w1309:u16)
              }
              frame "Exit" {
                n467 = for {
                  shift-right: [w1328] -> w1324
                  shift-left: w1325 -> [w1329]
                  tunnel: string[] ["STOP", "RESET ENCODERS", "RESET YAW", ""] -> [w1327] mode=indexing
                  n468 = Enqueue Element(queue=w1329, element=w1327) -> (queue out=w1328:refnum<queue>)  [unwired: 2 in, 2 out]
                }
              }
            }
          }
          frame 33 {
            # ">>> yStepper command>>>"
            n469 = Dequeue Element(queue=w1338, timeout in ms (-1)=w1337, error in (no error)=w1336) -> (element=w1339:T7)  [unwired: 3 out]
            n470 = case shown="\"None\", Default" w1339 {
              tunnel: w1334 -> [w1340 _]
              tunnel: [w1348 State_Type_Definitions,_for_0.26g_versions_and_later_2."True Stop" ("Enum")] -> w1331
              tunnel: w1335 -> [w1346 w1364]
              tunnel: [w1345 w1363] -> w1330
              tunnel: [State_Type_Definitions,_for_0.26g_versions_and_later_2."Idle" ("Enum") State_Type_Definitions,_for_0.26g_versions_and_later_2."Shutdown" ("Enum")] -> w1333
              frame "None", Default {
                n471 = case shown="True" w1340 {
                  tunnel: w1346 -> [w1351 w1357]
                  tunnel: [w1350 w1355] -> w1345
                  frame False {
                    n472 = for {
                      shift-right: [w1353] -> w1350
                      shift-left: w1351 -> [w1354]
                      tunnel: string[] ["READ IR", "FORWARD - IR ASSIST"] ("element") -> [w1352] mode=indexing
                      n473 = Enqueue Element(queue=w1354, element=w1352) -> (queue out=w1353:refnum<queue>)  [unwired: 2 in, 2 out]
                    }
                  }
                  frame True {
                    n474 = for {
                      shift-right: [w1359] -> w1355
                      shift-left: w1357 -> [w1360]
                      tunnel: string[] ["STOP", "RESET ENCODERS", "RESET YAW", ""] -> [w1358] mode=indexing
                      n475 = Enqueue Element(queue=w1360, element=w1358) -> (queue out=w1359:refnum<queue>)  [unwired: 2 in, 2 out]
                    }
                  }
                }
                n476 = Select(t=State_Type_Definitions,_for_0.26g_versions_and_later_2."True Stop" ("Enum"), s=w1340, f=State_Type_Definitions,_for_0.26g_versions_and_later_2."True Stop") -> (s? t:f=w1342:T6)
                n477 = Select(t=w1342, s=w1340, f=State_Type_Definitions."Task 9C: Rotation alignmnet" ("Enum")) -> (s? t:f=w1348:u16)
              }
              frame "Exit" {
                n478 = for {
                  shift-right: [w1367] -> w1363
                  shift-left: w1364 -> [w1368]
                  tunnel: string[] ["STOP", "RESET ENCODERS", "RESET YAW", ""] -> [w1366] mode=indexing
                  n479 = Enqueue Element(queue=w1368, element=w1366) -> (queue out=w1367:refnum<queue>)  [unwired: 2 in, 2 out]
                }
              }
            }
          }
          frame 27 {
            # ">>> yStepper command>>>"
            # ">> Manual override >>"
            n480 = Dequeue Element(queue=w1377, timeout in ms (-1)=w1376, error in (no error)=w1378) -> (element=w1375:T7)  [unwired: 3 out]
            n481 = Equal?(x=w1374, y=u8 60) -> (x = y?=w1372:bool)
            n482 = case shown="\"None\", Default" w1375 {
              tunnel: [w1388 State_Type_Definitions,_for_0.26g_versions_and_later_2."True Stop" ("Enum")] -> w1379
              tunnel: [w1391 w1408] -> w1380
              tunnel: [State_Type_Definitions,_for_0.26g_versions_and_later_2."Idle" ("Enum") State_Type_Definitions,_for_0.26g_versions_and_later_2."Shutdown" ("Enum")] -> w1381
              tunnel: w1372 -> [w1387 _]
              tunnel: w1371 -> [w1386 _]
              tunnel: w1370 -> [w1382 w1405]
              frame "None", Default {
                # "Stays in Task 5_A until stepper reaches desired \nheight"
                # "T: Go back to idle, F: Continue with task\""
                # ">> Manual override >>"
                n483 = case shown="True" w1387 {
                  tunnel: [w1395 w1401] -> w1391
                  tunnel: w1382 -> [w1393 w1399]
                  frame False {
                    n484 = for {
                      tunnel: string[] ["Z STEPPER CAM HEIGHT", "READ STEPPER VALUES"] ("element") -> [w1396] mode=indexing
                      shift-right: [w1398] -> w1395
                      shift-left: w1393 -> [w1397]
                      n485 = Enqueue Element(queue=w1397, element=w1396) -> (queue out=w1398:refnum<queue>)  [unwired: 2 in, 2 out]
                    }
                  }
                  frame True {
                    n486 = for {
                      shift-right: [w1403] -> w1401
                      shift-left: w1399 -> [w1404]
                      tunnel: string[] ["ARDUINO - ULTRASONIC", "READ ULTRASONIC", ""] -> [w1402] mode=indexing
                      n487 = Enqueue Element(queue=w1404, element=w1402) -> (queue out=w1403:refnum<queue>)  [unwired: 2 in, 2 out]
                    }
                  }
                }
                n488 = Or(x=w1387, y=w1386) -> (x .or. y?=w1389:bool)
                n489 = Select(t=State_Type_Definitions,_for_0.26g_versions_and_later_2."True Stop" ("Enum"), s=w1386, f=State_Type_Definitions,_for_0.26g_versions_and_later_2."Task 8B: MOVE TO BOX" ("Enum")) -> (s? t:f=w1383:T6)
                n490 = Select(t=w1383, s=w1389, f=State_Type_Definitions,_for_0.26g_versions_and_later_2."Task 8A: RAISE ARM" ("Enum")) -> (s? t:f=w1388:T6)
              }
              frame "Exit" {
                n491 = for {
                  shift-right: [w1411] -> w1408
                  shift-left: w1405 -> [w1412]
                  tunnel: string[] ["STOP", "RESET ENCODERS", "RESET YAW", "ARDUINO MODE 0"] -> [w1410] mode=indexing
                  n492 = Enqueue Element(queue=w1412, element=w1410) -> (queue out=w1411:refnum<queue>)  [unwired: 2 in, 2 out]
                }
              }
            }
          }
          frame 28 {
            w1418 = u8 20 ("y")
            # ">>> yStepper command>>>"
            n493 = Less?(x=w1415, y=w1418) -> (x < y?=w1416:bool)
            n494 = Dequeue Element(queue=w1422, timeout in ms (-1)=w1421, error in (no error)=w1423) -> (element=w1420:T7)  [unwired: 3 out]
            n495 = Less?(x=w1414, y=w1418) -> (x < y?=w1417:bool)
            n496 = And(x=w1417, y=w1416) -> (x .and. y?=w1413:bool)
            n497 = case shown="\"None\", Default" w1420 {
              tunnel: [w1435 State_Type_Definitions,_for_0.26g_versions_and_later_2."True Stop" ("Enum")] -> w1425
              tunnel: [w1438 w1455] -> w1424
              tunnel: [State_Type_Definitions,_for_0.26g_versions_and_later_2."Idle" ("Enum") State_Type_Definitions,_for_0.26g_versions_and_later_2."Shutdown" ("Enum")] -> w1426
              tunnel: w1428 -> [w1434 _]
              tunnel: w1427 -> [w1430 w1452]
              tunnel: w1413 -> [w1429 _]
              frame "None", Default {
                # "Stays in Task 5_B to capture image over 5 seconds"
                # "T: Go back to idle, F: Continue with task\""
                # ">> Manual override >>"
                n498 = case shown="True" w1429 {
                  tunnel: [w1442 w1448] -> w1438
                  tunnel: w1430 -> [w1440 w1446]
                  frame False {
                    n499 = for {
                      tunnel: string[] ["FORWARD", "READ ULTRASONIC", "READ NAVX"] ("element") -> [w1443] mode=indexing
                      shift-right: [w1445] -> w1442
                      shift-left: w1440 -> [w1444]
                      n500 = Enqueue Element(queue=w1444, element=w1443) -> (queue out=w1445:refnum<queue>)  [unwired: 2 in, 2 out]
                    }
                  }
                  frame True {
                    n501 = for {
                      shift-right: [w1450] -> w1448
                      shift-left: w1446 -> [w1451]
                      tunnel: string[] ["STOP", "RESET ENCODERS", "OPEN LOG CAM", "SET TIMER 5"] -> [w1449] mode=indexing
                      n502 = Enqueue Element(queue=w1451, element=w1449) -> (queue out=w1450:refnum<queue>)  [unwired: 2 in, 2 out]
                    }
                  }
                }
                n503 = Or(x=w1429, y=w1434) -> (x .or. y?=w1436:bool)
                n504 = Select(t=State_Type_Definitions,_for_0.26g_versions_and_later_2."True Stop" ("Enum"), s=w1434, f=State_Type_Definitions,_for_0.26g_versions_and_later_2."Task 8C: CAM BURST" ("Enum")) -> (s? t:f=w1431:T6)
                n505 = Select(t=w1431, s=w1436, f=State_Type_Definitions,_for_0.26g_versions_and_later_2."Task 8B: MOVE TO BOX" ("Enum")) -> (s? t:f=w1435:T6)
              }
              frame "Exit" {
                n506 = for {
                  shift-right: [w1458] -> w1455
                  shift-left: w1452 -> [w1459]
                  tunnel: string[] ["STOP", "RESET ENCODERS", "RESET YAW", "ARDUINO MODE 0"] -> [w1457] mode=indexing
                  n507 = Enqueue Element(queue=w1459, element=w1457) -> (queue out=w1458:refnum<queue>)  [unwired: 2 in, 2 out]
                }
              }
            }
          }
          frame 29 {
            # ">>> yStepper command>>>"
            # ">> Manual override >>"
            n508 = Dequeue Element(queue=w1468, timeout in ms (-1)=w1467, error in (no error)=w1466) -> (element=w1465:T7)  [unwired: 3 out]
            n509 = case shown="\"None\", Default" w1465 {
              tunnel: [w1477 State_Type_Definitions,_for_0.26g_versions_and_later_2."True Stop" ("Enum")] -> w1470
              tunnel: [w1480 w1497] -> w1463
              tunnel: [State_Type_Definitions,_for_0.26g_versions_and_later_2."Idle" ("Enum") State_Type_Definitions,_for_0.26g_versions_and_later_2."Shutdown" ("Enum")] -> w1462
              tunnel: w1464 -> [w1471 _]
              tunnel: w1469 -> [w1476 w1494]
              tunnel: w1460 -> [w1475 _]
              frame "None", Default {
                # ">> Is time up? >>"
                # "Determines if object is in range to pick up"
                # ">> Manual override >>"
                n510 = case shown="True" w1475 {
                  tunnel: [w1484 w1490] -> w1480
                  tunnel: w1476 -> [w1482 w1488]
                  frame False {
                    n511 = for {
                      tunnel: string[] ["CAM ACQ", "START TIMER"] ("element") -> [w1485] mode=indexing
                      shift-right: [w1487] -> w1484
                      shift-left: w1482 -> [w1486]
                      n512 = Enqueue Element(queue=w1486, element=w1485) -> (queue out=w1487:refnum<queue>)  [unwired: 2 in, 2 out]
                    }
                  }
                  frame True {
                    n513 = for {
                      shift-right: [w1492] -> w1490
                      shift-left: w1488 -> [w1493]
                      tunnel: string[] ["CAM CLOSE", "PROCESS IMAGE", "SET TIMER 5"] -> [w1491] mode=indexing
                      n514 = Enqueue Element(queue=w1493, element=w1491) -> (queue out=w1492:refnum<queue>)  [unwired: 2 in, 2 out]
                    }
                  }
                }
                n515 = Or(x=w1475, y=w1471) -> (x .or. y?=w1478:bool)
                n516 = Select(t=State_Type_Definitions,_for_0.26g_versions_and_later_2."True Stop" ("Enum"), s=w1471, f=State_Type_Definitions,_for_0.26g_versions_and_later_2."Task 8D: PROCESS IMAGE" ("Enum")) -> (s? t:f=w1473:T6)
                n517 = Select(t=w1473, s=w1478, f=State_Type_Definitions,_for_0.26g_versions_and_later_2."Task 8C: CAM BURST" ("Enum")) -> (s? t:f=w1477:T6)
              }
              frame "Exit" {
                n518 = for {
                  shift-right: [w1500] -> w1497
                  shift-left: w1494 -> [w1501]
                  tunnel: string[] ["STOP", "RESET ENCODERS", "RESET YAW", "ARDUINO MODE 0"] -> [w1499] mode=indexing
                  n519 = Enqueue Element(queue=w1501, element=w1499) -> (queue out=w1500:refnum<queue>)  [unwired: 2 in, 2 out]
                }
              }
            }
          }
          frame 30 {
            # ">>> yStepper command>>>"
            n520 = Dequeue Element(queue=w1507, timeout in ms (-1)=w1506, error in (no error)=w1505) -> (element=w1504:T7)  [unwired: 3 out]
            n521 = case shown="\"None\", Default" w1504 {
              tunnel: [w1519 State_Type_Definitions,_for_0.26g_versions_and_later_2."True Stop" ("Enum")] -> w1511
              tunnel: [w1522 w1539] -> w1510
              tunnel: [State_Type_Definitions,_for_0.26g_versions_and_later_2."Idle" ("Enum") State_Type_Definitions,_for_0.26g_versions_and_later_2."Shutdown" ("Enum")] -> w1512
              tunnel: w1508 -> [w1518 _]
              tunnel: w1509 -> [w1514 w1536]
              tunnel: w1502 -> [w1513 _]
              frame "None", Default {
                # ">> T: Breaks out of state loop; F: Stays in loop>>"
                # ">> Manual override >>"
                # ">> Checks if time is up>>"
                # "Stays in Task 5D until the object is detected"
                # "T: Go back to idle, F: Continue with task\""
                # ">> Manual override >>"
                n522 = case shown="True" w1513 {
                  tunnel: [w1526 w1532] -> w1522
                  tunnel: w1514 -> [w1524 w1530]
                  frame False {
                    n523 = for {
                      tunnel: string[] ["START TIMER", "PROCESS IMAGE", ""] ("element") -> [w1527] mode=indexing
                      shift-right: [w1529] -> w1526
                      shift-left: w1524 -> [w1528]
                      n524 = Enqueue Element(queue=w1528, element=w1527) -> (queue out=w1529:refnum<queue>)  [unwired: 2 in, 2 out]
                    }
                  }
                  frame True {
                    n525 = for {
                      shift-right: [w1534] -> w1532
                      shift-left: w1530 -> [w1535]
                      tunnel: string[] ["CAM CLOSE", "RESET ENCODERS", ""] -> [w1533] mode=indexing
                      n526 = Enqueue Element(queue=w1535, element=w1533) -> (queue out=w1534:refnum<queue>)  [unwired: 2 in, 2 out]
                    }
                  }
                }
                n527 = Or(x=w1513, y=w1518) -> (x .or. y?=w1520:bool)
                n528 = Select(t=State_Type_Definitions,_for_0.26g_versions_and_later_2."True Stop" ("Enum"), s=w1518, f=State_Type_Definitions,_for_0.26g_versions_and_later_2."Task 8E: ROBOT ADJUST" ("Enum")) -> (s? t:f=w1515:T6)
                n529 = Select(t=w1515, s=w1520, f=State_Type_Definitions,_for_0.26g_versions_and_later_2."Task 8D: PROCESS IMAGE" ("Enum")) -> (s? t:f=w1519:T6)
              }
              frame "Exit" {
                n530 = for {
                  shift-right: [w1542] -> w1539
                  shift-left: w1536 -> [w1543]
                  tunnel: string[] ["STOP", "RESET ENCODERS", "RESET YAW", "ARDUINO MODE 0"] -> [w1541] mode=indexing
                  n531 = Enqueue Element(queue=w1543, element=w1541) -> (queue out=w1542:refnum<queue>)  [unwired: 2 in, 2 out]
                }
              }
            }
          }
          frame 31 {
            # ">>> yStepper command>>>"
            n532 = Dequeue Element(queue=w1554, timeout in ms (-1)=w1553, error in (no error)=w1552) -> (element=w1551:T7)  [unwired: 3 out]
            n533 = Subtract(x=w1549, y=300.0) -> (x-y=w1547:dbl)
            n534 = formula code="if (error >= -20 && error <= 20)\ndistance = 0;\n\nelse if (error >= 21 && error <= 40)\ndistance = 10;\n\nelse if (error >= 41)\ndistance = 20;"("error"=w1547) -> ("distance"=w1545:dbl)
            n535 = Greater Or Equal?(x=w1546, y=w1545) -> (x >= y?=w1544:bool)
            n536 = case shown="\"None\", Default" w1551 {
              tunnel: [w1566 State_Type_Definitions,_for_0.26g_versions_and_later_2."True Stop" ("Enum")] -> w1558
              tunnel: [w1569 w1586] -> w1557
              tunnel: [State_Type_Definitions,_for_0.26g_versions_and_later_2."Idle" ("Enum") State_Type_Definitions,_for_0.26g_versions_and_later_2."Shutdown" ("Enum")] -> w1559
              tunnel: w1555 -> [w1565 _]
              tunnel: w1556 -> [w1561 w1583]
              tunnel: w1544 -> [w1560 _]
              frame "None", Default {
                # ">> T: Breaks out of state loop; F: Stays in loop>>"
                # ">> Manual override >>"
                # ">> Checks if time is up>>"
                # "Stays in Task 5D until the object is detected"
                # "T: Go back to idle, F: Continue with task\""
                # ">> Manual override >>"
                n537 = case shown="False" w1560 {
                  tunnel: [w1573 w1579] -> w1569
                  tunnel: w1561 -> [w1571 w1577]
                  frame False {
                    n538 = for {
                      tunnel: string[] ["RIGHT - SLOW", "READ ENCODERS", "READ YAW"] ("element") -> [w1574] mode=indexing
                      shift-right: [w1576] -> w1573
                      shift-left: w1571 -> [w1575]
                      n539 = Enqueue Element(queue=w1575, element=w1574) -> (queue out=w1576:refnum<queue>)  [unwired: 2 in, 2 out]
                    }
                  }
                  frame True {
                    n540 = for {
                      shift-right: [w1581] -> w1579
                      shift-left: w1577 -> [w1582]
                      tunnel: string[] ["CAM CLOSE", "", ""] -> [w1580] mode=indexing
                      n541 = Enqueue Element(queue=w1582, element=w1580) -> (queue out=w1581:refnum<queue>)  [unwired: 2 in, 2 out]
                    }
                  }
                }
                n542 = Or(x=w1560, y=w1565) -> (x .or. y?=w1567:bool)
                n543 = Select(t=State_Type_Definitions,_for_0.26g_versions_and_later_2."True Stop" ("Enum"), s=w1565, f=State_Type_Definitions,_for_0.26g_versions_and_later_2."True Stop" ("Enum")) -> (s? t:f=w1562:T6)
                n544 = Select(t=w1562, s=w1567, f=State_Type_Definitions,_for_0.26g_versions_and_later_2."Task 8E: ROBOT ADJUST" ("Enum")) -> (s? t:f=w1566:T6)
              }
              frame "Exit" {
                n545 = for {
                  shift-right: [w1589] -> w1586
                  shift-left: w1583 -> [w1590]
                  tunnel: string[] ["STOP", "RESET ENCODERS", "RESET YAW", "ARDUINO MODE 0"] -> [w1588] mode=indexing
                  n546 = Enqueue Element(queue=w1590, element=w1588) -> (queue out=w1589:refnum<queue>)  [unwired: 2 in, 2 out]
                }
              }
            }
          }
        }
      }
    }
    n547 = local write "Green LED"(w198) -> ()
  }
  n548 = call <vilib>:"DIO Close.vi"("error in (no error)"=w23, "DIO Info In"=w26) -> ()  [unwired: 9 in, 1 out]
  n549 = call <vilib>:"DIO Close.vi"("error in (no error)"=w33, "DIO Info In"=w35) -> ()  [unwired: 9 in, 1 out]
  n550 = call <vilib>:"NavX Close.vi"("error in (no error)"=w7, "NavX Info In"=w6) -> ()  [unwired: 9 in, 1 out]
  n551 = call <vilib>:"DIO Close.vi"("error in (no error)"=w28, "DIO Info In"=w30) -> ()  [unwired: 9 in, 1 out]
  n552 = call <vilib>:"DIO Close.vi"("error in (no error)"=w14, "DIO Info In"=w15) -> ()  [unwired: 9 in, 1 out]
  n553 = call <vilib>:"DIO Close.vi"("error in (no error)"=w9, "DIO Info In"=w10) -> ()  [unwired: 9 in, 1 out]
  n554 = while {
    stop <- w2150 stop-if-true
    n555 = call <vilib>:"RT Get CPU Loads.vi"() -> ("CPU loads"=→"CPU loads":T5[])  [unwired: 10 in, 1 out]
    n556 = Wait (ms)(milliseconds to wait=u32 100) -> ()  [unwired: 1 out]
    n557 = call "FGV Stop.vi"("Init/Read/Write State"=States_for_Action_Engine."Read") -> ("Output node"=w2150:bool)  [unwired: 2 in, 1 out]
  }
  n558 = while {
    stop <- w2154 stop-if-true
    n559 = call "MOTOR CONTROL WITH PID AE.vi"("AE Mode"=MOTOR_CONTROL_WITH_PID_AE_DATA_MODE_TYPE_DEF."Read from AE") -> ("Speed & distance"=→"Speed & distance":T1)  [unwired: 3 in]
    n560 = call "FGV Stop.vi"("Init/Read/Write State"=States_for_Action_Engine."Read") -> ("Output node"=w2154:bool)  [unwired: 2 in, 1 out]
    n561 = Wait (ms)(milliseconds to wait=u32 5) -> ()  [unwired: 1 out]
  }
  n562 = Merge Errors "Merge Errors"(w63, w62) -> (w45:errorcluster)
  n563 = Merge Errors(w49, w45) -> (w44:errorcluster)
  n564 = Destroy User Event(user event=w66, error in=w44) -> ()  [unwired: 1 out]
  n565 = Destroy User Event(user event=w67, error in=w44) -> ()  [unwired: 1 out]
  n566 = Unregister For Events(event registration refnum=w58, error in=w44) -> ()  [unwired: 1 out]
  n567 = Release Queue(queue=w40, error in (no error)=w44) -> (error out=→"error out":errorcluster)  [unwired: 1 in, 2 out]
  n568 = Release Queue(queue=w57, error in (no error)=w44) -> ()  [unwired: 1 in, 3 out]
